vi "Main_Marvin.vi"() -> ()   [LabVIEW 2017]
uses:
  PCAN_Driver/ControlCAN.llb/DevType.ctl
  PCAN_Driver/ControlCAN.llb/CAN Channel.ctl
  PCAN_Driver/ControlCAN.llb/VCI_INIT_CONFIG.ctl
  PCAN_Driver/ControlCAN.llb/InitFlag.ctl
  PCAN_Driver/ControlCAN.llb/Fliter.ctl
  PCAN_Driver/ControlCAN.llb/Mode.ctl
  <vilib>/Utility/miscctls.llb/LVRowAndColumnTypeDef.ctl
  <vilib>/Utility/config.llb/Read Key (String).vi
  <vilib>/Utility/config.llb/Write Key (String).vi
  <vilib>/Utility/cursorutil.llb/Set Cursor (Icon Pict).vi
  PCAN_Driver/ControlCAN.lvlib
  <vilib>/Utility/config.llb/NI_LVConfig.lvlib
panel:
  in  "Index":string="5"
  out "Automation":bool
  out "ClosePanel 2":bool=TRUE
  out "ClosePanel":bool=TRUE
  out "Next SN":string
  out "Curret SN":string
  out "Array 5":dbl[](array[numeric])
  out "Array 4":dbl[](array[numeric])
  out "VC1500-2 Vel":dbl
  out "VC15100-1 Vel":dbl
  out "Array Test":T1(array[ring])
  out "TempAlg":bool=TRUE
  out "f":T2(ring)=enum."Empty"
  out "VC15100-2":dbl
  out "VC15100-1 Cur":dbl
  out "Auxiind":bool
  out "TempSensCalind":bool
  out "VisualInspectionResult":bool
  out "Burninind":bool
  out "TempControlind":bool
  out "MotorTempind":bool
  out "SpeedStopind":bool
  out "EnableTestind":bool
  out "ComTestind":bool
  out "SoftwareVer":string
  in  "SetSN":bool
  out "CurrentOffset":dbl
  out "Array 3":string[](array[string])
  out "Cal Value":string
  in  "Stop Burn-in":bool
  out "Array 2":dbl[](array[numeric])
  out "VISA resource name out":refnum<visa-resource-name>
  out "UUT":u8
  out "CAN Status":bool
  in  "Channel 2":T3 caption="Channel" items=["Channel 1", "Channel 2"]
  out "Config_CANAT":T9 {"DevType" items=["USB-CAN"=3, "USB-CAN2"=4]; "CanIndex" items=["通道1", "通道2"]; "VCI_INIT_CONFIG"."Fliter" items=["接收所有类型"=3, "只接收标准帧"=4, "只接收扩展帧"=7]; "VCI_INIT_CONFIG"."Mode" items=["正常工作", "自测模式（环回）", "仅侦听模式"]; "VCI_INIT_CONFIG"."InitFlag" items=["使用Flash参数", "使用界面设置参数"]}
  out "Array":u64[][](array[numeric]) format="%016x"
  out "Motor Phase Current RMS":dbl
  out "Ambient Temperature":dbl
  out "Speed error":bool
  out "Commutation err":bool
  out "Under voltage/Over voltage":bool
  out "Derated drive temp":bool
  out "Motor Over temperature":bool
  out "Motor Sensor temp Fauilre":bool
  out "Drive Over temperature":bool
  out "Drive Sensor temp Failure":bool
  out "Ambient Over temp":bool
  out "Ambient Sensor temp":bool
  out "DC Voltage":dbl
  out "DC Current":dbl
  out "Power transistor Heat sink Temp.":dbl
  out "Motor Stator Temp.":dbl
  out "Motor Speed RPM":dbl
  out "ECS State":u16
  out "Waveform Chart":dbl[](graph)
  out "UUT":string="EBAY"
  in  "Logger Path":path
  in  "Report":bool
  in  "Start":bool
  in  "ATR":string[][](table)=[["Test Communication", "-", "-", "-", "-", ""], ["Set S/N", "-", "-", "-", "-", ""], ["Set Board Number", "-", "-", "-", "-", ""], [" ", "", "", "", "", ""], ["Test Communication", "-", "-", "-", "-", ""], ["Get S/N", "-", "-", "-", "", ""], ["Get Board Number", "-", "-", "-", "", ""], ["Get FW", "-", "-", "-", "", ""], ["Enable Motor", "", "", "", "", ""], ["Small position command", "", "", "", "", ""], ["Measure delta", "", "", "", "", ""], ["Velocity command", "", "", "", "", ""]]
  in  "Settings":bool
  in  "Refresh Button":bool
  out "Serial":bool
  in  "VISA resource name":refnum<visa-resource-name>="COM6"
  in  "Serial Com":bool
  in  "Help Button":bool
  out "Pannel User Message":string
  in  "Stop Button":bool
  # "Marvin"
  # "REDLER TECHNOLOGIES LTD"
  # "ver 1.2g"
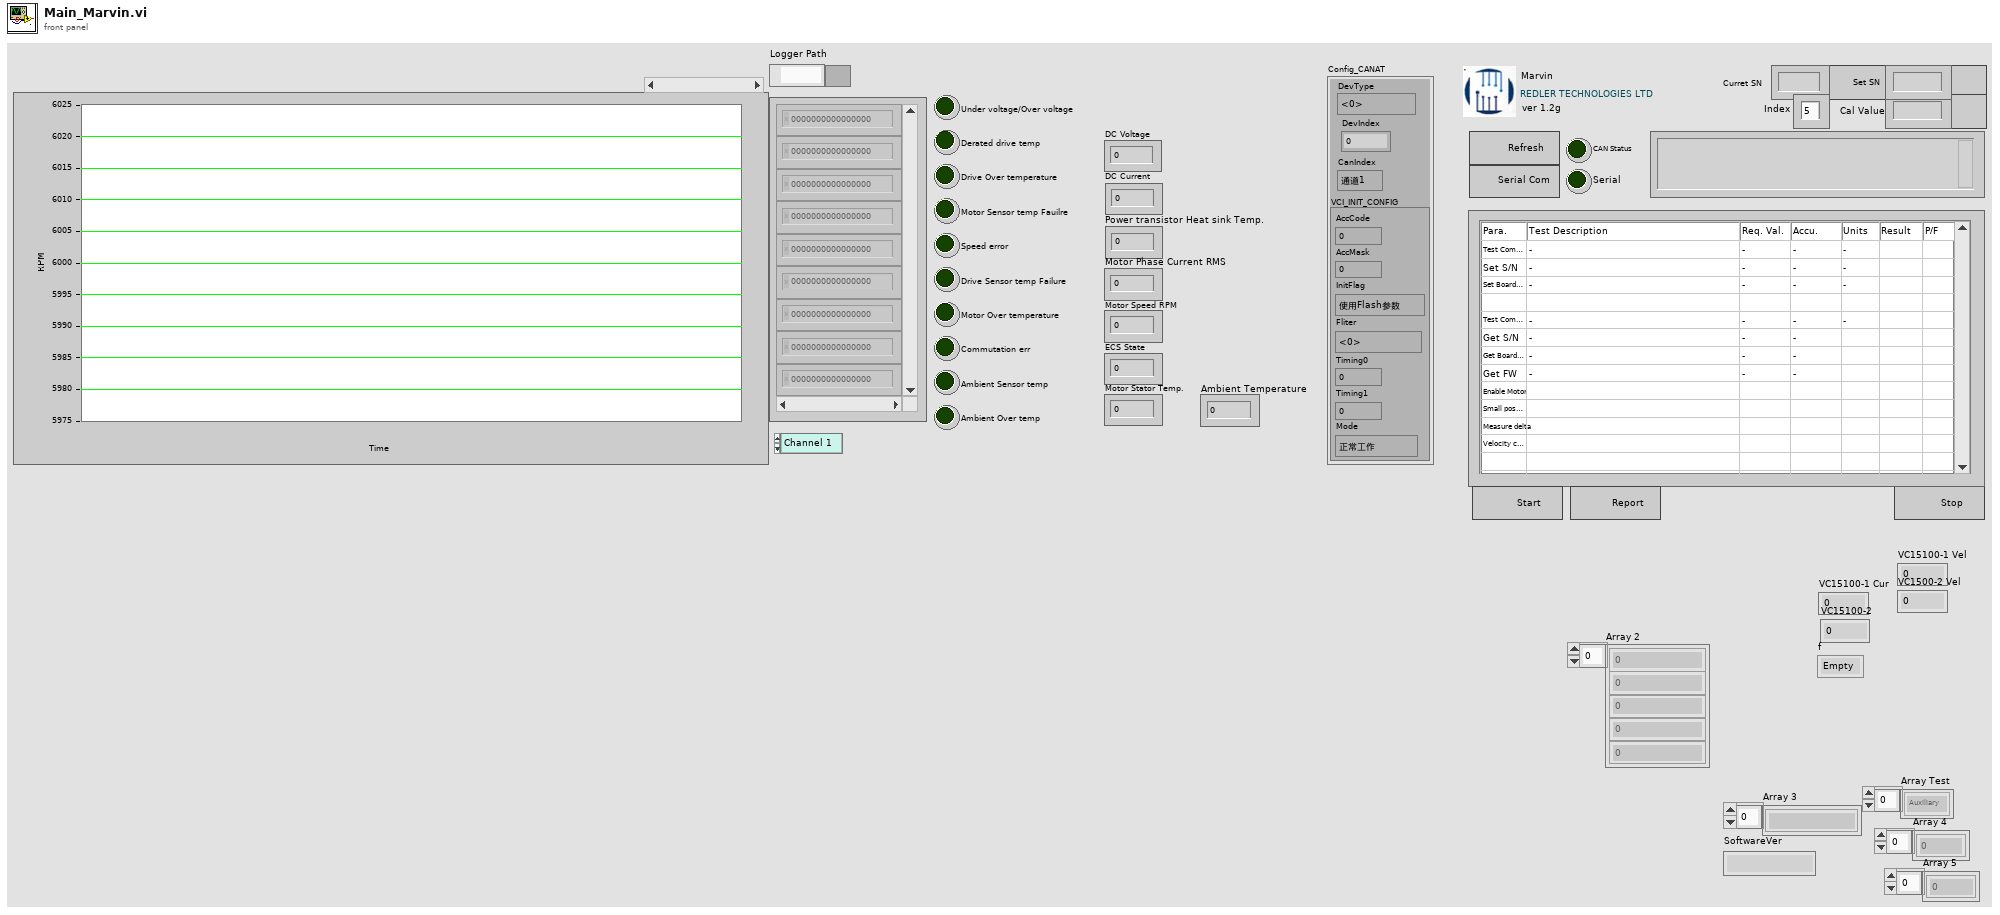
[diagram p1: front panel]
types:
  T1 = enum16{"Auxiliary", "Temp Sens Cal", "Com Test", "Enable Test", "Speed Command", "Stop Time", "Temp Control", "Burn in", "Visual Inspec", "Empty"}[]
  T2 = enum16{"Auxiliary", "Temp Sens Cal", "Com Test", "Enable Test", "Speed Command", "Stop Time", "Temp Control", "Burn in", "Visual Inspec", "Empty"}
  T3 = typedef "ControlCAN.lvlib/CAN Channel.ctl" = u32
  T4 = typedef "ControlCAN.lvlib/DevType.ctl" = u32
  T5 = typedef "ControlCAN.lvlib/VCI_INIT_CONFIG.ctl" = cluster{"AccCode":u32, "AccMask":u32, "InitFlag":T6, "Fliter":T7, "Timing0":u8, "Timing1":u8, "Mode":T8}
  T6 = typedef "ControlCAN.lvlib/InitFlag.ctl" = u32
  T7 = typedef "ControlCAN.lvlib/Fliter.ctl" = u8
  T8 = typedef "ControlCAN.lvlib/Mode.ctl" = u8
  T9 = cluster{"DevType":T4, "DevIndex":u32, "CanIndex":T3, "VCI_INIT_CONFIG":T5}
  T10 = cluster{"VISA":refnum<visa-resource-name>, "Array Test":enum16{"Auxiliary", "Temp Sens Cal", "Com Test", "Enable Test", "Speed Command", "Stop Time", "Temp Control", "Burn in", "Visual Inspec", "Empty"}[]}
  T11 = cluster{"ID":u32, "MSGTYPE":u8, "LEN":u8, "aDATA":u8[]}[]
  T12 = enum16{"Erase ATR Table", "Stop", "MainProgram", "Initialize"}
  T13 = enum8{"Enabled", "Disabled", "Disabled and Grayed Out"}
  T14 = cluster{"ID":u32, "MSGTYPE":u8, "LEN":u8, "aDATA":u8[]}
  T15 = typedef "NI_LVConfig.lvlib/Config Data RefNum.ctl" = refnum<k1>
  T16 = enum16{"STOP", "VC15100-2", "RESET", "VC15100-1", "MD0"}
  T17 = typedef "LVRowAndColumnTypeDef.ctl" = cluster{"Row":i32, "Column":i32}
  T18 = enum32{"Invalid", "Standard", "Closed", "Hidden", "Minimized", "Maximized"}
  T19 = enum16{"End", "Start", "Verify VR", "Verify UUT"}
  T20 = enum16{"open", "replace", "create", "open or create", "replace or create", "replace or create with confirmation"}
  T21 = typedef "ControlCAN.lvlib/VCI_CAN_OBJ.ctl" = cluster{"ID":u32, "TimeStamp":u32, "TimeFlag":u8, "SendType":u8, "RemoteFlag":u8, "ExternFlag":u8, "DataLen":u8, "Data":u8[], "Reserved":u8[]}
  T22 = cluster{"Type":enum16{"接收", "发送"}, "Channel":T3, "Time":timestamp, "VCI_CAN_OBJ":T21}[]
  T23 = cluster{"Type":enum16{"接收", "发送"}, "Channel":T3, "Time":timestamp, "VCI_CAN_OBJ":T21}
  T24 = typedef "LVPoint32TypeDef.ctl" = cluster{"Horizontal":i32, "Vertical":i32}
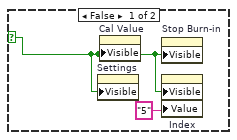
[diagram p3: hidden frame]
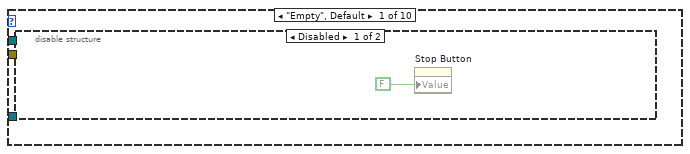
[diagram p6: hidden frame]
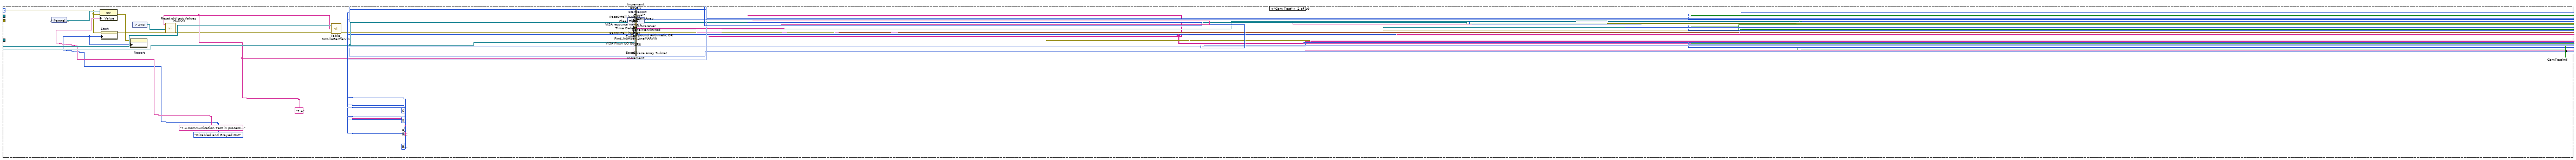
[diagram p8: hidden frame]
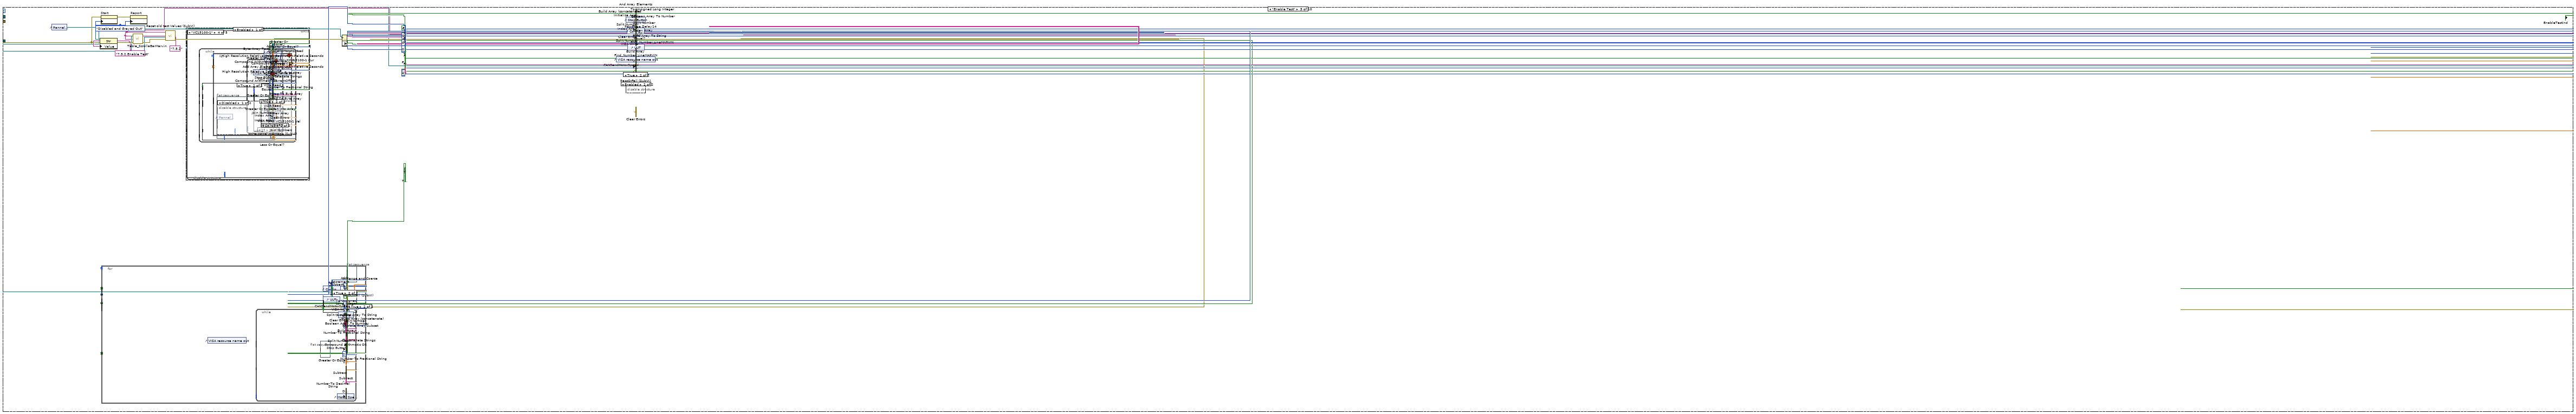
[diagram p9: hidden frame]
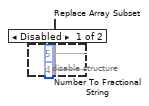
[diagram p11: hidden frame]
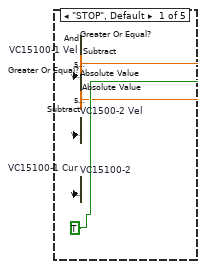
[diagram p12: hidden frame]
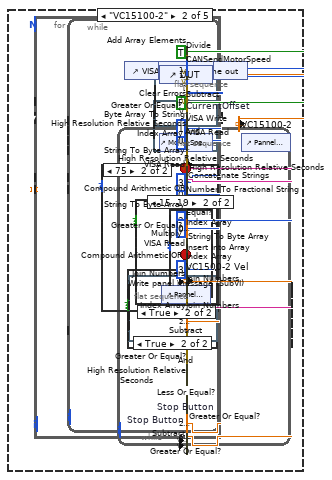
[diagram p13: hidden frame]
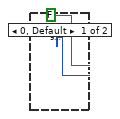
[diagram p14: hidden frame]
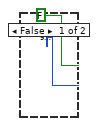
[diagram p15: hidden frame]
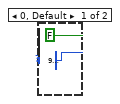
[diagram p16: hidden frame]
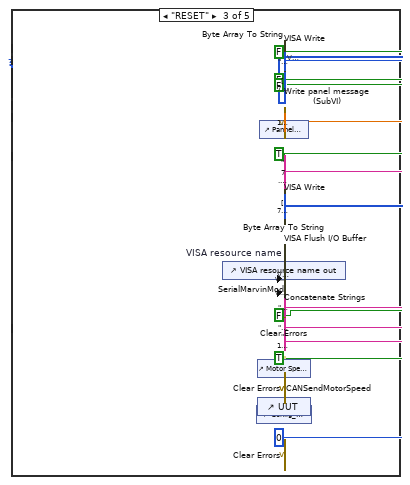
[diagram p18: hidden frame]
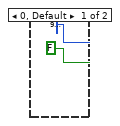
[diagram p19: hidden frame]
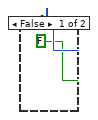
[diagram p20: hidden frame]
diagram:
  w1 = FALSE ("ClosePanel")
  w2 = "0" ("Next SN")
  w7 = 0.0 ("Val")
  (unwired) "[Marvin]\nEBAY Software Version = \"5.3.9\"\nAHU Software Version = \"5.3.8d\"\nEBAY Serial Number = \"0\"\nAHU Serial Number = \"0\""
  w21 = errorcluster {"status"=FALSE, "code"=0, "source"=""} ("error in (no error)")
  n1 = disable-structure shown="Disabled" {
    frame Disabled {
      n2 = case shown="\" float\"" {
        selector: _ -> [_ _]
        tunnel: [u32 0 ("Data I") w30] -> _
        frame "Int", Default {
        }
        frame " float" {
          n3 = To Single Precision Float(number=sgl 0.0 ("Data F")) -> (single precision float=w32:sgl)
          n4 = call "Int_Float.vi"("1 Float in"=w32) -> ("1 Int out"=w31:i32)  [unwired: 1 in, 1 out]
          n5 = To Unsigned Long Integer(number=w31) -> (unsigned 32bit integer=w30:u32)
        }
      }
    }
    frame Enabled {
    }
  }
  n6 = disable-structure shown="Disabled" {
    frame Disabled {
    }
    frame Enabled {
    }
  }
  n7 = disable-structure shown="Disabled" {
    frame Disabled {
      w35 = T13."Disabled and Grayed Out" ("Disabled")
      w36 = T13."Enabled" ("Disabled")
      n8 = control-ref of="Stop Button"() -> ()  [unwired: 1 out]
      n9 = control-ref of="Config_CANAT"() -> ()  [unwired: 1 out]
      n10 = control-ref of="UUT"() -> ()  [unwired: 1 out]
      n11 = control-ref of="Motor Speed RPM"() -> ()  [unwired: 1 out]
      n12 = control-ref of="Pannel User Message"() -> ()  [unwired: 1 out]
      n13 = control-ref of="ATR"() -> (w33:refnum<vi>)
      n14 = call "Reset old test Values (SubVI).vi"("Atr in"=w33) -> ()  [unwired: 10 in, 1 out]
      n15 = property on="Stop Button" class="Bool (strict)" props=["Value"]() -> ()  [unwired: 2 in, 3 out]
      n16 = property on="Start" class="Bool (strict)"("DisabledEnum"=w35) -> (error out=w34:errorcluster)  [unwired: 2 in, 1 out]
      n17 = property on="Start" class="Bool (strict)"("DisabledEnum"=w36) -> (error out=w37:errorcluster)  [unwired: 2 in, 1 out]
      n18 = property on="Report" class="Bool (strict)"(error in=w34, "DisabledEnum"=w35) -> ()  [unwired: 1 in, 2 out]
      n19 = property on="Report" class="Bool (strict)"(error in=w37, "DisabledEnum"=w36) -> ()  [unwired: 1 in, 2 out]
    }
    frame Enabled {
    }
  }
  n20 = disable-structure shown="Disabled" {
    frame Disabled {
      n21 = control-ref of="Pannel User Message"() -> (w38:refnum<vi>)
      n22 = call "Write panel message (SubVI).vi"("Time to wait"=30.0, "String in"=w38) -> ()  [unwired: 9 in, 1 out]
    }
    frame Enabled {
    }
  }
  n23 = disable-structure shown="Disabled" {
    frame Disabled {
      (unwired) 0.5 ("Delay Time (sec)")
      n24 = call <vilib>:"Unset Busy.vi"() -> ()  [unwired: 11 in, 1 out]
      n25 = call <vilib>:"Set Busy.vi"() -> ()  [unwired: 10 in, 2 out]
      n26 = call "Wait_Sec.vi"() -> ()  [unwired: 4 in, 1 out]
      n27 = call <vilib>:"Clear Errors.vi"() -> ()  [unwired: 6 in, 2 out]
    }
    frame Enabled {
    }
  }
  n28 = disable-structure shown="Disabled" {
    frame Disabled {
      (unwired) 5 ("disabled index (col)")
      (unwired) 3 ("index (row)")
      (unwired) 4 ("disabled index (col)")
      (unwired) 3 ("index (row)")
      n29 = property class="Tbl (strict)"() -> (reference out=w42:refnum<vi>, error out=w43:errorcluster, "Value"=w45:string[][])  [unwired: 2 in]
      n30 = Replace Array Subset(array=w45) -> (w44:string[][])  [unwired: 3 in]
      n31 = property class="Tbl (strict)"(reference=w42, error in=w43, "Value"=w44) -> (reference out=w40:refnum<vi>, error out=w41:errorcluster)
      n32 = call "PassOrFail (SubVI).vi"("error in (no error)"=w41, "Table in"=w40) -> ()  [unwired: 9 in, 1 out]
    }
    frame Enabled {
    }
  }
  n33 = control-ref of="ATR"() -> (w20:refnum<vi>)
  n34 = Obtain Queue(name (unnamed)="Test", element data type=T10 {"VISA"="COM1", "Array Test"=[]}, error in (no error)=w21) -> (queue out=w19:refnum<queue>)  [unwired: 2 in, 2 out]
  n35 = Obtain Queue(name (unnamed)="CAN RX Data", element data type=T11 [], error in (no error)=w21) -> (queue out=w23:refnum<queue>, error out=w13:errorcluster)  [unwired: 2 in, 1 out]
  n36 = while {
    tunnel: [w52] -> w9
    tunnel: [w48] -> w8
    tunnel: [w49] -> w6
    stop <- w52 stop-if-true
    n37 = call "Operator Name"() -> ("Operator Name"=w48:string, "OK"=w53:bool)  [unwired: 17 in, 1 out]
    n38 = Not Equal?(x=w48, y="") -> (x != y?=w54:bool)
    n39 = Equal?(x="nissim", y=w48) -> (x = y?=w46:bool)
    n40 = Equal?(x="admin", y=w48) -> (x = y?=w50:bool)
    n41 = And(x=w53, y=w54) -> (x .and. y?=w52:bool)
    n42 = Or(x=w46, y=w50) -> (x .or. y?=w49:bool)
  }
  n43 = while {
    shift-right: [w76] -> _
    shift-left: w23 -> [w78]
    shift-right: [w74] -> _
    shift-left: _ -> [w75]
    shift-right: [w71] -> _
    shift-left: _ -> [w70]
    shift-right: [w68] -> _
    shift-left: w13 -> [w68]
    shift-right: [w67] -> _
    shift-left: w7 -> [w61]
    shift-right: [w60] -> _
    shift-left: w7 -> [w66]
    shift-right: [w57] -> _
    shift-left: w7 -> [w65]
    shift-right: [w59] -> _
    shift-left: w7 -> [w64]
    shift-right: [w56] -> _
    shift-left: w7 -> [w63]
    shift-right: [w58] -> _
    shift-left: w7 -> [w62]
    stop <- w77 stop-if-true
    n44 = Dequeue Element(queue=w78, error in (no error)=w68) -> (queue out=w76:refnum<queue>, element=w69:T11, error out=w77:errorcluster)  [unwired: 1 in, 1 out]
    n45 = for {
      tunnel: [w245] -> w73 mode=indexing
      tunnel: w69 -> [w244] mode=indexing
      tunnel: [w243] -> w72 mode=indexing
      n46 = Unbundle By Name(w244) -> ("aDATA"=w243:u8[])
      n47 = call "Array Data to Single Num in Hex.vi"("aDATA"=w243) -> ("Numeric"=w245:u64)  [unwired: 10 in]
    }
    n48 = Build Array (concatenate)(w73, w75) -> (w74:u64[][])
    "Array" <- w74
    n49 = for {
      tunnel: w72 -> [w95] mode=indexing
      tunnel: [w93] -> w71
      tunnel: w70 -> [w92]
      tunnel: w69 -> [w91]
      shift-right: [w90] -> w67
      shift-left: w61 -> [w89]
      shift-right: [w84] -> w58
      shift-left: w62 -> [w83]
      shift-right: [w88] -> w60
      shift-left: w66 -> [w87]
      shift-right: [w86] -> w59
      shift-left: w64 -> [w85]
      shift-right: [w79] -> w56
      shift-left: w63 -> [w80]
      shift-right: [w82] -> w57
      shift-left: w65 -> [w81]
      i -> [w94]
      n50 = case shown="0, Default" w94 {
        tunnel: w95 -> [w156 w198 w238]
        tunnel: [w132 w193 w233] -> w93
        tunnel: w92 -> [w133 w193 w233]
        tunnel: w91 -> [w131 _ _]
        tunnel: [w117 w186 w226] -> w90
        tunnel: [w100 w185 w225] -> w88
        tunnel: [w99 w183 w224] -> w86
        tunnel: w89 -> [w120 w186 w226]
        tunnel: w87 -> [w103 w185 w225]
        tunnel: w85 -> [w98 w183 w224]
        tunnel: [w116 w184 w218] -> w84
        tunnel: w83 -> [w116 w184 w219]
        tunnel: [w113 w181 w222] -> w82
        tunnel: w81 -> [w112 w181 w222]
        tunnel: w80 -> [w109 w182 w223]
        tunnel: [w108 w182 w223] -> w79
        frame 0, Default {
          # "Frame ID\n0x18E1273F"
          n51 = Index Array(array=w156, index #1=0 ("index"), index #2=1 ("index"), index #3=2 ("index"), index #4=3 ("index"), index #5=4 ("index"), index #6=5 ("index"), index #7=6 ("index"), index #8=7 ("index")) -> (element #1=w140:u8, element #2=w142:u8, element #3=w143:u8, element #4=w147:u8, element #5=w150:u8, element #6=w154:u8, element #7=w155:u8, element #8=w153:u8)
          n52 = Number To Hexadecimal String(2:w153) -> (0:w166:string)  [unwired: 1 in]
          n53 = Join Numbers(hi=w155, lo=w154) -> ((hi.lo)=w172:u16)
          n54 = Join Numbers(hi=w143, lo=w142) -> ((hi.lo)=w144:u16)
          n55 = Number To Hexadecimal String(2:w150) -> (0:w151:string)  [unwired: 1 in]
          n56 = Number To Hexadecimal String(2:w172) -> (0:w171:string)  [unwired: 1 in]
          n57 = Number To Hexadecimal String(2:w140) -> (0:w141:string)  [unwired: 1 in]
          n58 = Number To Hexadecimal String(2:w144) -> (0:w145:string)  [unwired: 1 in]
          n59 = Number To Hexadecimal String(2:w147) -> (0:w148:string)  [unwired: 1 in]
          n60 = Hexadecimal String To Number(string=w166) -> (number=w165:u32)  [unwired: 2 in, 1 out]
          n61 = Index Array(array=w131, index=0) -> (element=w129:T14)
          n62 = To Double Precision Float(number=w165) -> (double precision float=w115:dbl)
          n63 = Unbundle By Name(w129) -> ("ID"=w122:u32)
          n64 = Hexadecimal String To Number(string=w151) -> (number=w152:u32)  [unwired: 2 in, 1 out]
          n65 = Hexadecimal String To Number(string=w171) -> (number=w170:u32)  [unwired: 2 in, 1 out]
          n66 = Hexadecimal String To Number(string=w141) -> (number=w138:u32)  [unwired: 2 in, 1 out]
          n67 = Hexadecimal String To Number(string=w145) -> (number=w146:u32)  [unwired: 2 in, 1 out]
          n68 = Hexadecimal String To Number(string=w148) -> (number=w149:u32)  [unwired: 2 in, 1 out]
          n69 = To Double Precision Float(number=w170) -> (double precision float=w167:dbl)
          n70 = To Double Precision Float(number=w152) -> (double precision float=w135:dbl)
          n71 = To Double Precision Float(number=w146) -> (double precision float=w119:dbl)
          n72 = To Double Precision Float(number=w149) -> (double precision float=w137:dbl)
          n73 = To Unsigned Word Integer(number=w138) -> (unsigned 16bit integer=→"ECS State":u16)
          n74 = To Double Precision Float(number=u32 10 ("y")) -> (double precision float=w168:dbl)
          n75 = Subtract(x=w135, y=50.0 ("x")) -> (x-y=w106:dbl)
          n76 = Subtract(x=w137, y=50.0 ("x")) -> (x-y=w104:dbl)
          n77 = Divide(x=w167, y=w168) -> (x/y=w111:dbl)
          n78 = Less Than 0?(x=w104) -> (x < 0?=w105:bool)
          n79 = Equal?(x=u32 417408815, y=w122) -> (x = y?=w123:bool)
          n80 = Equal?(x=u32 417408831, y=w122) -> (x = y?=w125:bool)
          n81 = Equal?(x=u32 417408863, y=w122) -> (x = y?=w124:bool)
          n82 = Less Than 0?(x=w106) -> (x < 0?=w107:bool)
          n83 = call "Filter (SubVI).vi"("Delta"=5000.0, "NewVal"=w119, "OldVal"=w120) -> ("Val"=w117:dbl)  [unwired: 8 in]
          "Motor Speed RPM" <- w117
          n84 = Select(t=w103, s=w105, f=w104) -> (s? t:f=w102:dbl)
          n85 = Select(t=w98, s=w107, f=w106) -> (s? t:f=w97:dbl)
          n86 = Compound Arithmetic op=OR(w125, w124, w123) -> (w121:bool)
          n87 = call "Filter (SubVI).vi"("Delta"=130.0, "NewVal"=w102, "OldVal"=w103) -> ("Val"=w100:dbl)  [unwired: 8 in]
          "Motor Stator Temp." <- w100
          n88 = call "Filter (SubVI).vi"("Delta"=100.0, "NewVal"=w97, "OldVal"=w98) -> ("Val"=w99:dbl)  [unwired: 8 in]
          "Power transistor Heat sink Temp." <- w99
          n89 = call "Filter (SubVI).vi"("Delta"=15.0, "NewVal"=w111, "OldVal"=w109) -> ("Val"=w108:dbl)  [unwired: 8 in]
          "DC Voltage" <- w108
          n90 = call "Filter (SubVI).vi"("Delta"=15.0, "NewVal"=w115, "OldVal"=w112) -> ("Val"=w113:dbl)  [unwired: 8 in]
          "DC Current" <- w113
          n91 = case shown="True" w121 {
            tunnel: w133 -> [w173 w176]
            tunnel: [w173 w175] -> w132
            tunnel: w119 -> [_ w174]
            frame False {
            }
            frame True {
              n92 = disable-structure shown="Disabled" {
                disable-tunnel: w174 -> [w180 _]
                frame Disabled {
                  n93 = call <vilib>:"Application Directory.vi"() -> ("Application Directory"=w178:path)
                  n94 = Build Path(base path=w178, name or relative path="RPM Log.lvm") -> (appended path=w179:path)
                  n95 = call "Write To Measurement File"("Signals"=w180, "Filename"=w179) -> ()  [unwired: 15 in, 3 out]
                }
                frame Enabled {
                }
              }
              n96 = Build Array (concatenate)(w174, w176) -> (w175:dbl[])
              "Waveform Chart" <- w175
            }
          }
        }
        frame 1 {
          # "Framde ID\n0x18E3273F"
          n97 = control-ref of="UUT"() -> (w187:refnum<vi>)
          n98 = property on="Property Node" class="DigNum (strict)"(reference=w187) -> ("Value"=w188:u8)  [unwired: 1 in, 2 out]
          n99 = Index Array(array=w198, index #1=0 ("index"), index #2=1 ("index")) -> (element #1=w196:u8, element #2=w190:u8)
          n100 = Number To Boolean Array(number=w196) -> (Boolean array=w195:bool[])
          n101 = Number To Boolean Array(number=w190) -> (Boolean array=w192:bool[])
          n102 = Boolean To (0,1)(Boolean=w192) -> (0, 1=w189:i16[])
          n103 = Boolean To (0,1)(Boolean=w195) -> (0, 1=w194:i16[])
          n104 = case shown="95" w188 {
            tunnel: w189 -> [_ w199]
            frame 0, Default {
            }
            frame 95 {
              n105 = for {
                tunnel: w199 -> [w204] mode=indexing
                i -> [w200]
                stop <- w202 stop-if-true
                n106 = Not Equal To 0?(x=w204) -> (x != 0?=w203:bool)
                n107 = case shown="0, Default" w200 {
                  tunnel: w203 -> [w205 w206]
                  frame 0, Default {
                    "Ambient Sensor temp" <- w205
                  }
                  frame 1 {
                    "Ambient Over temp" <- w206
                  }
                }
                n108 = Equal?(x=w200, y=1.0) -> (x = y?=w202:bool)
              }
            }
          }
          n109 = for {
            tunnel: w194 -> [w208] mode=indexing
            i -> [w209]
            n110 = Not Equal To 0?(x=w208) -> (x != 0?=w207:bool)
            n111 = case shown="2" w209 {
              tunnel: w207 -> [w210 w211 w212 w213 w214 w215 w216 w217]
              frame 0, Default {
                "Drive Sensor temp Failure" <- w210
              }
              frame 1 {
                "Drive Over temperature" <- w211
              }
              frame 2 {
                "Motor Sensor temp Fauilre" <- w212
              }
              frame 3 {
                "Motor Over temperature" <- w213
              }
              frame 4 {
                "Derated drive temp" <- w214
              }
              frame 5 {
                "Under voltage/Over voltage" <- w215
              }
              frame 6 {
                "Commutation err" <- w216
              }
              frame 7 {
                "Speed error" <- w217
              }
            }
          }
        }
        frame 2 {
          # "Frame ID\n0x18E2273F"
          n112 = Index Array(array=w238, index #1=0 ("index"), index #2=1 ("index")) -> (element #1=w235:u8, element #2=w231:u8)
          n113 = disable-structure shown="Enabled" {
            disable-tunnel: [w241 w242] -> w236
            disable-tunnel: w235 -> [w240 w242]
            frame Disabled {
              n114 = Number To Hexadecimal String(2:w240) -> (0:w239:string)  [unwired: 1 in]
              n115 = Hexadecimal String To Number(string=w239) -> (number=w241:u32)  [unwired: 2 in, 1 out]
            }
            frame Enabled {
            }
          }
          n116 = Number To Hexadecimal String(2:w231) -> (0:w229:string)  [unwired: 1 in]
          n117 = Hexadecimal String To Number(string=w229) -> (number=w230:u32)  [unwired: 2 in, 1 out]
          n118 = To Double Precision Float(number=w230) -> (double precision float=w228:dbl)
          n119 = To Double Precision Float(number=w236) -> (double precision float=→"Motor Phase Current RMS":dbl)
          n120 = Subtract(x=w228, y=50.0) -> (x-y=w220:dbl)
          n121 = Less Than 0?(x=w220) -> (x < 0?=w221:bool)
          n122 = Select(t=w219, s=w221, f=w220) -> (s? t:f=w218:dbl)
          "Ambient Temperature" <- w218
        }
      }
    }
  }
  n123 = control-ref of="This VI"() -> (w5:refnum<vi>)
  n124 = register-events "Register For Events"(w5) -> (reference out=w4:refnum<event-registration>)  [unwired: 2 in, 1 out]
  n125 = call <vilib>:"Application Directory.vi"() -> ("Application Directory"=w16:path)
  n126 = Build Path(base path=w16, name or relative path="data\\MarvinParams.ini") -> (appended path=w10:path)
  n127 = call <vilib>:"Open Config Data.vi"("error in (no error)"=w13, "create file if necessary (T)"=FALSE, "configuration file path"=w10) -> ("error out"=w12:errorcluster, "refnum"=w11:T15)  [unwired: 7 out]
  n128 = case shown="True" w6 {
    selector: w6 -> [w247 w249]
    frame False {
      n129 = property on="Settings" class="Bool"("Visible"=w247) -> ()  [unwired: 2 in, 2 out]
      n130 = property on="Cal Value" class="Str"("Visible"=w247) -> ()  [unwired: 2 in, 2 out]
      n131 = property on="Stop Burn-in" class="Bool"("Visible"=w247) -> ()  [unwired: 2 in, 2 out]
      n132 = property on="Index" class="Str"("Visible"=w247, "Value"="5" ("Index")) -> ()  [unwired: 2 in, 2 out]
    }
    frame True {
      n133 = property on="Settings" class="Bool"("Visible"=w249) -> ()  [unwired: 2 in, 2 out]
      n134 = property on="Cal Value" class="Str"("Visible"=w249) -> ()  [unwired: 2 in, 2 out]
      n135 = property on="Index" class="Str"("Visible"=w249, "Value"="5" ("Index")) -> ()  [unwired: 2 in, 2 out]
      n136 = property on="Stop Burn-in" class="Bool"("Visible"=w249) -> ()  [unwired: 2 in, 2 out]
    }
  }
  n137 = local write "ClosePanel"(w1) -> ()
  n138 = local write "Next SN"(w2) -> ()
  n139 = while {
    tunnel: w20 -> [w258]
    tunnel: w13 -> [w256]
    tunnel: w19 -> [w257]
    stop <- w252 stop-if-true
    n140 = Dequeue Element(queue=w257, error in (no error)=w256) -> (element=w255:T10, error out=w252:errorcluster)  [unwired: 1 in, 2 out]
    n141 = Unbundle By Name(w255) -> ("VISA"=w254:refnum<visa-resource-name>, "Array Test"=w253:T1)
    n142 = for {
      tunnel: w253 -> [w263] mode=indexing
      tunnel: w254 -> [w265]
      tunnel: w258 -> [w264]
      tunnel: w252 -> [w262]
      tunnel: [w262] -> w251
      stop <- w260 stop-if-true
      n143 = case shown="\"Stop Time\"" w263 {
        tunnel: w265 -> [_ _ _ _ _ _ _ _ w1959 _]
        tunnel: w264 -> [_ w299 w318 w970 w1166 w1285 w1607 w1918 w1921 w2166]
        tunnel: w262 -> [_ w279 w334 w975 w1173 w1297 w1633 w1914 w1954 w2175]
        frame "Empty", Default {
          n144 = disable-structure shown="Disabled" {
            frame Disabled {
              n145 = property on="Stop Button" class="Bool (strict)"("Value"=FALSE ("Stop Button")) -> ()  [unwired: 2 in, 2 out]
            }
            frame Enabled {
            }
          }
        }
        frame "Com Test" {
          w276 = T13."Enabled" ("Disabled")
          w277 = T13."Disabled and Grayed Out" ("Disabled")
          w300 = 6 ("disabled index (col)")
          w269 = "7.4" ("Test Paragraph")
          n146 = control-ref of="Pannel User Message"() -> (w297:refnum<vi>)
          n147 = property class="Str"(reference=w297, error in=w279, "Value"="7.4.Communication Test in process...") -> (error out=w268:errorcluster)  [unwired: 1 out]
          n148 = property on="Start" class="Bool (strict)"(error in=w279, "DisabledEnum"=w277) -> (error out=w278:errorcluster)  [unwired: 1 in, 1 out]
          n149 = property on="Report" class="Bool (strict)"(error in=w278, "DisabledEnum"=w277) -> ()  [unwired: 1 in, 2 out]
          n150 = control-ref of="ATR"() -> (w270:refnum<vi>)
          n151 = call "Reset old test Values (SubVI).vi"("error in"=w268, "Atr in"=w270, "Test Paragraph"=w269) -> ("error out"=w267:errorcluster)  [unwired: 8 in]
          n152 = call "Table_ScrollaBarMarvin.vi"("error in"=w267, "Line to focus"=w269, "reference in"=w299) -> ("error out"=w298:errorcluster)  [unwired: 2 out]
          n153 = control-ref of="UUT"() -> (w310:refnum<vi>)
          n154 = property on="SoftwareVer" class="Str"() -> ("Value"=w283:string)  [unwired: 2 in, 2 out]
          n155 = property on="VISA resource name" class="VISAName"() -> ("Value"=w294:refnum<visa-resource-name>)  [unwired: 2 in, 2 out]
          n156 = property class="Tbl (strict)"(reference=w299, error in=w298) -> (reference out=w287:refnum<vi>, error out=w314:errorcluster, "Value"=w271:string[][])
          n157 = Index Array(array=w271, index (col)=0 ("disabled index (col)")) -> (element=w315:string[])  [unwired: 1 in]
          n158 = call "Find_Number_LineMARVIN.vi"("Test Paragraph"=w269, "error in"=w314, "Row Headers[]"=w315) -> ("error out"=w312:errorcluster, "Line number"=w311:i32)  [unwired: 2 in, 2 out]
          n159 = call <vilib>:"Clear Errors.vi"("error in (no error)"=w312) -> ("error out"=w273:errorcluster)  [unwired: 5 in, 1 out]
          n160 = call "Time Delay7"("error in (no error)"=w273) -> ("error out"=w272:errorcluster)  [unwired: 10 in]
          n161 = VISA Flush I/O Buffer(VISA resource name=w294, error in (no error)=w272) -> (VISA resource name out=w292:refnum<visa-resource-name>, error out=w293:errorcluster)  [unwired: 1 in]
          n162 = call "SerialMarvinMod.vi"("error in (no error)"=w293, "write buffer"="VR\r\n", "VISA resource name"=w292) -> ("error out"=w286:errorcluster, "read buffer"=w289:string)  [unwired: 7 in]
          n163 = Equal?(x=w283, y=w289) -> (x = y?=w281:bool)
          n164 = Increment(x=w311) -> (x+1=w291:i32)
          n165 = Increment(x=w291) -> (x+1=w302:i32)
          n166 = Replace Array Subset(array=w271, new element=w289, index (row)=w291, index (col)=5 ("disabled index (col)")) -> (w288:string[][])
          n167 = property class="Tbl (strict)"(reference=w287, error in=w286, "Value"=w288) -> (error out=w285:errorcluster)  [unwired: 1 out]
          n168 = call "PassOrFail (SubVI).vi"("disabled index (col)"=w300, "index (row)"=w291, "error in (no error)"=w285, "Boolean"=w281, "Table in"=w299) -> ("error out"=w284:errorcluster)  [unwired: 6 in]
          n169 = property class="DigNum (strict)"(reference=w310, error in=w284) -> (error out=w301:errorcluster, "Value"=w309:u8)  [unwired: 1 out]
          n170 = Equal?(x=w309, y=u8 47) -> (x = y?=w305:bool)
          n171 = Equal?(x=w309, y=u8 63) -> (x = y?=w304:bool)
          n172 = Equal?(x=w309, y=u8 95) -> (x = y?=w303:bool)
          n173 = Compound Arithmetic op=OR(w305, w304, w303) -> (w282:bool)
          n174 = call "PassOrFail (SubVI).vi"("disabled index (col)"=w300, "index (row)"=w302, "error in (no error)"=w301, "Boolean"=w282, "Table in"=w299) -> ("error out"=w274:errorcluster)  [unwired: 6 in]
          n175 = property on="Start" class="Bool (strict)"(error in=w274, "DisabledEnum"=w276) -> (error out=w275:errorcluster)  [unwired: 1 in, 1 out]
          n176 = property on="Report" class="Bool (strict)"(error in=w275, "DisabledEnum"=w276) -> ()  [unwired: 1 in, 2 out]
          n177 = And(x=w282, y=w281) -> (x .and. y?=→"ComTestind":bool)
        }
        frame "Enable Test" {
          w333 = T13."Enabled" ("Disabled")
          w336 = T13."Disabled and Grayed Out" ("Disabled")
          w317 = "7.5.2" ("Test Paragraph")
          n178 = control-ref of="Pannel User Message"() -> (w352:refnum<vi>)
          n179 = property class="Str"(reference=w352, error in=w334, "Value"="7.5.2.Enable Test") -> (error out=w351:errorcluster)  [unwired: 1 out]
          n180 = property on="Start" class="Bool (strict)"(error in=w334, "DisabledEnum"=w336) -> (error out=w335:errorcluster)  [unwired: 1 in, 1 out]
          n181 = property on="Report" class="Bool (strict)"(error in=w335, "DisabledEnum"=w336) -> ()  [unwired: 1 in, 2 out]
          n182 = call "Table_ScrollaBarMarvin.vi"("error in"=w351, "Line to focus"=w317, "reference in"=w318) -> ("error out"=w390:errorcluster)  [unwired: 2 out]
          n183 = call "Reset old test Values (SubVI).vi"("error in"=w390, "Atr in"=w318, "Test Paragraph"=w317) -> ("error out"=w319:errorcluster)  [unwired: 8 in]
          n184 = property class="Tbl (strict)"(reference=w318, error in=w319) -> (error out=w392:errorcluster, "Value"=w393:string[][])  [unwired: 1 out]
          n185 = control-ref of="VISA resource name out"() -> (w363:refnum<vi>)
          n186 = control-ref of="Stop Button"() -> (w329:refnum<vi>)
          n187 = control-ref of="Config_CANAT"() -> (w345:refnum<vi>)
          n188 = control-ref of="UUT"() -> (w346:refnum<vi>)
          n189 = Initialize Array(FALSE, 14 ("dimension size")) -> (w375:bool[])
          n190 = Build Array (concatenate)(w375, bool[] [FALSE, FALSE, FALSE, FALSE, FALSE, FALSE, FALSE] ("array")) -> (w376:bool[])
          n191 = Boolean Array To Number(Boolean array=w376) -> (number=w374:u32)
          n192 = To Unsigned Long Integer(number=w374) -> (unsigned 32bit integer=w365:u32)
          n193 = Split Number(x=w365) -> (hi(x)=w370:u16, lo(x)=w371:u16)
          n194 = Split Number(x=w371) -> (hi(x)=w369:u8, lo(x)=w368:u8)
          n195 = Index Array(array=w393, index (col)=0 ("disabled index (col)")) -> (element=w394:string[])  [unwired: 1 in]
          n196 = property on="UUT" class="Str"() -> ("Value"=w327:string)  [unwired: 2 in, 2 out]
          n197 = Equal?(x=w327, y="EBAY") -> (x = y?=w325:bool)
          n198 = case shown="True" w325 {
            tunnel: [u16 12100 ("Motor Speed RPM") u16 15100 ("Motor Speed RPM")] -> w324
            tunnel: [11200.0 ("y") 14800.0 ("y")] -> w323
            tunnel: [13000.0 ("y") 16000.0 ("y")] -> w322
            tunnel: [20.0 ("y") 48.0 ("y")] -> w321
            tunnel: [15.0 ("y") 40.0 ("y")] -> w320
            frame False {
            }
            frame True {
            }
          }
          n199 = call "Find_Number_LineMARVIN.vi"("Test Paragraph"=w317, "error in"=w392, "Row Headers[]"=w394) -> ("error out"=w328:errorcluster, "Line number"=w389:i32)  [unwired: 2 in, 2 out]
          n200 = for {
            tunnel: w318 -> [w928]
            tunnel: w389 -> [w918]
            tunnel: u16[] [5000, 0, 5000] -> [w893] mode=indexing
            tunnel: [w916] -> w387
            tunnel: w328 -> [w894]
            tunnel: bool[] [TRUE, FALSE, TRUE] -> [w892] mode=indexing
            tunnel: bool[] [TRUE, TRUE, TRUE] -> [w891] mode=indexing
            tunnel: [w890] -> w342 mode=indexing
            i -> [w920]
            w921 = 200.0 ("y")
            n201 = control-ref of="VISA resource name out"() -> (w913:refnum<vi>)
            n202 = while {
              tunnel: [w940] -> w930
              tunnel: [w957] -> w929
              tunnel: w887 -> [w956]
              tunnel: w889 -> [w954]
              stop <- w939 stop-if-true
              w951 = 15.0 ("y")
              n203 = flat-sequence {
                tunnel: [w959] -> w955
                frame #0 {
                  n204 = call <vilib>:"High Resolution Relative Seconds.vi"() -> ("relative seconds"=w959:dbl)
                }
              }
              n205 = control-ref of="Motor Speed RPM"() -> (w958:refnum<vi>)
              n206 = control-ref of="Pannel User Message"() -> (w952:refnum<vi>)
              n207 = property on="Stop Button" class="Bool (strict)"() -> ("Value"=w938:bool)  [unwired: 2 in, 2 out]
              n208 = Subtract(x=w955, y=w954) -> (x-y=w950:dbl)
              n209 = Greater Or Equal?(x=w950, y=w951) -> (x >= y?=w953:bool)
              n210 = Compound Arithmetic op=OR(w938, w953) -> (w939:bool)
              n211 = Subtract(x=w951, y=w950) -> (x-y=w942:dbl)
              n212 = Number To Fractional String(number=w942, precision (6)=i16 2) -> (F-format string=w948:string)  [unwired: 2 in]
              n213 = property class="DigNum (strict)"(reference=w958, error in=w956) -> (error out=w957:errorcluster, "Value"=w940:dbl)  [unwired: 1 out]
              n214 = Number To Decimal String(number=w940) -> (decimal integer string=w949:string)  [unwired: 1 in]
              n215 = Concatenate Strings("7.5.2.Enable Test in process...\nRemained Time: " ("string"), w948, "  sec." ("string"), "\r\n", "Motor speed [rpm]: " ("string"), w949) -> (w943:string)
              n216 = property class="Str"(reference=w952, "Value"=w943) -> ()  [unwired: 1 in, 2 out]
            }
            n217 = control-ref of="Config_CANAT"() -> (w935:refnum<vi>)
            n218 = Subtract(x=w893, y=w921) -> (x-y=w922:dbl)
            n219 = flat-sequence {
              tunnel: [w937] -> w889
              tunnel: w888 -> [w936]
              tunnel: [w936] -> w887
              frame #0 {
                n220 = call <vilib>:"High Resolution Relative Seconds.vi"() -> ("relative seconds"=w937:dbl)
              }
            }
            n221 = Add(x=w893, y=w921) -> (x+y=w923:dbl)
            n222 = In Range and Coerce(upper limit=w923, x=w930, lower limit=w922) -> (In Range?=w890:bool)  [unwired: 1 out]
            n223 = Increment(x=w920) -> (x+1=w919:i32)
            n224 = Add(x=w918, y=w919) -> (x+y=w915:i32)
            n225 = case shown="True" w892 {
              tunnel: [bool[] [FALSE, FALSE, FALSE, FALSE, FALSE, FALSE, FALSE] ("array") bool[] [FALSE, FALSE, FALSE, TRUE, FALSE, FALSE, FALSE] ("array")] -> w900
              frame False {
              }
              frame True {
              }
            }
            n226 = call <vilib>:"Clear Errors.vi"("error in (no error)"=w929) -> ("error out"=w886:errorcluster)  [unwired: 5 in, 1 out]
            n227 = call "PassOrFail (SubVI).vi"("disabled index (col)"=6, "index (row)"=w915, "error in (no error)"=w886, "Boolean"=w890, "Table in"=w928) -> ("error out"=w932:errorcluster)  [unwired: 6 in]
            n228 = property class="Tbl (strict)"(reference=w928, error in=w932) -> (reference out=w924:refnum<vi>, error out=w933:errorcluster, "Value"=w925:string[][])
            n229 = Build Array (concatenate)(bool[] [FALSE, FALSE, FALSE, TRUE, FALSE, FALSE, FALSE, FALSE, FALSE, FALSE, FALSE, FALSE, FALSE, FALSE] ("array"), w900) -> (w901:bool[])
            n230 = Boolean Array To Number(Boolean array=w901) -> (number=w902:u32)
            n231 = To Unsigned Long Integer(number=w902) -> (unsigned 32bit integer=w911:u32)
            n232 = Split Number(x=w911) -> (hi(x)=w906:u16, lo(x)=w905:u16)
            n233 = Split Number(x=w905) -> (hi(x)=w907:u8, lo(x)=w908:u8)
            n234 = Number To Fractional String(number=w930, precision (6)=i16 2) -> (F-format string=w927:string)  [unwired: 2 in]
            n235 = Replace Array Subset(array=w925, new element=w927, index (row)=w915, index (col)=5 ("disabled index (col)")) -> (w926:string[][])
            n236 = property class="Tbl (strict)"(reference=w924, error in=w933, "Value"=w926) -> (error out=w916:errorcluster)  [unwired: 1 out]
            n237 = property class="VISAName"(reference=w913, error in=w894) -> (error out=w914:errorcluster, "Value"=w904:refnum<visa-resource-name>)  [unwired: 1 out]
            n238 = Split Number(x=w906) -> (hi(x)=w909:u8, lo(x)=w910:u8)
            n239 = Build Array(u8 75, u8 0 ("element"), u8 4 ("Length"), u8 2, w908, w907, w910, w909) -> (w903:u8[])
            n240 = Byte Array To String(unsigned byte array=w903) -> (string=w912:string)
            n241 = VISA Write(VISA resource name=w904, write buffer=w912, error in (no error)=w914) -> (error out=w895:errorcluster)  [unwired: 2 out]
            n242 = case shown="True" w891 {
              tunnel: w935 -> [_ w965]
              tunnel: [w960 w964] -> w888
              tunnel: w895 -> [w960 w962]
              frame False {
              }
              frame True {
                n243 = control-ref of="UUT"() -> (w966:refnum<vi>)
                n244 = call "CANSendMotorSpeed.vi"("Remote"=TRUE, "error in (no error)"=w962, "Motor Speed RPM"=u16 5000, "UUT"=w966, "Cluster in"=w965) -> ("error out"=w964:errorcluster)  [unwired: 6 in]
              }
            }
          }
          n245 = And Array Elements(Boolean array=w342) -> (logical AND=w341:bool)
          n246 = Split Number(x=w370) -> (hi(x)=w367:u8, lo(x)=w366:u8)
          n247 = Build Array(u8 75, u8 0 ("element"), u8 4 ("Length"), u8 2, w368, w369, w366, w367) -> (w373:u8[])
          n248 = Byte Array To String(unsigned byte array=w373) -> (string=w364:string)
          n249 = call <vilib>:"Clear Errors.vi"("error in (no error)"=w387) -> ("error out"=w338:errorcluster)  [unwired: 5 in, 1 out]
          n250 = disable-structure shown="Enabled" {
            disable-tunnel: w338 -> [w427 w883]
            disable-tunnel: [w426 w882] -> w344
            disable-tunnel: [w425 w884] -> w340
            disable-tunnel: T16."MD0" -> [w424 _]
            disable-tunnel: w329 -> [w423 _]
            disable-tunnel: w324 -> [w422 _]
            disable-tunnel: w323 -> [w421 _]
            disable-tunnel: w322 -> [w420 _]
            disable-tunnel: w321 -> [w419 _]
            disable-tunnel: w320 -> [w418 _]
            frame Enabled {
              n251 = while {
                tunnel: [w439] -> w425
                tunnel: w427 -> [w441]
                tunnel: [w440] -> w426
                shift-right: [w437] -> _
                shift-left: w424 -> [w438]
                tunnel: w423 -> [w433]
                tunnel: w422 -> [w432]
                tunnel: w421 -> [w431]
                tunnel: w420 -> [w430]
                tunnel: w419 -> [w429]
                tunnel: w418 -> [w428]
                stop <- w435 stop-if-true
                n252 = case shown="\"VC15100-1\"" w438 {
                  selector: w438 -> [w455 _ _ _ _]
                  tunnel: w441 -> [w456 w484 w638 w678 w844]
                  tunnel: [w456 w477 w644 w672 w843] -> w440
                  tunnel: [w448 FALSE FALSE FALSE FALSE] -> w439
                  tunnel: [w455 T16."STOP" T16."VC15100-2" w664 w847] -> w437
                  tunnel: [TRUE FALSE FALSE FALSE FALSE] -> w436
                  tunnel: w433 -> [_ w463 w622 w658 w838]
                  tunnel: w432 -> [_ w462 _ _ _]
                  tunnel: w431 -> [_ w461 _ _ _]
                  tunnel: w430 -> [_ w460 _ _ _]
                  tunnel: w429 -> [_ w459 _ w656 _]
                  tunnel: w428 -> [_ w458 _ w657 _]
                  frame "STOP", Default {
                    n253 = property on="VC15100-1 Vel" class="DigNum (strict)"() -> ("Value"=w447:dbl)  [unwired: 2 in, 2 out]
                    n254 = property on="VC1500-2 Vel" class="DigNum (strict)"() -> ("Value"=w446:dbl)  [unwired: 2 in, 2 out]
                    n255 = Subtract(x=w447, y=w446) -> (x-y=w445:dbl)
                    n256 = Absolute Value(x=w445) -> (abs(x)=w444:dbl)
                    n257 = Greater Or Equal?(x=w444, y=500.0) -> (x >= y?=w442:bool)
                    n258 = property on="VC15100-2" class="DigNum (strict)"() -> ("Value"=w454:dbl)  [unwired: 2 in, 2 out]
                    n259 = property on="VC15100-1 Cur" class="DigNum (strict)"() -> ("Value"=w453:dbl)  [unwired: 2 in, 2 out]
                    n260 = Subtract(x=w454, y=w453) -> (x-y=w450:dbl)
                    n261 = Absolute Value(x=w450) -> (abs(x)=w449:dbl)
                    n262 = Greater Or Equal?(x=w449, y=5.0) -> (x >= y?=w451:bool)
                    n263 = And(x=w442, y=w451) -> (x .and. y?=w448:bool)
                  }
                  frame "VC15100-2" {
                    n264 = control-ref of="VISA resource name out"() -> (w479:refnum<vi>)
                    n265 = flat-sequence {
                      tunnel: [w578] -> w483
                      tunnel: w482 -> [w577]
                      tunnel: [w577] -> w481
                      frame #0 {
                        n266 = call <vilib>:"High Resolution Relative Seconds.vi"() -> ("relative seconds"=w578:dbl)
                      }
                    }
                    n267 = control-ref of="Config_CANAT"() -> (w486:refnum<vi>)
                    n268 = control-ref of="UUT"() -> (w485:refnum<vi>)
                    n269 = call <vilib>:"Clear Errors.vi"("error in (no error)"=w481) -> ("error out"=w471:errorcluster)  [unwired: 5 in, 1 out]
                    n270 = while {
                      tunnel: w483 -> [w602]
                      tunnel: w471 -> [w596]
                      tunnel: [w597] -> w478
                      tunnel: [w595] -> w476
                      tunnel: w463 -> [w583]
                      tunnel: w461 -> [w580]
                      tunnel: w460 -> [w579]
                      stop <- w600 stop-if-true
                      w581 = "7.5.2.4.Motor rotation direction test in process..." ("string")
                      n271 = control-ref of="Motor Speed RPM"() -> (w582:refnum<vi>)
                      n272 = property class="DigNum (strict)"(reference=w582, error in=w596) -> (error out=w597:errorcluster, "Value"=w586:dbl)  [unwired: 1 out]
                      "VC1500-2 Vel" <- w586
                      n273 = Number To Fractional String(number=w586, precision (6)=i16 2) -> (F-format string=w590:string)  [unwired: 2 in]
                      n274 = Concatenate Strings(w581, "\r\n", "Motor speed [rpm]: " ("string"), w590) -> (w585:string)
                      n275 = Greater Or Equal?(x=w586, y=w580) -> (x >= y?=w594:bool)
                      n276 = call <vilib>:"High Resolution Relative Seconds.vi"() -> ("relative seconds"=w603:dbl)
                      n277 = Subtract(x=w603, y=w602) -> (x-y=w598:dbl)
                      n278 = Less Or Equal?(x=w586, y=w579) -> (x <= y?=w593:bool)
                      n279 = And(x=w594, y=w593) -> (x .and. y?=w592:bool)
                      n280 = case shown="True" w592 {
                        selector: w592 -> [w604 w609]
                        tunnel: [w604 w608] -> w595
                        tunnel: w581 -> [_ w607]
                        tunnel: w583 -> [_ w606]
                        tunnel: w582 -> [_ w605]
                        frame False {
                        }
                        frame True {
                          n281 = flat-sequence {
                            tunnel: w609 -> [w616]
                            tunnel: [w616] -> w608
                            tunnel: w607 -> [w613]
                            tunnel: w606 -> [w612]
                            tunnel: w605 -> [w611]
                            frame #0 {
                              n282 = control-ref of="Pannel User Message"() -> (w614:refnum<vi>)
                              n283 = call "Write panel message (SubVI).vi"(4:"rpm"=w611, 5:"rpm"=TRUE ("rpm"), "Stop"=w612, "Time to wait"=20.0, "Strin"=w613, "String in"=w614) -> ()  [unwired: 5 in, 1 out]
                            }
                          }
                        }
                      }
                      n284 = Greater Or Equal?(x=w598, y=60.0) -> (x >= y?=w599:bool)
                      n285 = property on="Stop Button" class="Bool (strict)"() -> ("Value"=w584:bool)  [unwired: 2 in, 2 out]
                      n286 = Compound Arithmetic op=OR(w595, w599, w584) -> (w600:bool)
                      n287 = control-ref of="Pannel User Message"() -> (w591:refnum<vi>)
                      n288 = property class="Str"(reference=w591, "Value"=w585) -> ()  [unwired: 1 in, 2 out]
                    }
                    n289 = for {
                      N: 10 -> [_]
                      tunnel: w479 -> [w499]
                      tunnel: [w488] -> w474 mode=indexing
                      shift-right: [w489] -> w477
                      shift-left: w478 -> [w498]
                      tunnel: w458 -> [w487]
                      n290 = flat-sequence {
                        tunnel: w497 -> [w501]
                        tunnel: [w501] -> w494
                        tunnel: [w500] -> w493
                        frame #0 {
                          n291 = call <vilib>:"High Resolution Relative Seconds.vi"() -> ("relative seconds"=w500:dbl)
                        }
                      }
                      n292 = Byte Array To String(unsigned byte array=u8[] [75, 0, 4, 17, 0, 0, 0, 0] ("appended array")) -> (string=w496:string)
                      n293 = property class="VISAName"(reference=w499, error in=w498) -> (error out=w490:errorcluster, "Value"=w491:refnum<visa-resource-name>)  [unwired: 1 out]
                      n294 = VISA Write(VISA resource name=w491, write buffer=w496, error in (no error)=w490) -> (VISA resource name out=w495:refnum<visa-resource-name>, error out=w497:errorcluster)  [unwired: 1 out]
                      n295 = while {
                        tunnel: w495 -> [w515]
                        tunnel: w494 -> [w514]
                        tunnel: [w513] -> _
                        tunnel: [w512] -> w489
                        tunnel: w493 -> [w510]
                        tunnel: [w504] -> w488
                        tunnel: w487 -> [w502]
                        stop <- w506 stop-if-true
                        n296 = VISA Read(VISA resource name=w515, byte count=u32 1, error in (no error)=w514) -> (VISA resource name out=w517:refnum<visa-resource-name>, read buffer=w518:string, error out=w516:errorcluster)  [unwired: 1 out]
                        n297 = String To Byte Array(string=w518) -> (unsigned byte array=w521:u8[])
                        n298 = Index Array(array=w521, index=0) -> (element=w519:u8)
                        n299 = case shown="75" w519 {
                          tunnel: [w526 w531] -> w512
                          tunnel: w517 -> [w525 w540]
                          tunnel: w516 -> [w526 w539]
                          tunnel: [w525 w532] -> w513
                          tunnel: [u32 9999 w529] -> w504
                          tunnel: [FALSE w528] -> w505
                          tunnel: w502 -> [_ w527]
                          frame 0, Default {
                          }
                          frame 75 {
                            n300 = VISA Read(VISA resource name=w540, byte count=u32 3, error in (no error)=w539) -> (VISA resource name out=w535:refnum<visa-resource-name>, read buffer=w543:string, error out=w534:errorcluster)  [unwired: 1 out]
                            n301 = String To Byte Array(string=w543) -> (unsigned byte array=w533:u8[])
                            n302 = Index Array(array=w533, index #1=0 ("index")) -> (element #1=w538:u8, element #2=w536:u8)  [unwired: 2 in, 1 out]
                            n303 = Equal?(x=u8 0, y=w538) -> (x = y?=w537:bool)
                            n304 = case shown="True" w537 {
                              tunnel: [w546 w554] -> w531
                              tunnel: w536 -> [_ w561]
                              tunnel: w535 -> [w547 w560]
                              tunnel: w534 -> [w546 w559]
                              tunnel: w533 -> [_ w558]
                              tunnel: [w547 w556] -> w532
                              tunnel: [u32 9999 w550] -> w529
                              tunnel: [FALSE w549] -> w528
                              tunnel: w527 -> [_ w548]
                              frame False {
                              }
                              frame True {
                                n305 = VISA Read(VISA resource name=w560, byte count=w561, error in (no error)=w559) -> (VISA resource name out=w556:refnum<visa-resource-name>, read buffer=w555:string, error out=w554:errorcluster)  [unwired: 1 out]
                                n306 = String To Byte Array(string=w555) -> (unsigned byte array=w557:u8[])
                                n307 = Insert Into Array(array=w558, new element=w557) -> (w551:u8[])  [unwired: 1 in]
                                n308 = Index Array(array=w551, index #1=0 ("index")) -> (element #3=w552:u8)  [unwired: 2 in, 2 out]
                                n309 = case shown="15..19" w552 {
                                tunnel: w551 -> [_ w575]
                                tunnel: [u32 9999 w565] -> w550
                                tunnel: [FALSE w566] -> w549
                                tunnel: w548 -> [_ w564]
                                frame 0, Default {
                                }
                                frame 15..19 {
                                n310 = Index Array(array=w575, index #1=3 ("index")) -> (element #1=w574:u8, element #2=w573:u8, element #3=w572:u8, element #4=w571:u8)  [unwired: 3 in]
                                n311 = Join Numbers(hi=w571, lo=w572) -> ((hi.lo)=w569:u16)
                                n312 = Join Numbers(hi=w573, lo=w574) -> ((hi.lo)=w570:u16)
                                n313 = Join Numbers(hi=w569, lo=w570) -> ((hi.lo)=w567:u32)
                                n314 = Multiply(x=0.02003173828125, y=w567) -> (x*y=w565:dbl)
                                n315 = Greater Or Equal?(x=w565, y=w564) -> (x >= y?=w566:bool)
                                }
                                }
                              }
                            }
                          }
                        }
                        n316 = call <vilib>:"High Resolution Relative Seconds.vi"() -> ("relative seconds"=w511:dbl)
                        n317 = Subtract(x=w511, y=w510) -> (x-y=w509:dbl)
                        n318 = Greater Or Equal?(x=w509, y=2.0) -> (x >= y?=w507:bool)
                        n319 = property on="Stop Button" class="Bool (strict)"() -> ("Value"=w503:bool)  [unwired: 2 in, 2 out]
                        n320 = Compound Arithmetic op=OR(w503, w507, w505) -> (w506:bool)
                      }
                    }
                    n321 = Add Array Elements(numeric array=w474) -> (sum=w466:dbl)
                    n322 = Divide(x=w466, y=10.0 ("x")) -> (x/y=w465:dbl)
                    n323 = call "CANSendMotorSpeed.vi"("Remote"=TRUE, "error in (no error)"=w484, "Motor Speed RPM"=w462, "UUT"=w485, "Cluster in"=w486) -> ("error out"=w482:errorcluster)  [unwired: 6 in]
                    n324 = property on="CurrentOffset" class="DigNum (strict)"() -> ("Value"=w472:dbl)  [unwired: 2 in, 2 out]
                    n325 = Subtract(x=w465, y=w472) -> (x-y=w473:dbl)
                    "VC15100-2" <- w473
                    n326 = Greater Or Equal?(x=w473, y=w459) -> (x >= y?=w475:bool)
                    n327 = And(x=w475, y=w476) -> ()  [unwired: 1 out]
                  }
                  frame "RESET" {
                    # "Venable + Power ON"
                    # "Venable + Power OFF"
                    n328 = control-ref of="VISA resource name out"() -> (w652:refnum<vi>)
                    n329 = control-ref of="Config_CANAT"() -> (w639:refnum<vi>)
                    n330 = control-ref of="Motor Speed RPM"() -> (w620:refnum<vi>)
                    n331 = control-ref of="UUT"() -> (w640:refnum<vi>)
                    n332 = control-ref of="Pannel User Message"() -> (w627:refnum<vi>)
                    n333 = Byte Array To String(unsigned byte array=u8[] [75, 0, 4, 2, 0, 0, 2, 0]) -> (string=w650:string)
                    n334 = Byte Array To String(unsigned byte array=u8[] [75, 0, 4, 2, 0, 0, 18, 0]) -> (string=w653:string)
                    n335 = property on="VISA resource name" class="VISAName"() -> ("Value"=w636:refnum<visa-resource-name>)  [unwired: 2 in, 2 out]
                    n336 = VISA Flush I/O Buffer(VISA resource name=w636) -> (VISA resource name out=w637:refnum<visa-resource-name>)  [unwired: 2 in, 1 out]
                    n337 = Concatenate Strings("EP=1\r\nMD[1]=" ("write buffer"), "1" ("string"), "\r\n" ("string")) -> (w635:string)
                    n338 = call <vilib>:"Clear Errors.vi"("error in (no error)"=w638) -> ("error out"=w618:errorcluster)  [unwired: 5 in, 1 out]
                    n339 = call "CANSendMotorSpeed.vi"("Remote"=TRUE, "error in (no error)"=w618, "Motor Speed RPM"=u16 0, "UUT"=w640, "Cluster in"=w639) -> ("error out"=w630:errorcluster)  [unwired: 6 in]
                    n340 = call <vilib>:"Clear Errors.vi"("error in (no error)"=w630) -> ("error out"=w617:errorcluster)  [unwired: 5 in, 1 out]
                    n341 = call "SerialMarvinMod.vi"("error in (no error)"=w617, "Clear Log"=FALSE, "write buffer"=w635, "VISA resource name"=w637) -> ("error out"=w629:errorcluster)  [unwired: 6 in, 1 out]
                    n342 = call <vilib>:"Clear Errors.vi"("error in (no error)"=w629) -> ("error out"=w628:errorcluster)  [unwired: 5 in, 1 out]
                    n343 = property class="VISAName"(reference=w652, error in=w628) -> (error out=w651:errorcluster, "Value"=w654:refnum<visa-resource-name>)  [unwired: 1 out]
                    n344 = VISA Write(VISA resource name=w654, write buffer=w653, error in (no error)=w651) -> (VISA resource name out=w649:refnum<visa-resource-name>, error out=w625:errorcluster)  [unwired: 1 out]
                    n345 = call "Write panel message (SubVI).vi"(4:"rpm"=w620, 5:"rpm"=FALSE ("rpm"), "PrintTime"=TRUE, "Stop"=w622, "error in (no error)"=w625, "Time to wait"=15.0, "Strin"="7.5.2.4.Motor rotation direction test in process...\nSet parameters" ("string"), "String in"=w627) -> ("error out"=w624:errorcluster)  [unwired: 3 in]
                    n346 = VISA Write(VISA resource name=w649, write buffer=w650, error in (no error)=w624) -> (error out=w644:errorcluster)  [unwired: 2 out]
                  }
                  frame "VC15100-1" {
                    n347 = control-ref of="Config_CANAT"() -> (w680:refnum<vi>)
                    n348 = control-ref of="UUT"() -> (w679:refnum<vi>)
                    n349 = flat-sequence {
                      tunnel: [w773] -> w676
                      tunnel: w675 -> [w772]
                      tunnel: [w772] -> w674
                      frame #0 {
                        n350 = call <vilib>:"High Resolution Relative Seconds.vi"() -> ("relative seconds"=w773:dbl)
                      }
                    }
                    n351 = call "CANSendMotorSpeed.vi"("Remote"=TRUE, "error in (no error)"=w678, "Motor Speed RPM"=u16 15100, "UUT"=w679, "Cluster in"=w680) -> ("error out"=w675:errorcluster)  [unwired: 6 in]
                    n352 = property on="CurrentOffset" class="DigNum (strict)"() -> ("Value"=w668:dbl)  [unwired: 2 in, 2 out]
                    n353 = call <vilib>:"Clear Errors.vi"("error in (no error)"=w674) -> ("error out"=w667:errorcluster)  [unwired: 5 in, 1 out]
                    n354 = while {
                      tunnel: w676 -> [w798]
                      tunnel: w667 -> [w793]
                      tunnel: [w792] -> w671
                      tunnel: w658 -> [w780]
                      tunnel: [w774] -> w655
                      stop <- w796 stop-if-true
                      w777 = "7.5.2.4.Motor rotation direction test in process..." ("string")
                      n355 = control-ref of="Motor Speed RPM"() -> (w778:refnum<vi>)
                      n356 = control-ref of="Pannel User Message"() -> (w784:refnum<vi>)
                      n357 = call <vilib>:"High Resolution Relative Seconds.vi"() -> ("relative seconds"=w799:dbl)
                      n358 = Subtract(x=w799, y=w798) -> (x-y=w794:dbl)
                      n359 = Greater Or Equal?(x=w794, y=60.0) -> (x >= y?=w795:bool)
                      n360 = property on="Stop Button" class="Bool (strict)"() -> ("Value"=w779:bool)  [unwired: 2 in, 2 out]
                      n361 = property class="DigNum (strict)"(reference=w778, error in=w793) -> (error out=w775:errorcluster, "Value"=w782:dbl)  [unwired: 1 out]
                      "VC15100-1 Vel" <- w782
                      n362 = Number To Fractional String(number=w782, precision (6)=i16 2) -> (F-format string=w783:string)  [unwired: 2 in]
                      n363 = Concatenate Strings(w777, "\r\n", "Motor speed [rpm]: " ("string"), w783) -> (w781:string)
                      n364 = property class="Str"(reference=w784, "Value"=w781) -> ()  [unwired: 1 in, 2 out]
                      n365 = Greater Or Equal?(x=w782, y=12800.0) -> (x >= y?=w791:bool)
                      n366 = Less Or Equal?(x=w782, y=16000.0) -> (x <= y?=w790:bool)
                      n367 = And(x=w791, y=w790) -> (x .and. y?=w788:bool)
                      n368 = case shown="True" w788 {
                        selector: w788 -> [w808 w816]
                        tunnel: [w808 w815] -> w792
                        tunnel: w777 -> [_ w814]
                        tunnel: w780 -> [_ w813]
                        tunnel: w778 -> [_ w812]
                        tunnel: [w804 w811] -> w776
                        tunnel: w775 -> [w801 w810]
                        tunnel: [w802 w809] -> w774
                        frame False {
                          n369 = control-ref of="VISA resource name out"() -> (w807:refnum<vi>)
                          n370 = control-ref of="Stop Button"() -> (w806:refnum<vi>)
                          n371 = call "Read ADC Current (SubVI).vi"("error out"=w801, "Bool Refnum"=w806, "VISAResourceName in"=w807) -> ("error out 2"=w802:errorcluster, "Result"=w805:dbl)  [unwired: 7 in]
                          n372 = Greater Or Equal?(x=w805, y=60.0) -> (x >= y?=w804:bool)
                        }
                        frame True {
                          n373 = flat-sequence {
                            tunnel: w816 -> [_]
                            tunnel: [FALSE] -> w815
                            tunnel: w814 -> [w823]
                            tunnel: w813 -> [w822]
                            tunnel: w812 -> [w821]
                            tunnel: [w820] -> w811
                            tunnel: w810 -> [w818]
                            tunnel: [w817] -> w809
                            frame #0 {
                              n374 = disable-structure shown="Disabled" {
                                disable-tunnel: w823 -> [w827 _]
                                disable-tunnel: w822 -> [w826 _]
                                disable-tunnel: w821 -> [w824 _]
                                disable-tunnel: [_ w832] -> w820
                                disable-tunnel: w818 -> [_ w831]
                                disable-tunnel: [_ w830] -> w817
                                frame Disabled {
                                n375 = control-ref of="Pannel User Message"() -> (w829:refnum<vi>)
                                n376 = call "Write panel message (SubVI).vi"(4:"rpm"=w824, 5:"rpm"=TRUE ("rpm"), "Stop"=w826, "Time to wait"=20.0, "Strin"=w827, "String in"=w829) -> ()  [unwired: 5 in, 1 out]
                                }
                                frame Enabled {
                                n377 = control-ref of="VISA resource name out"() -> (w836:refnum<vi>)
                                n378 = control-ref of="Stop Button"() -> (w835:refnum<vi>)
                                n379 = call "Read ADC Current (SubVI).vi"("error out"=w831, "Bool Refnum"=w835, "VISAResourceName in"=w836) -> ("error out 2"=w830:errorcluster, "Result"=w833:dbl)  [unwired: 7 in]
                                n380 = Greater Or Equal?(x=w833, y=60.0) -> (x >= y?=w832:bool)
                                }
                              }
                            }
                          }
                        }
                      }
                      n381 = Compound Arithmetic op=OR(w792, w795, w779, w776) -> (w796:bool)
                    }
                    n382 = for {
                      N: 10 -> [_]
                      tunnel: [w684] -> w662 mode=indexing
                      tunnel: [T16."RESET"] -> w664
                      tunnel: w655 -> [w694]
                      tunnel: [w685] -> w672
                      tunnel: w657 -> [w682]
                      n383 = control-ref of="VISA resource name out"() -> (w681:refnum<vi>)
                      n384 = flat-sequence {
                        tunnel: w693 -> [w696]
                        tunnel: [w696] -> w690
                        tunnel: [w695] -> w689
                        frame #0 {
                          n385 = call <vilib>:"High Resolution Relative Seconds.vi"() -> ("relative seconds"=w695:dbl)
                        }
                      }
                      n386 = Byte Array To String(unsigned byte array=u8[] [75, 0, 4, 17, 0, 0, 0, 0] ("appended array")) -> (string=w692:string)
                      n387 = property class="VISAName"(reference=w681, error in=w694) -> (error out=w686:errorcluster, "Value"=w687:refnum<visa-resource-name>)  [unwired: 1 out]
                      n388 = VISA Write(VISA resource name=w687, write buffer=w692, error in (no error)=w686) -> (VISA resource name out=w691:refnum<visa-resource-name>, error out=w693:errorcluster)  [unwired: 1 out]
                      n389 = while {
                        tunnel: w691 -> [w710]
                        tunnel: w690 -> [w709]
                        tunnel: [w708] -> _
                        tunnel: [w707] -> w685
                        tunnel: w689 -> [w705]
                        tunnel: [w699] -> w684
                        tunnel: w682 -> [w697]
                        stop <- w701 stop-if-true
                        n390 = call <vilib>:"High Resolution Relative Seconds.vi"() -> ("relative seconds"=w706:dbl)
                        n391 = Subtract(x=w706, y=w705) -> (x-y=w704:dbl)
                        n392 = Greater Or Equal?(x=w704, y=2.0) -> (x >= y?=w702:bool)
                        n393 = property on="Stop Button" class="Bool (strict)"() -> ("Value"=w698:bool)  [unwired: 2 in, 2 out]
                        n394 = VISA Read(VISA resource name=w710, byte count=u32 1, error in (no error)=w709) -> (VISA resource name out=w712:refnum<visa-resource-name>, read buffer=w713:string, error out=w711:errorcluster)  [unwired: 1 out]
                        n395 = String To Byte Array(string=w713) -> (unsigned byte array=w716:u8[])
                        n396 = Index Array(array=w716, index=0) -> (element=w714:u8)
                        n397 = case shown="75" w714 {
                          tunnel: [w721 w726] -> w707
                          tunnel: w712 -> [w720 w735]
                          tunnel: w711 -> [w721 w734]
                          tunnel: [w720 w727] -> w708
                          tunnel: [u32 9999 w724] -> w699
                          tunnel: [FALSE w723] -> w700
                          tunnel: w697 -> [_ w722]
                          frame 0, Default {
                          }
                          frame 75 {
                            n398 = VISA Read(VISA resource name=w735, byte count=u32 3, error in (no error)=w734) -> (VISA resource name out=w730:refnum<visa-resource-name>, read buffer=w738:string, error out=w729:errorcluster)  [unwired: 1 out]
                            n399 = String To Byte Array(string=w738) -> (unsigned byte array=w728:u8[])
                            n400 = Index Array(array=w728, index #1=0 ("index")) -> (element #1=w733:u8, element #2=w731:u8)  [unwired: 2 in, 1 out]
                            n401 = Equal?(x=u8 0, y=w733) -> (x = y?=w732:bool)
                            n402 = case shown="True" w732 {
                              tunnel: [w741 w749] -> w726
                              tunnel: w731 -> [_ w756]
                              tunnel: w730 -> [w742 w755]
                              tunnel: w729 -> [w741 w754]
                              tunnel: w728 -> [_ w753]
                              tunnel: [w742 w751] -> w727
                              tunnel: [u32 9999 w745] -> w724
                              tunnel: [FALSE w744] -> w723
                              tunnel: w722 -> [_ w743]
                              frame False {
                              }
                              frame True {
                                n403 = VISA Read(VISA resource name=w755, byte count=w756, error in (no error)=w754) -> (VISA resource name out=w751:refnum<visa-resource-name>, read buffer=w750:string, error out=w749:errorcluster)  [unwired: 1 out]
                                n404 = String To Byte Array(string=w750) -> (unsigned byte array=w752:u8[])
                                n405 = Insert Into Array(array=w753, new element=w752) -> (w746:u8[])  [unwired: 1 in]
                                n406 = Index Array(array=w746, index #1=0 ("index")) -> (element #3=w747:u8)  [unwired: 2 in, 2 out]
                                n407 = case shown="15..19" w747 {
                                tunnel: w746 -> [_ w770]
                                tunnel: [u32 9999 w760] -> w745
                                tunnel: [FALSE w761] -> w744
                                tunnel: w743 -> [_ w759]
                                frame 0, Default {
                                }
                                frame 15..19 {
                                n408 = Index Array(array=w770, index #1=3 ("index")) -> (element #1=w769:u8, element #2=w768:u8, element #3=w767:u8, element #4=w766:u8)  [unwired: 3 in]
                                n409 = Join Numbers(hi=w766, lo=w767) -> ((hi.lo)=w764:u16)
                                n410 = Join Numbers(hi=w768, lo=w769) -> ((hi.lo)=w765:u16)
                                n411 = Join Numbers(hi=w764, lo=w765) -> ((hi.lo)=w762:u32)
                                n412 = Multiply(x=0.02003173828125, y=w762) -> (x*y=w760:dbl)
                                n413 = Greater Or Equal?(x=w760, y=w759) -> (x >= y?=w761:bool)
                                }
                                }
                              }
                            }
                          }
                        }
                        n414 = Compound Arithmetic op=OR(w698, w702, w700) -> (w701:bool)
                      }
                    }
                    n415 = Add Array Elements(numeric array=w662) -> (sum=w661:dbl)
                    n416 = Divide(x=w661, y=10.0) -> (x/y=w659:dbl)
                    n417 = Subtract(x=w659, y=w668) -> (x-y=w669:dbl)
                    "VC15100-1 Cur" <- w669
                    n418 = Greater Or Equal?(x=w669, y=w656) -> (x >= y?=w670:bool)
                    n419 = And(x=w670, y=w671) -> ()  [unwired: 1 out]
                  }
                  frame "MD0" {
                    n420 = control-ref of="Pannel User Message"() -> (w841:refnum<vi>)
                    n421 = property on="Serial" class="Bool (strict)"(error in=w844) -> (error out=w840:errorcluster, "Value"=w846:bool)  [unwired: 1 in, 1 out]
                    n422 = Select(t=T16."VC15100-1", s=w846, f=T16."STOP") -> (s? t:f=w847:T16)
                    n423 = property class="Str"(reference=w841, error in=w840, "Value"="7.5.2.4.Motor rotation direction test in process..." ("string")) -> (error out=w839:errorcluster)  [unwired: 1 out]
                    n424 = case shown="True" w846 {
                      tunnel: [w850 w860] -> w843
                      tunnel: w839 -> [w850 w859]
                      tunnel: w838 -> [_ w854]
                      frame False {
                        n425 = call "Display Message to User6"() -> ()  [unwired: 10 in, 2 out]
                      }
                      frame True {
                        (unwired) TRUE ("Remote")
                        # "Venable + Power ON"
                        # "Venable + Power OFF"
                        n426 = control-ref of="VISA resource name out"() -> (w867:refnum<vi>)
                        n427 = control-ref of="Config_CANAT"() -> (w873:refnum<vi>)
                        n428 = control-ref of="UUT"() -> (w874:refnum<vi>)
                        n429 = control-ref of="Motor Speed RPM"() -> (w852:refnum<vi>)
                        n430 = control-ref of="Pannel User Message"() -> (w858:refnum<vi>)
                        n431 = Byte Array To String(unsigned byte array=u8[] [75, 0, 4, 2, 0, 0, 2, 0]) -> (string=w865:string)
                        n432 = Byte Array To String(unsigned byte array=u8[] [75, 0, 4, 2, 0, 0, 18, 0]) -> (string=w868:string)
                        n433 = property on="VISA resource name" class="VISAName"() -> ("Value"=w880:refnum<visa-resource-name>)  [unwired: 2 in, 2 out]
                        n434 = VISA Flush I/O Buffer(VISA resource name=w880) -> (VISA resource name out=w881:refnum<visa-resource-name>)  [unwired: 2 in, 1 out]
                        n435 = Concatenate Strings("EP=1\r\nMD[1]=" ("write buffer"), "0" ("string"), "\r\n" ("string")) -> (w879:string)
                        n436 = call "CANSendMotorSpeed.vi"("error in (no error)"=w859, "Motor Speed RPM"=u16 0, "UUT"=w874, "Cluster in"=w873) -> ("error out"=w871:errorcluster)  [unwired: 7 in]
                        n437 = call "SerialMarvinMod.vi"("error in (no error)"=w871, "Clear Log"=FALSE, "write buffer"=w879, "VISA resource name"=w881) -> ("error out"=w870:errorcluster)  [unwired: 6 in, 1 out]
                        n438 = call <vilib>:"Clear Errors.vi"("error in (no error)"=w870) -> ("error out"=w861:errorcluster)  [unwired: 5 in, 1 out]
                        n439 = property class="VISAName"(reference=w867, error in=w861) -> (error out=w866:errorcluster, "Value"=w869:refnum<visa-resource-name>)  [unwired: 1 out]
                        n440 = VISA Write(VISA resource name=w869, write buffer=w868, error in (no error)=w866) -> (VISA resource name out=w864:refnum<visa-resource-name>, error out=w856:errorcluster)  [unwired: 1 out]
                        n441 = call "Write panel message (SubVI).vi"(4:"rpm"=w852, 5:"rpm"=FALSE ("rpm"), "Stop"=w854, "error in (no error)"=w856, "Time to wait"=15.0, "Strin"="7.5.2.4.Motor rotation direction test in process...\nSet parameters" ("string"), "String in"=w858) -> ("error out"=w855:errorcluster)  [unwired: 4 in]
                        n442 = VISA Write(VISA resource name=w864, write buffer=w865, error in (no error)=w855) -> (error out=w860:errorcluster)  [unwired: 2 out]
                      }
                    }
                  }
                }
                n443 = property on="Stop Button" class="Bool (strict)"() -> ("Value"=w434:bool)  [unwired: 2 in, 2 out]
                n444 = Compound Arithmetic op=OR(w436, w434) -> (w435:bool)
              }
            }
            frame Disabled {
              n445 = call "Display Message to User"("error in (no error)"=w883) -> ("error out"=w882:errorcluster, "YES"=w884:bool)  [unwired: 9 in]
            }
          }
          n446 = And(x=w341, y=w340) -> (x .and. y?=→"EnableTestind":bool)
          n447 = call "CANSendMotorSpeed.vi"("Remote"=FALSE, "error in (no error)"=w344, "Motor Speed RPM"=u16 0, "UUT"=w346, "Cluster in"=w345) -> ("error out"=w343:errorcluster)  [unwired: 6 in]
          n448 = property class="Tbl (strict)"(reference=w318, error in=w343) -> (reference out=w377:refnum<vi>, error out=w384:errorcluster, "Value"=w383:string[][])
          n449 = Index Array(array=w383, index (col)=0 ("disabled index (col)")) -> (element=w382:string[])  [unwired: 1 in]
          n450 = call "Find_Number_LineMARVIN.vi"("Test Paragraph"="7.5.2.4", "error in"=w384, "Row Headers[]"=w382) -> ("error out"=w381:errorcluster, "Line number"=w378:i32)  [unwired: 2 in, 2 out]
          n451 = call "PassOrFail (SubVI).vi"("disabled index (col)"=6, "index (row)"=w378, "error in (no error)"=w381, "Boolean"=w340, "Table in"=w377) -> ("error out"=w379:errorcluster)  [unwired: 6 in]
          n452 = disable-structure shown="Enabled" {
            disable-tunnel: w379 -> [w411 w417]
            disable-tunnel: w378 -> [w408 _]
            disable-tunnel: _ -> [w407 _]
            disable-tunnel: w377 -> [w406 _]
            disable-tunnel: [w405 w417] -> w354
            frame Disabled {
              n453 = property class="Tbl (strict)"(reference=w406, error in=w411) -> (reference out=w416:refnum<vi>, error out=w412:errorcluster, "Value"=w415:string[][])
              n454 = Number To Fractional String(number=w407, precision (6)=i16 4) -> (F-format string=w409:string)  [unwired: 2 in]
              n455 = Replace Array Subset(array=w415, new element=w409, index (row)=w408, index (col)=5 ("disabled index (col)")) -> (w414:string[][])
              n456 = property class="Tbl (strict)"(reference=w416, error in=w412, "Value"=w414) -> (error out=w405:errorcluster)  [unwired: 1 out]
            }
            frame Enabled {
            }
          }
          n457 = property class="VISAName"(reference=w363, error in=w354) -> (error out=w362:errorcluster, "Value"=w372:refnum<visa-resource-name>)  [unwired: 1 out]
          n458 = VISA Write(VISA resource name=w372, write buffer=w364, error in (no error)=w362) -> (error out=w331:errorcluster)  [unwired: 2 out]
          n459 = call <vilib>:"Clear Errors.vi"("error in (no error)"=w331) -> ("error out"=w330:errorcluster)  [unwired: 5 in, 1 out]
          n460 = call "Time Delay14"("error in (no error)"=w330) -> ("error out"=w316:errorcluster)  [unwired: 10 in]
          n461 = property on="Start" class="Bool (strict)"(error in=w316, "DisabledEnum"=w333) -> (error out=w332:errorcluster)  [unwired: 1 in, 1 out]
          n462 = property on="Report" class="Bool (strict)"(error in=w332, "DisabledEnum"=w333) -> ()  [unwired: 1 in, 2 out]
        }
        frame "Speed Command" {
          w976 = T13."Disabled and Grayed Out" ("Disabled")
          w980 = T13."Enabled" ("Disabled")
          w1060 = "7.5.3" ("Test Paragraph")
          w969 = "7.5.4" ("Test Paragraph")
          n463 = control-ref of="Pannel User Message"() -> (w991:refnum<vi>)
          n464 = property class="Str"(reference=w991, error in=w975, "Value"="7.5.4.Speed Command Test") -> (error out=w990:errorcluster)  [unwired: 1 out]
          n465 = property on="Start" class="Bool (strict)"(error in=w975, "DisabledEnum"=w976) -> (error out=w977:errorcluster)  [unwired: 1 in, 1 out]
          n466 = Initialize Array(FALSE, 14 ("dimension size")) -> (w1038:bool[])
          n467 = property on="Report" class="Bool (strict)"(error in=w977, "DisabledEnum"=w976) -> ()  [unwired: 1 in, 2 out]
          n468 = Build Array (concatenate)(w1038, bool[] [FALSE, FALSE, FALSE, TRUE, FALSE, FALSE, FALSE] ("array")) -> (w1039:bool[])
          n469 = call "Table_ScrollaBarMarvin.vi"("error in"=w990, "Line to focus"=w969, "reference in"=w970) -> ("error out"=w1071:errorcluster)  [unwired: 2 out]
          n470 = Boolean Array To Number(Boolean array=w1039) -> (number=w1037:u32)
          n471 = call "Reset old test Values (SubVI).vi"("error in"=w1071, "Atr in"=w970, "Test Paragraph"=w969) -> ("error out"=w971:errorcluster)  [unwired: 8 in]
          n472 = property class="Tbl (strict)"(reference=w970, error in=w971) -> (error out=w1073:errorcluster, "Value"=w1074:string[][])  [unwired: 1 out]
          n473 = To Unsigned Long Integer(number=w1037) -> (unsigned 32bit integer=w1028:u32)
          n474 = control-ref of="VISA resource name out"() -> (w1002:refnum<vi>)
          n475 = control-ref of="VISA resource name out"() -> (w1026:refnum<vi>)
          n476 = control-ref of="Config_CANAT"() -> (w1068:refnum<vi>)
          n477 = control-ref of="UUT"() -> (w1067:refnum<vi>)
          n478 = Initialize Array(FALSE, 14 ("dimension size")) -> (w1014:bool[])
          n479 = Build Array (concatenate)(w1014, bool[] [FALSE, FALSE, FALSE, FALSE, FALSE, FALSE, FALSE] ("array")) -> (w1015:bool[])
          n480 = Boolean Array To Number(Boolean array=w1015) -> (number=w1013:u32)
          n481 = To Unsigned Long Integer(number=w1013) -> (unsigned 32bit integer=w1004:u32)
          n482 = Split Number(x=w1004) -> (hi(x)=w1009:u16, lo(x)=w1010:u16)
          n483 = Split Number(x=w1010) -> (hi(x)=w1008:u8, lo(x)=w1007:u8)
          n484 = property on="UUT" class="Str"() -> ("Value"=w974:string)  [unwired: 2 in, 2 out]
          n485 = Equal?(x=w974, y="EBAY") -> (x = y?=w972:bool)
          n486 = case shown="False" w972 {
            tunnel: [u16[] [6000, 9000, 12100] u16[] [6000, 11500, 15100]] -> w1069
            frame False {
            }
            frame True {
            }
          }
          n487 = Split Number(x=w1028) -> (hi(x)=w1033:u16, lo(x)=w1034:u16)
          n488 = Split Number(x=w1009) -> (hi(x)=w1006:u8, lo(x)=w1005:u8)
          n489 = Build Array(u8 75, u8 0 ("element"), u8 4 ("Length"), u8 2, w1007, w1008, w1005, w1006) -> (w1012:u8[])
          n490 = Byte Array To String(unsigned byte array=w1012) -> (string=w1003:string)
          n491 = Split Number(x=w1034) -> (hi(x)=w1032:u8, lo(x)=w1031:u8)
          n492 = Concatenate Strings("7.5.3.Stop Time Test in process... ", "\r\n", "Motor Speed [rpm]: " ("string")) -> (w985:string)
          n493 = Index Array(array=w1074, index (col)=0 ("disabled index (col)")) -> (element=w1075:string[])  [unwired: 1 in]
          n494 = Split Number(x=w1033) -> (hi(x)=w1030:u8, lo(x)=w1029:u8)
          n495 = Build Array(u8 75, u8 0 ("element"), u8 4 ("Length"), u8 2, w1031, w1032, w1029, w1030) -> (w1036:u8[])
          n496 = Byte Array To String(unsigned byte array=w1036) -> (string=w1027:string)
          n497 = call "Find_Number_LineMARVIN.vi"("Test Paragraph"=w969, "error in"=w1073, "Row Headers[]"=w1075) -> ("error out"=w1017:errorcluster, "Line number"=w1070:i32)  [unwired: 2 in, 2 out]
          n498 = property class="VISAName"(reference=w1026, error in=w1017) -> (error out=w1025:errorcluster, "Value"=w1035:refnum<visa-resource-name>)  [unwired: 1 out]
          n499 = VISA Write(VISA resource name=w1035, write buffer=w1027, error in (no error)=w1025) -> (error out=w1016:errorcluster)  [unwired: 2 out]
          n500 = for {
            tunnel: w1016 -> [w1123]
            tunnel: w970 -> [w1120]
            tunnel: w1070 -> [w1109]
            tunnel: w1069 -> [w1112] mode=indexing
            tunnel: [w1107] -> w1066
            tunnel: [w1099] -> w984 mode=indexing
            i -> [w1111]
            w1113 = 200.0 ("y")
            n501 = control-ref of="Config_CANAT"() -> (w1129:refnum<vi>)
            n502 = control-ref of="Motor Speed RPM"() -> (w1128:refnum<vi>)
            n503 = control-ref of="UUT"() -> (w1130:refnum<vi>)
            n504 = Add(x=w1112, y=w1113) -> (x+y=w1115:dbl)
            n505 = Subtract(x=w1112, y=w1113) -> (x-y=w1114:dbl)
            n506 = Increment(x=w1111) -> (x+1=w1110:i32)
            n507 = Add(x=w1109, y=w1110) -> (x+y=w1106:i32)
            n508 = call "CANSendMotorSpeed.vi"("Remote"=TRUE, "error in (no error)"=w1123, "Motor Speed RPM"=w1112, "UUT"=w1130, "Cluster in"=w1129) -> ("error out"=w1104:errorcluster)  [unwired: 6 in]
            n509 = call <vilib>:"High Resolution Relative Seconds.vi"() -> ("relative seconds"=w1100:dbl)
            n510 = while {
              tunnel: w1104 -> [w1150]
              tunnel: [w1150] -> w1103
              tunnel: "7.5.4.Speed Command Test" ("Value") -> [w1147]
              tunnel: "Time to wait: " ("Value") -> [w1145]
              tunnel: w1100 -> [w1143]
              stop <- w1135 stop-if-true
              n511 = control-ref of="Pannel User Message"() -> (w1149:refnum<vi>)
              n512 = call <vilib>:"High Resolution Relative Seconds.vi"() -> ("relative seconds"=w1144:dbl)
              n513 = Subtract(x=w1144, y=w1143) -> (x-y=w1141:dbl)
              n514 = property on="Stop Button" class="Bool (strict)"() -> ("Value"=w1134:bool)  [unwired: 2 in, 2 out]
              n515 = Subtract(x=35.0, y=w1141) -> (x-y=w1136:dbl)
              n516 = Less Or Equal To 0?(x=w1136) -> (x <= 0?=w1142:bool)
              n517 = Compound Arithmetic op=OR(w1142, w1134) -> (w1135:bool)
              n518 = Number To Fractional String(number=w1136, precision (6)=i16 2) -> (F-format string=w1138:string)  [unwired: 2 in]
              n519 = property on="Motor Speed RPM" class="DigNum (strict)"() -> ("Value"=w1132:dbl)  [unwired: 2 in, 2 out]
              n520 = Number To Fractional String(number=w1132, precision (6)=i16 2) -> (F-format string=w1131:string)  [unwired: 2 in]
              n521 = Concatenate Strings(w1147, "\r\n", w1145, w1138, "  Sec.\nMotor speed [rpm]: " ("string"), w1131) -> (w1148:string)
              n522 = property class="Str"(reference=w1149, "Value"=w1148) -> ()  [unwired: 1 in, 2 out]
            }
            n523 = property class="DigNum (strict)"(reference=w1128, error in=w1103) -> (error out=w1121:errorcluster, "Value"=w1122:dbl)  [unwired: 1 out]
            n524 = In Range and Coerce(upper limit=w1115, x=w1122, lower limit=w1114) -> (In Range?=w1099:bool)  [unwired: 1 out]
            n525 = call "PassOrFail (SubVI).vi"("disabled index (col)"=6, "index (row)"=w1106, "error in (no error)"=w1121, "Boolean"=w1099, "Table in"=w1120) -> ("error out"=w1125:errorcluster)  [unwired: 6 in]
            n526 = property class="Tbl (strict)"(reference=w1120, error in=w1125) -> (reference out=w1116:refnum<vi>, error out=w1126:errorcluster, "Value"=w1117:string[][])
            n527 = Number To Fractional String(number=w1122, precision (6)=i16 2) -> (F-format string=w1119:string)  [unwired: 2 in]
            n528 = Replace Array Subset(array=w1117, new element=w1119, index (row)=w1106, index (col)=5 ("disabled index (col)")) -> (w1118:string[][])
            n529 = property class="Tbl (strict)"(reference=w1116, error in=w1126, "Value"=w1118) -> (error out=w1107:errorcluster)  [unwired: 1 out]
          }
          n530 = call "CANSendMotorSpeed.vi"("Remote"=TRUE, "error in (no error)"=w1066, "Motor Speed RPM"=u16 0, "UUT"=w1067, "Cluster in"=w1068) -> ("error out"=w1063:errorcluster)  [unwired: 6 in]
          n531 = while {
            tunnel: w1064 -> [w1095]
            tunnel: w1062 -> [w1089]
            tunnel: [w1090] -> w1041
            tunnel: [w1086] -> w1053
            tunnel: w985 -> [w1083]
            stop <- w1093 stop-if-true
            n532 = control-ref of="Motor Speed RPM"() -> (w1098:refnum<vi>)
            n533 = control-ref of="Pannel User Message"() -> (w1088:refnum<vi>)
            n534 = call <vilib>:"High Resolution Relative Seconds.vi"() -> ("relative seconds"=w1096:dbl)
            n535 = Subtract(x=w1096, y=w1095) -> (x-y=w1090:dbl)
            n536 = property class="DigNum (strict)"(reference=w1098, error in=w1089) -> (error out=w1087:errorcluster, "Value"=w1081:dbl)  [unwired: 1 out]
            n537 = Number To Fractional String(number=w1081, precision (6)=i16 2) -> (F-format string=w1082:string)  [unwired: 2 in]
            n538 = Concatenate Strings(w1083, w1082) -> (w1084:string)
            n539 = property class="Str"(reference=w1088, error in=w1087, "Value"=w1084) -> (error out=w1086:errorcluster)  [unwired: 1 out]
            n540 = Less Or Equal?(x=w1081, y=0.0) -> (x <= y?=w1092:bool)
            n541 = Greater Or Equal?(x=w1090, y=50.0) -> (x >= y?=w1091:bool)
            n542 = property on="Stop Button" class="Bool (strict)"() -> ("Value"=w1080:bool)  [unwired: 2 in, 2 out]
            n543 = Compound Arithmetic op=OR(w1092, w1091, w1080) -> (w1093:bool)
          }
          n544 = Less?(x=w1041, y=50.0) -> (x < y?=w983:bool)
          n545 = call "Table_ScrollaBarMarvin.vi"("error in"=w1053, "Line to focus"=w1060, "reference in"=w970) -> ("error out"=w1061:errorcluster)  [unwired: 2 out]
          n546 = property class="Tbl (strict)"(reference=w970, error in=w1061) -> (reference out=w1040:refnum<vi>, error out=w1058:errorcluster, "Value"=w1057:string[][])
          n547 = Index Array(array=w1057, index (col)=0 ("disabled index (col)")) -> (element=w1056:string[])  [unwired: 1 in]
          n548 = call "Find_Number_LineMARVIN.vi"("Test Paragraph"=w1060, "error in"=w1058, "Row Headers[]"=w1056) -> ("error out"=w1054:errorcluster, "Line number"=w1055:i32)  [unwired: 2 in, 2 out]
          n549 = Build Array (concatenate)(w984, w983) -> (w982:bool[])
          n550 = And Array Elements(Boolean array=w982) -> (logical AND=→"SpeedStopind":bool)
          n551 = Increment(x=w1055) -> (x+1=w1042:i32)
          n552 = call "PassOrFail (SubVI).vi"("disabled index (col)"=6, "index (row)"=w1042, "error in (no error)"=w1054, "Boolean"=w983, "Table in"=w1040) -> ("error out"=w1046:errorcluster)  [unwired: 6 in]
          n553 = property class="Tbl (strict)"(reference=w1040, error in=w1046) -> (reference out=w1051:refnum<vi>, error out=w1047:errorcluster, "Value"=w1050:string[][])
          n554 = Number To Fractional String(number=w1041, precision (6)=i16 2) -> (F-format string=w1043:string)  [unwired: 2 in]
          n555 = Replace Array Subset(array=w1050, new element=w1043, index (row)=w1042, index (col)=5 ("disabled index (col)")) -> (w1049:string[][])
          n556 = property class="Tbl (strict)"(reference=w1051, error in=w1047, "Value"=w1049) -> (error out=w993:errorcluster)  [unwired: 1 out]
          n557 = property class="VISAName"(reference=w1002, error in=w993) -> (error out=w1001:errorcluster, "Value"=w1011:refnum<visa-resource-name>)  [unwired: 1 out]
          n558 = VISA Write(VISA resource name=w1011, write buffer=w1003, error in (no error)=w1001) -> (error out=w978:errorcluster)  [unwired: 2 out]
          n559 = property on="Start" class="Bool (strict)"(error in=w978, "DisabledEnum"=w980) -> (error out=w979:errorcluster)  [unwired: 1 in, 1 out]
          n560 = property on="Report" class="Bool (strict)"(error in=w979, "DisabledEnum"=w980) -> ()  [unwired: 1 in, 2 out]
          n561 = flat-sequence {
            tunnel: [w1079] -> w1064
            tunnel: w1063 -> [w1078]
            tunnel: [w1078] -> w1062
            frame #0 {
              n562 = call <vilib>:"High Resolution Relative Seconds.vi"() -> ("relative seconds"=w1079:dbl)
            }
          }
        }
        frame "Stop Time" {
          w1168 = T13."Enabled" ("Disabled")
          w1169 = T13."Disabled and Grayed Out" ("Disabled")
          w1156 = "9.Motor Temperature  test in process..." ("Value")
          w1165 = "9" ("Test Paragraph")
          # "k15 = 64\nk16 = 128"
          # "K15+Venable"
          # "Deg"
          # "K15 OFF"
          n563 = property on="Stop Button" class="Bool (strict)"("DisabledEnum"=w1169) -> ()  [unwired: 2 in, 2 out]
          n564 = Byte Array To String(unsigned byte array=u8[] [75, 0, 4, 2, 0, 64, 0, 0] ("appended array")) -> ()  [unwired: 1 out]
          n565 = property on="Start" class="Bool (strict)"(error in=w1173, "DisabledEnum"=w1169) -> (error out=w1174:errorcluster)  [unwired: 1 in, 1 out]
          n566 = property on="Report" class="Bool (strict)"(error in=w1174, "DisabledEnum"=w1169) -> (error out=w1172:errorcluster)  [unwired: 1 in, 1 out]
          n567 = control-ref of="VISA resource name out"() -> (w1194:refnum<vi>)
          n568 = control-ref of="Stop Button"() -> (w1159:refnum<vi>)
          n569 = control-ref of="Config_CANAT"() -> (w1185:refnum<vi>)
          n570 = control-ref of="UUT"() -> (w1186:refnum<vi>)
          n571 = control-ref of="Motor Speed RPM"() -> (w1157:refnum<vi>)
          n572 = control-ref of="Pannel User Message"() -> (w1190:refnum<vi>)
          n573 = control-ref of="Pannel User Message"() -> (w1158:refnum<vi>)
          n574 = Byte Array To String(unsigned byte array=u8[] [75, 0, 4, 2, 0, 0, 0, 0] ("appended array")) -> (string=w1197:string)
          n575 = property on="Index" class="Str"() -> ("Value"=w1155:string)  [unwired: 2 in, 2 out]
          n576 = Decimal String To Number(string=w1155) -> (number=w1154:i32)  [unwired: 2 in, 1 out]
          n577 = Subtract(x=w1154, y=3 ("x")) -> (x-y=w1153:i32)
          n578 = Number To Decimal String(number=w1153) -> (decimal integer string=w1152:string)  [unwired: 1 in]
          n579 = property class="Str"(reference=w1190, error in=w1172, "Value"=w1156) -> (error out=w1189:errorcluster)  [unwired: 1 out]
          n580 = call "Reset old test Values (SubVI).vi"("error in"=w1189, "Atr in"=w1166, "Test Paragraph"=w1165) -> ("error out"=w1167:errorcluster)  [unwired: 8 in]
          n581 = call "Table_ScrollaBarMarvin.vi"("error in"=w1167, "Line to focus"=w1165, "reference in"=w1166) -> ("error out"=w1204:errorcluster)  [unwired: 2 out]
          n582 = property class="Tbl (strict)"(reference=w1166, error in=w1204) -> (reference out=w1188:refnum<vi>, error out=w1203:errorcluster, "Value"=w1202:string[][])
          n583 = Index Array(array=w1202, index (col)=0 ("disabled index (col)")) -> (element=w1201:string[])  [unwired: 1 in]
          n584 = call "Find_Number_LineMARVIN.vi"("Test Paragraph"=w1165, "error in"=w1203, "Row Headers[]"=w1201) -> ("error out"=w1199:errorcluster, "Line number"=w1179:i32)  [unwired: 2 in, 2 out]
          n585 = call "Table_ScrollaBarMarvin.vi"("error in"=w1199, "Line to focus"=w1165, "reference in"=w1188) -> ("error out"=w1182:errorcluster)  [unwired: 2 out]
          n586 = call "CANSendMotorSpeed.vi"("Remote"=FALSE, "error in (no error)"=w1182, "Motor Speed RPM"=u16 0, "UUT"=w1186, "Cluster in"=w1185) -> ("error out"=w1181:errorcluster)  [unwired: 6 in]
          n587 = property class="VISAName"(reference=w1194, error in=w1181) -> (error out=w1180:errorcluster, "Value"=w1205:refnum<visa-resource-name>)  [unwired: 1 out]
          n588 = call "Write panel message (SubVI).vi"("rpm"=w1157, "Stop"=w1159, "error in (no error)"=w1180, "Time to wait"=5.0 ("Delay Time (sec)"), "Strin"=w1156, "String in"=w1158) -> ("error out"=w1192:errorcluster)  [unwired: 5 in]
          n589 = call "Time Delay2"("error in (no error)"=w1192) -> ("error out"=w1163:errorcluster)  [unwired: 10 in]
          n590 = call "Write panel message (SubVI).vi"("rpm"=w1157, "PrintTime"=FALSE, "Stop"=w1159, "error in (no error)"=w1163, "Time to wait"=0.01, "Strin"=w1156, "String in"=w1158) -> ("error out"=w1162:errorcluster)  [unwired: 4 in]
          n591 = call <vilib>:"Clear Errors.vi"("error in (no error)"=w1162) -> ("error out"=w1164:errorcluster)  [unwired: 5 in, 1 out]
          n592 = for {
            tunnel: w1164 -> [w1256]
            tunnel: dbl[] [1288.0, 1569.0, 1774.0] -> [w1236] mode=indexing
            tunnel: w1188 -> [w1250]
            tunnel: w1188 -> [w1245]
            tunnel: [w1238] -> w1170
            tunnel: w1205 -> [w1244]
            tunnel: w1179 -> [w1234]
            tunnel: dbl[] [60.0, 90.0, 110.0] -> [w1231] mode=indexing
            tunnel: [w1229] -> w1177 mode=indexing
            tunnel: u32[] [128, 1024, 4096] -> [w1215] mode=indexing
            tunnel: w1159 -> [w1212]
            tunnel: w1158 -> [w1211]
            tunnel: w1157 -> [w1210]
            tunnel: w1156 -> [w1207]
            tunnel: w1152 -> [w1206]
            i -> [w1228]
            w1237 = 3.0 ("y")
            n593 = Add(x=w1231, y=w1237) -> (x+y=w1241:dbl)
            n594 = Increment(x=w1234) -> (x+1=w1233:i32)
            n595 = Subtract(x=w1231, y=w1237) -> (x-y=w1242:dbl)
            n596 = Add(x=w1233, y=w1228) -> (x+y=w1232:i32)
            n597 = call "DegToDAC (SubVI).vi"("error in (no error)"=w1256, "R2"=10.0, "Numeric"=w1236) -> ("error out"=w1240:errorcluster)  [unwired: 7 in, 1 out]
            n598 = To Unsigned Long Integer(number=w1215) -> (unsigned 32bit integer=w1218:u32)
            n599 = Split Number(x=w1218) -> (hi(x)=w1223:u16, lo(x)=w1224:u16)
            n600 = Split Number(x=w1224) -> (hi(x)=w1222:u8, lo(x)=w1221:u8)
            n601 = Split Number(x=w1223) -> (hi(x)=w1220:u8, lo(x)=w1219:u8)
            n602 = Build Array(u8 75, u8 0 ("element"), u8 4 ("Length"), u8 2, w1221, w1222, w1219, w1220) -> (w1216:u8[])
            n603 = Byte Array To String(unsigned byte array=w1216) -> (string=w1214:string)
            n604 = VISA Write(VISA resource name=w1244, write buffer=w1214, error in (no error)=w1240) -> (error out=w1243:errorcluster)  [unwired: 2 out]
            n605 = call "Write panel message (SubVI).vi"(4:"rpm"=w1210, 5:"rpm"=FALSE ("rpm"), "PrintTime"=TRUE, "Stop"=w1212, "error in (no error)"=w1243, "Time to wait"=3.0, "Strin"=w1207, "String in"=w1211) -> ("error out"=w1235:errorcluster)  [unwired: 3 in]
            n606 = disable-structure shown="Enabled" {
              disable-tunnel: [w1260 w1270] -> w1249
              disable-tunnel: [w1258 w1266] -> w1239
              disable-tunnel: w1235 -> [w1257 w1269]
              disable-tunnel: w1206 -> [_ w1261]
              frame Disabled {
                n607 = control-ref of="Motor Stator Temp."() -> (w1259:refnum<vi>)
                n608 = property class="DigNum (strict)"(reference=w1259, error in=w1257) -> (error out=w1260:errorcluster, "Value"=w1258:dbl)  [unwired: 1 out]
              }
              frame Enabled {
                n609 = for {
                  N: 6 -> [_]
                  tunnel: [w1283] -> w1271 mode=indexing
                  tunnel: w1269 -> [w1279]
                  tunnel: [w1282] -> w1270
                  tunnel: w1261 -> [w1273]
                  n610 = Search and Replace String(input string="TA[2]\r\n" ("write buffer"), search string="2", replace string=w1273) -> (result string=w1272:string)  [unwired: 5 in, 3 out]
                  n611 = property on="VISA resource name" class="VISAName"() -> ("Value"=w1280:refnum<visa-resource-name>)  [unwired: 2 in, 2 out]
                  n612 = call "Time Delay15"("error in (no error)"=w1279) -> ("error out"=w1276:errorcluster)  [unwired: 10 in]
                  n613 = VISA Flush I/O Buffer(VISA resource name=w1280, error in (no error)=w1276) -> (VISA resource name out=w1277:refnum<visa-resource-name>, error out=w1278:errorcluster)  [unwired: 1 in]
                  n614 = call "SerialMarvinMod.vi"("error in (no error)"=w1278, "write buffer"=w1272, "VISA resource name"=w1277) -> ("error out"=w1282:errorcluster, "read buffer"=w1281:string)  [unwired: 7 in]
                  n615 = Fract/Exp String To Number(string=w1281) -> (number=w1283:dbl)  [unwired: 3 in, 1 out]
                }
                n616 = Delete From Array(array=w1271, length=1, index=0) -> (array with subset deleted=w1264:dbl[])  [unwired: 1 out]
                n617 = Add Array Elements(numeric array=w1264) -> (sum=w1267:dbl)
                n618 = Divide(x=w1267, y=5.0) -> (x/y=w1266:dbl)
              }
            }
            n619 = In Range and Coerce(upper limit=w1241, x=w1239, lower limit=w1242) -> (In Range?=w1229:bool)  [unwired: 1 out]
            n620 = call "PassOrFail (SubVI).vi"("disabled index (col)"=6, "index (row)"=w1232, "error in (no error)"=w1249, "Boolean"=w1229, "Table in"=w1245) -> ("error out"=w1253:errorcluster)  [unwired: 6 in]
            n621 = property class="Tbl (strict)"(reference=w1250, error in=w1253) -> (error out=w1246:errorcluster, "Value"=w1255:string[][])  [unwired: 1 out]
            n622 = Number To Fractional String(number=w1239, precision (6)=i16 2) -> (F-format string=w1254:string)  [unwired: 2 in]
            n623 = Replace Array Subset(array=w1255, new element=w1254, index (row)=w1232, index (col)=5 ("disabled index (col)")) -> (w1247:string[][])
            n624 = property class="Tbl (strict)"(reference=w1245, error in=w1246, "Value"=w1247) -> (error out=w1238:errorcluster)  [unwired: 1 out]
          }
          n625 = And Array Elements(Boolean array=w1177) -> (logical AND=→"MotorTempind":bool)
          n626 = property class="VISAName"(reference=w1194, error in=w1170) -> (error out=w1196:errorcluster, "Value"=w1198:refnum<visa-resource-name>)  [unwired: 1 out]
          n627 = VISA Write(VISA resource name=w1198, write buffer=w1197, error in (no error)=w1196) -> ()  [unwired: 3 out]
          n628 = property on="Start" class="Bool (strict)"(error in=w1170, "DisabledEnum"=w1168) -> (error out=w1171:errorcluster)  [unwired: 1 in, 1 out]
          n629 = property on="Report" class="Bool (strict)"(error in=w1171, "DisabledEnum"=w1168) -> ()  [unwired: 1 in, 2 out]
          n630 = property on="Stop Button" class="Bool (strict)"("DisabledEnum"=w1168) -> ()  [unwired: 2 in, 2 out]
        }
        frame "Temp Control" {
          (unwired) dbl[] [5927.0, 11480.0, 15061.0, 11530.0, 6175.0]
          w1299 = T13."Enabled" ("Disabled")
          w1301 = T13."Disabled and Grayed Out" ("Disabled")
          w1284 = "7.5.6" ("Test Paragraph")
          # "K16+Venable"
          # "Deg"
          # "K16 OFF + Venable"
          # "Venable"
          n631 = flat-sequence {
            tunnel: w1297 -> [_]
            frame #0 {
              "TempAlg" <- TRUE
            }
          }
          n632 = control-ref of="Pannel User Message"() -> (w1323:refnum<vi>)
          n633 = property class="Str"(reference=w1323, error in=w1297, "Value"="7.5.6.Temperature controle test") -> (error out=w1322:errorcluster)  [unwired: 1 out]
          n634 = property on="Start" class="Bool (strict)"(error in=w1297, "DisabledEnum"=w1301) -> (error out=w1302:errorcluster)  [unwired: 1 in, 1 out]
          n635 = call "Reset old test Values (SubVI).vi"("error in"=w1322, "Atr in"=w1285, "Test Paragraph"=w1284) -> ("error out"=w1286:errorcluster)  [unwired: 8 in]
          n636 = property on="Report" class="Bool (strict)"(error in=w1302, "DisabledEnum"=w1301) -> ()  [unwired: 1 in, 2 out]
          n637 = call "Table_ScrollaBarMarvin.vi"("error in"=w1286, "Line to focus"=w1284, "reference in"=w1285) -> ("error out"=w1343:errorcluster)  [unwired: 2 out]
          n638 = property class="Tbl (strict)"(reference=w1285, error in=w1343) -> (reference out=w1320:refnum<vi>, error out=w1342:errorcluster, "Value"=w1341:string[][])
          n639 = control-ref of="VISA resource name out"() -> (w1333:refnum<vi>)
          n640 = control-ref of="Config_CANAT"() -> (w1314:refnum<vi>)
          n641 = control-ref of="UUT"() -> (w1315:refnum<vi>)
          n642 = Byte Array To String(unsigned byte array=u8[] [75, 0, 4, 2, 0, 0, 0, 0] ("appended array")) -> (string=w1335:string)
          n643 = Index Array(array=w1341, index (col)=0 ("disabled index (col)")) -> (element=w1340:string[])  [unwired: 1 in]
          n644 = Byte Array To String(unsigned byte array=u8[] [75, 0, 4, 2, 0, 0, 2, 0] ("appended array")) -> (string=w1345:string)
          n645 = Byte Array To String(unsigned byte array=u8[] [75, 0, 4, 2, 0, 128, 2, 0] ("appended array")) -> (string=w1327:string)
          n646 = call "Find_Number_LineMARVIN.vi"("Test Paragraph"=w1284, "error in"=w1342, "Row Headers[]"=w1340) -> ("error out"=w1338:errorcluster, "Line number"=w1330:i32)  [unwired: 2 in, 2 out]
          n647 = call "Table_ScrollaBarMarvin.vi"("error in"=w1338, "Line to focus"=w1284, "reference in"=w1320) -> ("error out"=w1310:errorcluster)  [unwired: 2 out]
          n648 = call "CANSendMotorSpeed.vi"("Remote"=FALSE, "error in (no error)"=w1310, "Motor Speed RPM"=u16 0, "UUT"=w1315, "Cluster in"=w1314) -> ("error out"=w1309:errorcluster)  [unwired: 6 in]
          n649 = property class="VISAName"(reference=w1333, error in=w1309) -> (error out=w1346:errorcluster, "Value"=w1344:refnum<visa-resource-name>)  [unwired: 1 out]
          n650 = VISA Write(VISA resource name=w1344, write buffer=w1345, error in (no error)=w1346) -> (VISA resource name out=w1328:refnum<visa-resource-name>, error out=w1329:errorcluster)  [unwired: 1 out]
          n651 = call "Wait_Sec.vi"("Delay Time (sec)"=2.0, "error out"=w1329) -> ("error in"=w1325:errorcluster)  [unwired: 2 in]
          n652 = VISA Write(VISA resource name=w1328, write buffer=w1327, error in (no error)=w1325) -> (VISA resource name out=w1318:refnum<visa-resource-name>, error out=w1326:errorcluster)  [unwired: 1 out]
          n653 = call "Time Delay"("error in (no error)"=w1326) -> ("error out"=w1311:errorcluster)  [unwired: 10 in]
          n654 = while {
            tunnel: [w1367] -> w1293
            stop <- w1368 stop-if-true
            w1370 = 6050.0 ("y")
            n655 = Random Number (0-1)() -> (number: 0 to 1=w1371:dbl)
            n656 = Multiply(x=w1371, y=w1370) -> (x*y=w1367:dbl)
            n657 = In Range and Coerce(upper limit=w1370, x=w1367, lower limit=5950.0) -> (In Range?=w1368:bool)  [unwired: 1 out]
          }
          n658 = while {
            tunnel: [w1352] -> w1292
            stop <- w1353 stop-if-true
            w1355 = 11550.0 ("y")
            n659 = Random Number (0-1)() -> (number: 0 to 1=w1356:dbl)
            n660 = Multiply(x=w1356, y=w1355) -> (x*y=w1352:dbl)
            n661 = In Range and Coerce(upper limit=w1355, x=w1352, lower limit=11450.0) -> (In Range?=w1353:bool)  [unwired: 1 out]
          }
          n662 = while {
            tunnel: [w1362] -> w1291
            stop <- w1363 stop-if-true
            w1365 = 15050.0 ("y")
            n663 = Random Number (0-1)() -> (number: 0 to 1=w1366:dbl)
            n664 = Multiply(x=w1366, y=w1365) -> (x*y=w1362:dbl)
            n665 = In Range and Coerce(upper limit=w1365, x=w1362, lower limit=14950.0) -> (In Range?=w1363:bool)  [unwired: 1 out]
          }
          n666 = while {
            tunnel: [w1357] -> w1290
            stop <- w1358 stop-if-true
            w1360 = 11550.0 ("y")
            n667 = Random Number (0-1)() -> (number: 0 to 1=w1361:dbl)
            n668 = Multiply(x=w1361, y=w1360) -> (x*y=w1357:dbl)
            n669 = In Range and Coerce(upper limit=w1360, x=w1357, lower limit=11450.0) -> (In Range?=w1358:bool)  [unwired: 1 out]
          }
          n670 = while {
            tunnel: [w1347] -> w1289
            stop <- w1348 stop-if-true
            w1350 = 6050.0 ("y")
            n671 = Random Number (0-1)() -> (number: 0 to 1=w1351:dbl)
            n672 = Multiply(x=w1351, y=w1350) -> (x*y=w1347:dbl)
            n673 = In Range and Coerce(upper limit=w1350, x=w1347, lower limit=5950.0) -> (In Range?=w1348:bool)  [unwired: 1 out]
          }
          n674 = Build Array(w1293, w1292, w1291, w1290, w1289) -> (w1288:dbl[])
          n675 = To Unsigned Word Integer(number=w1288) -> (unsigned 16bit integer=w1287:u16[])
          n676 = for {
            tunnel: w1311 -> [w1414]
            tunnel: dbl[] [1202.0, 1288.0, 1472.0, 1472.0, 1379.0] -> [w1383] mode=indexing
            tunnel: dbl[] [200.0, 200.0, 400.0, 200.0, 200.0] -> [w1413] mode=indexing
            tunnel: w1330 -> [w1411]
            tunnel: w1320 -> [w1404]
            tunnel: w1320 -> [w1389]
            tunnel: [w1403] -> w1319
            tunnel: w1318 -> [w1384]
            tunnel: dbl[] [6000.0, 7000.0, 12200.0, 14500.0, 11100.0] -> [w1375] mode=indexing
            tunnel: dbl[] [50.0, 68.0, 88.0, 80.0, 60.0] -> [w1382] mode=indexing
            tunnel: dbl[] [6000.0, 11400.0, 14900.0, 11600.0, 6200.0] -> [w1380] mode=indexing
            tunnel: [w1377] -> w1306 mode=indexing
            tunnel: [w1376] -> w1305 mode=indexing
            tunnel: w1287 -> [w1374] mode=indexing
            tunnel: dbl[] [57.0, 67.0, 89.0, 79.0, 61.0] -> [w1373] mode=indexing
            i -> [w1379]
            w1395 = 6 ("disabled index (col)")
            n677 = disable-structure shown="Enabled" {
              disable-tunnel: w1414 -> [w1432 w1602]
              disable-tunnel: w1413 -> [w1431 _]
              disable-tunnel: [w1430 w1600] -> w1393
              disable-tunnel: w1384 -> [w1428 _]
              disable-tunnel: w1383 -> [w1427 _]
              disable-tunnel: w1382 -> [w1426 _]
              disable-tunnel: [w1424 w1602] -> w1381
              disable-tunnel: w1380 -> [w1423 _]
              disable-tunnel: w1379 -> [w1422 _]
              disable-tunnel: [w1420 w1601] -> w1378
              disable-tunnel: [w1419 w1603] -> w1377
              disable-tunnel: [w1418 w1603] -> w1376
              disable-tunnel: w1375 -> [w1415 _]
              disable-tunnel: w1374 -> [_ w1601]
              disable-tunnel: w1373 -> [_ w1600]
              frame Enabled {
                n678 = call <vilib>:"High Resolution Relative Seconds.vi"() -> ("relative seconds"=w1429:dbl)
                n679 = while {
                  tunnel: w1431 -> [w1511]
                  tunnel: w1432 -> [w1523]
                  tunnel: [w1506] -> w1416
                  tunnel: [w1491] -> w1421
                  tunnel: [w1509] -> w1419
                  tunnel: [w1499] -> w1430
                  tunnel: [w1498] -> w1418
                  tunnel: w1422 -> [w1500]
                  tunnel: w1429 -> [w1518]
                  tunnel: w1428 -> [w1514]
                  tunnel: w1415 -> [w1512]
                  shift-right: [w1513] -> _
                  shift-left: w1427 -> [w1497]
                  tunnel: w1426 -> [w1496]
                  shift-right: [w1488] -> _
                  shift-left: "" -> [w1495]
                  tunnel: [w1486] -> w1417
                  stop <- w1520 stop-if-true
                  n680 = control-ref of="Motor Speed RPM"() -> (w1522:refnum<vi>)
                  n681 = control-ref of="Ambient Temperature"() -> (w1524:refnum<vi>)
                  n682 = call <vilib>:"High Resolution Relative Seconds.vi"() -> ("relative seconds"=w1515:dbl)
                  n683 = call <vilib>:"High Resolution Relative Seconds.vi"() -> ("relative seconds"=w1519:dbl)
                  n684 = Subtract(x=w1519, y=w1518) -> (x-y=w1517:dbl)
                  n685 = Greater Or Equal?(x=w1517, y=180.0) -> (x >= y?=w1486:bool)
                  n686 = property on="Stop Button" class="Bool (strict)"() -> ("Value"=w1490:bool)  [unwired: 2 in, 2 out]
                  n687 = First Call?() -> (First Call?: T/F=w1487:bool)
                  n688 = case shown="0, 1, Default" w1500 {
                    tunnel: w1523 -> [w1572 w1579]
                    tunnel: [w1572 w1578] -> w1494
                    tunnel: w1514 -> [_ w1577]
                    tunnel: w1497 -> [_ w1576]
                    tunnel: [TRUE FALSE] -> w1510
                    frame 10 {
                    }
                    frame 0, 1, Default {
                      n689 = call "DegToDAC (SubVI).vi"("error in (no error)"=w1579, "R2"=0.0, "Numeric"=w1576) -> ("error out"=w1580:errorcluster, "output array"=w1575:u8[])  [unwired: 7 in]
                      n690 = Byte Array To String(unsigned byte array=w1575) -> (string=w1581:string)
                      n691 = VISA Write(VISA resource name=w1577, write buffer=w1581, error in (no error)=w1580) -> (error out=w1578:errorcluster)  [unwired: 2 out]
                    }
                  }
                  n692 = property class="DigNum (strict)"(reference=w1524, error in=w1494) -> (error out=w1521:errorcluster, "Value"=w1499:dbl)  [unwired: 1 out]
                  n693 = property class="DigNum (strict)"(reference=w1522, error in=w1521) -> (error out=w1493:errorcluster, "Value"=w1506:dbl)  [unwired: 1 out]
                  n694 = Number To Fractional String(number=w1499, precision (6)=i16 2) -> (F-format string=w1504:string)  [unwired: 2 in]
                  n695 = Number To Fractional String(number=w1506, precision (6)=i16 2) -> (F-format string=w1502:string)  [unwired: 2 in]
                  n696 = Concatenate Strings("\r\n", "Temp: " ("string"), w1504, "  Speed: " ("string"), w1502) -> (w1489:string)
                  n697 = case shown="True" w1487 {
                    tunnel: w1489 -> [w1525 _]
                    tunnel: [w1525 ""] -> w1488
                    frame False {
                    }
                    frame True {
                    }
                  }
                  n698 = case shown="1, 2" w1500 {
                    tunnel: w1499 -> [w1531 w1537 w1540]
                    tunnel: [w1532 w1538 w1541] -> w1498
                    tunnel: w1496 -> [w1530 w1533 _]
                    frame 3, 4 {
                      w1529 = 2.0 ("y")
                      n699 = Add(x=w1529, y=w1530) -> (x+y=w1528:dbl)
                      n700 = Subtract(x=w1530, y=w1529) -> (x-y=w1527:dbl)
                      n701 = In Range and Coerce(upper limit=w1528, x=w1531, lower limit=w1527) -> (In Range?=w1532:bool)  [unwired: 1 out]
                    }
                    frame 1, 2 {
                      w1536 = 2.0 ("y")
                      n702 = Add(x=w1536, y=w1533) -> (x+y=w1535:dbl)
                      n703 = Subtract(x=w1533, y=w1536) -> (x-y=w1534:dbl)
                      n704 = In Range and Coerce(upper limit=w1535, x=w1537, lower limit=w1534) -> (In Range?=w1538:bool)  [unwired: 1 out]
                    }
                    frame Default {
                      n705 = Less Or Equal?(x=w1540, y=65.0) -> (x <= y?=w1541:bool)
                    }
                  }
                  n706 = case shown="3, 4" w1500 {
                    tunnel: [w1547 w1564] -> w1509
                    tunnel: [w1551 w1568] -> w1513
                    tunnel: w1497 -> [w1550 w1567]
                    tunnel: w1506 -> [w1545 w1559]
                    tunnel: w1512 -> [w1544 w1563]
                    tunnel: w1511 -> [w1549 w1566]
                    tunnel: w1493 -> [w1543 w1557]
                    tunnel: [w1543 w1557] -> w1492
                    frame 0, 1, Default {
                      n707 = Add(x=10.0, y=w1550) -> (x+y=w1551:dbl)
                      n708 = Greater Or Equal?(x=w1545, y=w1544) -> (x >= y?=w1546:bool)
                      n709 = Add(x=w1544, y=w1549) -> (x+y=w1552:dbl)
                      n710 = Subtract(x=w1544, y=w1549) -> (x-y=w1553:dbl)
                      n711 = In Range and Coerce(upper limit=w1552, x=w1545, lower limit=w1553) -> (In Range?=w1542:bool)  [unwired: 1 out]
                      n712 = Compound Arithmetic op=OR(w1546, w1542) -> (w1547:bool)
                    }
                    frame 3, 4 {
                      n713 = Subtract(x=w1567, y=10.0 ("x")) -> (x-y=w1568:dbl)
                      n714 = Less Or Equal?(x=w1559, y=w1563) -> (x <= y?=w1561:bool)
                      n715 = Greater Or Equal?(x=w1559, y=5800.0) -> (x >= y?=w1560:bool)
                      n716 = property on="Stop Button" class="Bool (strict)"() -> ("Value"=w1556:bool)  [unwired: 2 in, 2 out]
                      n717 = Not(x=w1556) -> (.not. x?=w1555:bool)
                      n718 = Compound Arithmetic op=AND(w1561, w1560, w1555) -> (w1562:bool)
                      n719 = Add(x=w1563, y=w1566) -> (x+y=w1569:dbl)
                      n720 = Subtract(x=w1563, y=w1566) -> (x-y=w1570:dbl)
                      n721 = In Range and Coerce(upper limit=w1569, x=w1559, lower limit=w1570) -> (In Range?=w1554:bool)  [unwired: 1 out]
                      n722 = Compound Arithmetic op=OR(w1562, w1554) -> (w1564:bool)
                    }
                  }
                  n723 = while {
                    tunnel: w1492 -> [w1584]
                    tunnel: w1515 -> [w1598]
                    tunnel: [w1584] -> w1491
                    tunnel: w1495 -> [w1585]
                    stop <- w1583 stop-if-true
                    n724 = control-ref of="Pannel User Message"() -> (w1586:refnum<vi>)
                    n725 = property on="Stop Button" class="Bool (strict)"() -> ("Value"=w1582:bool)  [unwired: 2 in, 2 out]
                    n726 = call <vilib>:"High Resolution Relative Seconds.vi"() -> ("relative seconds"=w1599:dbl)
                    n727 = Subtract(x=w1599, y=w1598) -> (x-y=w1596:dbl)
                    n728 = Subtract(x=4.0, y=w1596) -> (x-y=w1591:dbl)
                    n729 = Less Or Equal To 0?(x=w1591) -> (x <= 0?=w1597:bool)
                    n730 = Compound Arithmetic op=OR(w1597, w1582) -> (w1583:bool)
                    n731 = Number To Fractional String(number=w1591, precision (6)=i16 2) -> (F-format string=w1593:string)  [unwired: 2 in]
                    n732 = Concatenate Strings("7.5.6.Temperature controle test" ("Value"), "\r\n", "Time to wait: " ("Value"), w1593, "  Sec." ("string"), w1585) -> (w1588:string)
                    n733 = property class="Str"(reference=w1586, "Value"=w1588) -> ()  [unwired: 1 in, 2 out]
                  }
                  n734 = Compound Arithmetic op=OR(w1509, w1510, w1486, w1490) -> (w1520:bool)
                }
                n735 = case shown="False" w1417 {
                  tunnel: [w1439 w1485] -> w1424
                  tunnel: w1423 -> [w1438 _]
                  tunnel: w1422 -> [w1437 _]
                  tunnel: w1421 -> [w1436 w1485]
                  tunnel: [w1433 w1484] -> w1420
                  tunnel: w1416 -> [_ w1484]
                  frame False {
                    n736 = while {
                      tunnel: w1435 -> [w1464]
                      tunnel: [w1463] -> w1439
                      tunnel: w1438 -> [w1462]
                      tunnel: w1437 -> [w1461]
                      tunnel: w1434 -> [w1456]
                      tunnel: [w1450] -> w1433
                      stop <- w1459 stop-if-true
                      w1446 = 120.0 ("y")
                      n737 = control-ref of="Motor Speed RPM"() -> (w1465:refnum<vi>)
                      n738 = control-ref of="Pannel User Message"() -> (w1455:refnum<vi>)
                      n739 = property class="DigNum (strict)"(reference=w1465, error in=w1464) -> (error out=w1463:errorcluster, "Value"=w1450:dbl)  [unwired: 1 out]
                      n740 = property on="Stop Button" class="Bool (strict)"() -> ("Value"=w1448:bool)  [unwired: 2 in, 2 out]
                      n741 = call <vilib>:"High Resolution Relative Seconds.vi"() -> ("relative seconds"=w1457:dbl)
                      n742 = Subtract(x=w1457, y=w1456) -> (x-y=w1445:dbl)
                      n743 = Number To Fractional String(number=w1450, precision (6)=i16 2) -> (F-format string=w1452:string)  [unwired: 2 in]
                      n744 = Subtract(x=w1446, y=w1445) -> (x-y=w1444:dbl)
                      n745 = Number To Fractional String(number=w1444, precision (6)=i16 2) -> (F-format string=w1442:string)  [unwired: 2 in]
                      n746 = Concatenate Strings("7.5.6.Temperature controle test\n" ("string"), "Motor speed [rpm]: " ("string"), w1452, "\nTimeout [sec]: " ("string"), w1442) -> (w1449:string)
                      n747 = property class="Str"(reference=w1455, "Value"=w1449) -> ()  [unwired: 1 in, 2 out]
                      n748 = Greater Or Equal?(x=w1445, y=w1446) -> (x >= y?=w1458:bool)
                      n749 = case shown="3, 4" w1461 {
                        tunnel: w1450 -> [w1467 w1473 w1479]
                        tunnel: [w1469 w1475 w1481] -> w1460
                        tunnel: w1462 -> [w1470 w1476 _]
                        frame 3, 4 {
                          n750 = Greater Or Equal?(x=w1467, y=5700.0) -> (x >= y?=w1468:bool)
                          n751 = Less Or Equal?(x=w1467, y=w1470) -> (x <= y?=w1471:bool)
                          n752 = And(x=w1468, y=w1471) -> (x .and. y?=w1469:bool)
                        }
                        frame 1, 2 {
                          n753 = Greater Or Equal?(x=w1473, y=w1476) -> (x >= y?=w1477:bool)
                          n754 = Less Or Equal?(x=w1473, y=15300.0) -> (x <= y?=w1474:bool)
                          n755 = And(x=w1477, y=w1474) -> (x .and. y?=w1475:bool)
                        }
                        frame Default {
                          n756 = Greater Or Equal?(x=w1479, y=5800.0) -> (x >= y?=w1483:bool)
                          n757 = Less Or Equal?(x=w1479, y=6200.0) -> (x <= y?=w1480:bool)
                          n758 = And(x=w1483, y=w1480) -> (x .and. y?=w1481:bool)
                        }
                      }
                      n759 = Compound Arithmetic op=OR(w1460, w1458, w1448) -> (w1459:bool)
                    }
                    n760 = flat-sequence {
                      tunnel: w1436 -> [w1441]
                      tunnel: [w1441] -> w1435
                      tunnel: [w1440] -> w1434
                      frame #0 {
                        n761 = call <vilib>:"High Resolution Relative Seconds.vi"() -> ("relative seconds"=w1440:dbl)
                      }
                    }
                  }
                  frame True {
                  }
                }
              }
              frame Disabled {
                w1603 = TRUE ("Boolean")
              }
            }
            n762 = Number To Fractional String(number=w1393, precision (6)=i16 2) -> (F-format string=w1400:string)  [unwired: 2 in]
            n763 = Number To Fractional String(number=w1378, precision (6)=i16 2) -> (F-format string=w1409:string)  [unwired: 2 in]
            n764 = Increment(x=w1411) -> (x+1=w1396:i32)
            n765 = Multiply(x=2, y=w1379) -> (x*y=w1412:i32)
            n766 = Add(x=w1396, y=w1412) -> (x+y=w1398:i32)
            n767 = call "PassOrFail (SubVI).vi"("disabled index (col)"=w1395, "index (row)"=w1398, "error in (no error)"=w1381, "Boolean"=w1377, "Table in"=w1389) -> ("error out"=w1408:errorcluster)  [unwired: 6 in]
            n768 = property class="Tbl (strict)"(reference=w1404, error in=w1408) -> (reference out=w1407:refnum<vi>, error out=w1391:errorcluster, "Value"=w1410:string[][])
            n769 = Replace Array Subset(array=w1410, new element=w1409, index (row)=w1398, index (col)=5 ("disabled index (col)")) -> (w1392:string[][])
            n770 = property class="Tbl (strict)"(reference=w1389, error in=w1391, "Value"=w1392) -> (reference out=w1387:refnum<vi>, error out=w1390:errorcluster)
            n771 = Increment(x=w1398) -> (x+1=w1394:i32)
            n772 = call "PassOrFail (SubVI).vi"("disabled index (col)"=w1395, "index (row)"=w1394, "error in (no error)"=w1390, "Boolean"=w1376, "Table in"=w1389) -> ("error out"=w1388:errorcluster)  [unwired: 6 in]
            n773 = property class="Tbl (strict)"(reference=w1387, error in=w1388) -> (error out=w1385:errorcluster, "Value"=w1386:string[][])  [unwired: 1 out]
            n774 = Replace Array Subset(array=w1386, new element=w1400, index (row)=w1394, index (col)=5 ("disabled index (col)")) -> (w1399:string[][])
            n775 = property class="Tbl (strict)"(reference=w1407, error in=w1385, "Value"=w1399) -> (error out=w1403:errorcluster)  [unwired: 1 out]
          }
          n776 = property class="VISAName"(reference=w1333, error in=w1319) -> (error out=w1298:errorcluster, "Value"=w1336:refnum<visa-resource-name>)  [unwired: 1 out]
          n777 = VISA Write(VISA resource name=w1336, write buffer=w1335, error in (no error)=w1298) -> ()  [unwired: 3 out]
          n778 = property on="Start" class="Bool (strict)"(error in=w1298, "DisabledEnum"=w1299) -> (error out=w1300:errorcluster)  [unwired: 1 in, 1 out]
          n779 = property on="Report" class="Bool (strict)"(error in=w1300, "DisabledEnum"=w1299) -> (error out=w1296:errorcluster)  [unwired: 1 in, 1 out]
          n780 = property on="TempAlg" class="Bool (strict)"(error in=w1296, "Value"=FALSE ("TempAlg")) -> ()  [unwired: 1 in, 2 out]
          n781 = Build Array (concatenate)(w1306, w1305) -> (w1304:bool[])
          n782 = And Array Elements(Boolean array=w1304) -> (logical AND=→"TempControlind":bool)
        }
        frame "Burn in" {
          w1613 = TRUE ("rpm")
          w1615 = FALSE ("PrintTime")
          w1631 = T13."Enabled" ("Disabled")
          w1634 = T13."Disabled and Grayed Out" ("Disabled")
          (unwired) "EP=1r\nVC=15100\r\n" ("write buffer")
          (unwired) dbl[] [60.0, 60.0, 60.0]
          w1699 = 13.0 ("y")
          w1698 = 25.0 ("x")
          w1697 = 2 ("disabled index (col)")
          w1704 = 6 ("disabled index (col)")
          w1723 = 400.0 ("y")
          w1722 = 15100.0 ("x")
          w1629 = "7.5.7.Burn-in test in process" ("Value")
          w1608 = "7.5.7" ("Test Paragraph")
          # "k16+Venable"
          # "K15 + Venable + 90deg OFF"
          # "Venable"
          n783 = Byte Array To String(unsigned byte array=u8[] [75, 0, 4, 2, 0, 0, 2, 0] ("appended array")) -> ()  [unwired: 1 out]
          n784 = property on="Start" class="Bool (strict)"(error in=w1633, "DisabledEnum"=w1634) -> (error out=w1635:errorcluster)  [unwired: 1 in, 1 out]
          n785 = property on="Report" class="Bool (strict)"(error in=w1635, "DisabledEnum"=w1634) -> (error out=w1606:errorcluster)  [unwired: 1 in, 1 out]
          n786 = control-ref of="Pannel User Message"() -> (w1731:refnum<vi>)
          n787 = Concatenate Strings(w1629, "\nFull speed operation" ("string")) -> (w1628:string)
          n788 = property class="Str"(reference=w1731, error in=w1606, "Value"=w1629) -> (reference out=w1620:refnum<vi>, error out=w1662:errorcluster)
          n789 = control-ref of="VISA resource name out"() -> (w1736:refnum<vi>)
          n790 = control-ref of="Stop Button"() -> (w1621:refnum<vi>)
          n791 = control-ref of="Config_CANAT"() -> (w1649:refnum<vi>)
          n792 = control-ref of="Config_CANAT"() -> (w1657:refnum<vi>)
          n793 = control-ref of="Config_CANAT"() -> (w1664:refnum<vi>)
          n794 = control-ref of="UUT"() -> (w1650:refnum<vi>)
          n795 = control-ref of="Power transistor Heat sink Temp."() -> (w1700:refnum<vi>)
          n796 = control-ref of="UUT"() -> (w1656:refnum<vi>)
          n797 = control-ref of="UUT"() -> (w1665:refnum<vi>)
          n798 = control-ref of="Motor Speed RPM"() -> (w1729:refnum<vi>)
          n799 = control-ref of="Motor Speed RPM"() -> (w1614:refnum<vi>)
          n800 = Byte Array To String(unsigned byte array=u8[] [75, 0, 4, 2, 0, 0, 0, 0] ("appended array")) -> (string=w1739:string)
          n801 = Add(x=w1722, y=w1723) -> (x+y=w1724:dbl)
          n802 = Add(x=w1698, y=w1699) -> (x+y=w1701:dbl)
          n803 = property on="UUT" class="Str"() -> ("Value"=w1612:string)  [unwired: 2 in, 2 out]
          n804 = Equal?(x=w1612, y="EBAY") -> (x = y?=w1610:bool)
          n805 = case shown="False" w1610 {
            tunnel: [28.0 ("x") 50.0 ("x")] -> w1715
            tunnel: [5.0 ("y") 7.0 ("y")] -> w1714
            frame False {
            }
            frame True {
            }
          }
          n806 = Add(x=w1715, y=w1714) -> (x+y=w1713:dbl)
          n807 = Subtract(x=w1722, y=w1723) -> (x-y=w1725:dbl)
          n808 = Subtract(x=w1698, y=w1699) -> (x-y=w1702:dbl)
          n809 = Byte Array To String(unsigned byte array=u8[] [75, 0, 4, 2, 0, 0, 2, 0] ("appended array")) -> (string=w1750:string)
          n810 = Subtract(x=w1715, y=w1714) -> (x-y=w1712:dbl)
          n811 = property on="CurrentOffset" class="DigNum (strict)"() -> ("Value"=w1642:dbl)  [unwired: 2 in, 2 out]
          n812 = disable-structure shown="Enabled" {
            disable-tunnel: w1665 -> [w1857 _]
            disable-tunnel: w1664 -> [w1856 _]
            disable-tunnel: u16 0 ("Motor Speed RPM") -> [w1854 _]
            disable-tunnel: w1662 -> [w1853 w1858]
            disable-tunnel: [w1852 w1858] -> w1661
            frame Disabled {
              n813 = call "CANSendMotorSpeed.vi"("Remote"=FALSE, "error in (no error)"=w1853, "Motor Speed RPM"=w1854, "UUT"=w1857, "Cluster in"=w1856) -> ("error out"=w1852:errorcluster)  [unwired: 6 in]
            }
            frame Enabled {
            }
          }
          n814 = call "Reset old test Values (SubVI).vi"("error in"=w1661, "Atr in"=w1607, "Test Paragraph"=w1608) -> ("error out"=w1609:errorcluster)  [unwired: 8 in]
          n815 = call "Table_ScrollaBarMarvin.vi"("error in"=w1609, "Line to focus"=w1608, "reference in"=w1607) -> ("error out"=w1748:errorcluster)  [unwired: 2 out]
          n816 = property class="Tbl (strict)"(reference=w1607, error in=w1748) -> (reference out=w1678:refnum<vi>, error out=w1747:errorcluster, "Value"=w1746:string[][])
          n817 = Index Array(array=w1746, index (col)=0 ("disabled index (col)")) -> (element=w1745:string[])  [unwired: 1 in]
          n818 = call "Find_Number_LineMARVIN.vi"("Test Paragraph"=w1608, "error in"=w1747, "Row Headers[]"=w1745) -> ("error out"=w1743:errorcluster, "Line number"=w1717:i32)  [unwired: 2 in, 2 out]
          n819 = call "Table_ScrollaBarMarvin.vi"("error in"=w1743, "Line to focus"=w1608, "reference in"=w1678) -> ("error out"=w1742:errorcluster)  [unwired: 2 out]
          n820 = property class="VISAName"(reference=w1736, error in=w1742) -> (error out=w1751:errorcluster, "Value"=w1749:refnum<visa-resource-name>)  [unwired: 1 out]
          n821 = VISA Write(VISA resource name=w1749, write buffer=w1750, error in (no error)=w1751) -> (VISA resource name out=w1734:refnum<visa-resource-name>, error out=w1735:errorcluster)  [unwired: 1 out]
          n822 = call "Wait_Sec.vi"("Delay Time (sec)"=0.0, "error out"=w1735) -> ("error in"=w1645:errorcluster)  [unwired: 2 in]
          n823 = property class="DigNum (strict)"(reference=w1700, error in=w1645) -> (error out=w1644:errorcluster, "Value"=w1693:dbl)  [unwired: 1 out]
          n824 = In Range and Coerce(upper limit=w1701, x=w1693, lower limit=w1702) -> (In Range?=w1639:bool)  [unwired: 1 out]
          n825 = Number To Fractional String(number=w1693, precision (6)=i16 2) -> (F-format string=w1708:string)  [unwired: 2 in]
          n826 = call "Write panel message (SubVI).vi"("rpm"=w1614, "Stop"=w1621, "error in (no error)"=w1644, "Time to wait"=10.0 ("Delay Time (sec)"), "Strin"=w1629, "String in"=w1620) -> ("error out"=w1659:errorcluster)  [unwired: 5 in]
          n827 = call "CANSendMotorSpeed.vi"("Remote"=TRUE, "error in (no error)"=w1659, "Motor Speed RPM"=u16 15100, "UUT"=w1656, "Cluster in"=w1657) -> ("error out"=w1658:errorcluster)  [unwired: 6 in]
          n828 = call "Write panel message (SubVI).vi"(4:"rpm"=w1614, 5:"rpm"=w1613, "PrintTime"=w1615, "Stop"=w1621, "error in (no error)"=w1658, "Time to wait"=30.0 ("Delay Time (sec)"), "Strin"=w1628, "String in"=w1620) -> ("error out"=w1728:errorcluster)  [unwired: 3 in]
          n829 = call "Write panel message (SubVI).vi"(4:"rpm"=w1614, 5:"rpm"=w1613, "PrintTime"=w1615, "Stop"=w1621, "error in (no error)"=w1728, "Time to wait"=1.0, "Strin"="7.5.7.Burn-in test in process.\nDC current measure.", "String in"=w1620) -> ("error out"=w1622:errorcluster)  [unwired: 3 in]
          n830 = Add(x=w1693, y=25.0) -> (x+y=w1687:dbl)
          n831 = Number To Fractional String(number=w1687, precision (6)=i16 2) -> (F-format string=w1691:string)  [unwired: 2 in]
          n832 = Concatenate Strings("< " ("string"), w1691) -> (w1690:string)
          n833 = Increment(x=w1717) -> (x+1=w1705:i32)
          n834 = Increment(x=w1705) -> (x+1=w1703:i32)
          n835 = Increment(x=w1703) -> (x+1=w1684:i32)
          n836 = Increment(x=w1684) -> (x+1=w1696:i32)
          n837 = Increment(x=w1696) -> (x+1=w1695:i32)
          n838 = Increment(x=w1695) -> (x+1=w1683:i32)
          n839 = for {
            N: 10 -> [_]
            tunnel: w1734 -> [w1777]
            tunnel: [w1768] -> w1617 mode=indexing
            tunnel: w1622 -> [w1776]
            tunnel: [w1769] -> w1726
            stop <- w1766 stop-if-true
            # "Get Current by ADC (2)"
            n840 = flat-sequence {
              tunnel: w1772 -> [w1779]
              tunnel: [w1779] -> w1771
              tunnel: [w1778] -> w1770
              frame #0 {
                n841 = call <vilib>:"High Resolution Relative Seconds.vi"() -> ("relative seconds"=w1778:dbl)
              }
            }
            n842 = Byte Array To String(unsigned byte array=u8[] [75, 0, 4, 17, 0, 0, 0, 0] ("appended array")) -> (string=w1775:string)
            n843 = call "Time Delay8"("error in (no error)"=w1776) -> ("error out"=w1767:errorcluster)  [unwired: 10 in]
            n844 = VISA Write(VISA resource name=w1777, write buffer=w1775, error in (no error)=w1767) -> (VISA resource name out=w1773:refnum<visa-resource-name>, error out=w1772:errorcluster)  [unwired: 1 out]
            n845 = while {
              tunnel: w1773 -> [w1792]
              tunnel: w1771 -> [w1791]
              tunnel: [w1790] -> _
              tunnel: [w1789] -> w1769
              tunnel: w1770 -> [w1787]
              tunnel: [w1781] -> w1768
              stop <- w1783 stop-if-true
              n846 = call <vilib>:"High Resolution Relative Seconds.vi"() -> ("relative seconds"=w1788:dbl)
              n847 = Subtract(x=w1788, y=w1787) -> (x-y=w1786:dbl)
              n848 = Greater Or Equal?(x=w1786, y=10.0) -> (x >= y?=w1784:bool)
              n849 = property on="Stop Button" class="Bool (strict)"() -> ("Value"=w1780:bool)  [unwired: 2 in, 2 out]
              n850 = VISA Read(VISA resource name=w1792, byte count=u32 1, error in (no error)=w1791) -> (VISA resource name out=w1794:refnum<visa-resource-name>, read buffer=w1795:string, error out=w1793:errorcluster)  [unwired: 1 out]
              n851 = String To Byte Array(string=w1795) -> (unsigned byte array=w1798:u8[])
              n852 = Index Array(array=w1798, index=0) -> (element=w1796:u8)
              n853 = case shown="75" w1796 {
                tunnel: [w1803 w1807] -> w1789
                tunnel: w1794 -> [w1802 w1816]
                tunnel: w1793 -> [w1803 w1815]
                tunnel: [w1802 w1808] -> w1790
                tunnel: [u32 9999 w1805] -> w1781
                tunnel: [FALSE w1804] -> w1782
                frame 0, Default {
                }
                frame 75 {
                  n854 = VISA Read(VISA resource name=w1816, byte count=u32 3, error in (no error)=w1815) -> (VISA resource name out=w1811:refnum<visa-resource-name>, read buffer=w1819:string, error out=w1810:errorcluster)  [unwired: 1 out]
                  n855 = String To Byte Array(string=w1819) -> (unsigned byte array=w1809:u8[])
                  n856 = Index Array(array=w1809, index #1=0 ("index")) -> (element #1=w1814:u8, element #2=w1812:u8)  [unwired: 2 in, 1 out]
                  n857 = Equal?(x=u8 0, y=w1814) -> (x = y?=w1813:bool)
                  n858 = case shown="True" w1813 {
                    tunnel: [w1822 w1829] -> w1807
                    tunnel: w1812 -> [_ w1836]
                    tunnel: w1811 -> [w1823 w1835]
                    tunnel: w1810 -> [w1822 w1834]
                    tunnel: w1809 -> [_ w1833]
                    tunnel: [w1823 w1831] -> w1808
                    tunnel: [u32 9999 w1825] -> w1805
                    tunnel: [FALSE w1824] -> w1804
                    frame False {
                    }
                    frame True {
                      n859 = VISA Read(VISA resource name=w1835, byte count=w1836, error in (no error)=w1834) -> (VISA resource name out=w1831:refnum<visa-resource-name>, read buffer=w1830:string, error out=w1829:errorcluster)  [unwired: 1 out]
                      n860 = String To Byte Array(string=w1830) -> (unsigned byte array=w1832:u8[])
                      n861 = Insert Into Array(array=w1833, new element=w1832) -> (w1826:u8[])  [unwired: 1 in]
                      n862 = Index Array(array=w1826, index #1=0 ("index")) -> (element #3=w1827:u8)  [unwired: 2 in, 2 out]
                      n863 = case shown="15..19" w1827 {
                        tunnel: w1826 -> [_ w1850]
                        tunnel: [u32 9999 w1839] -> w1825
                        tunnel: [FALSE w1840] -> w1824
                        frame 0, Default {
                        }
                        frame 15..19 {
                          n864 = Index Array(array=w1850, index #1=3 ("index")) -> (element #1=w1849:u8, element #2=w1848:u8, element #3=w1847:u8, element #4=w1846:u8)  [unwired: 3 in]
                          n865 = Join Numbers(hi=w1846, lo=w1847) -> ((hi.lo)=w1844:u16)
                          n866 = Join Numbers(hi=w1848, lo=w1849) -> ((hi.lo)=w1845:u16)
                          n867 = Join Numbers(hi=w1844, lo=w1845) -> ((hi.lo)=w1842:u32)
                          n868 = Multiply(x=0.02003173828125, y=w1842) -> (x*y=w1839:dbl)
                          n869 = Greater Or Equal?(x=w1839, y=40.0) -> (x >= y?=w1840:bool)
                        }
                      }
                    }
                  }
                }
              }
              n870 = Compound Arithmetic op=OR(w1780, w1784, w1782) -> (w1783:bool)
            }
            n871 = property on="Stop Button" class="Bool (strict)"() -> ("Value"=w1766:bool)  [unwired: 2 in, 2 out]
          }
          n872 = call <vilib>:"Clear Errors.vi"("error in (no error)"=w1726) -> ("error out"=w1653:errorcluster)  [unwired: 5 in, 1 out]
          n873 = property class="DigNum (strict)"(reference=w1729, error in=w1653) -> (error out=w1646:errorcluster, "Value"=w1688:dbl)  [unwired: 1 out]
          n874 = In Range and Coerce(upper limit=w1724, x=w1688, lower limit=w1725) -> (In Range?=w1640:bool)  [unwired: 1 out]
          n875 = Number To Fractional String(number=w1688, precision (6)=i16 2) -> (F-format string=w1709:string)  [unwired: 2 in]
          n876 = property class="Tbl (strict)"(reference=w1678, error in=w1646) -> (reference out=w1716:refnum<vi>, error out=w1673:errorcluster, "Value"=w1721:string[][])
          n877 = for {
            tunnel: w1617 -> [_] mode=indexing
            shift-right: [w1756] -> w1616
            shift-left: w1617 -> [w1759]
            n878 = Search 1D Array(1D array=w1759, element=9999.0) -> (index of element=w1757:i32)  [unwired: 1 in]
            n879 = Greater Or Equal To 0?(x=w1757) -> (x >= 0?=w1758:bool)
            n880 = case shown="True" w1758 {
              tunnel: w1759 -> [w1761 w1764]
              tunnel: w1757 -> [_ w1763]
              tunnel: [w1761 w1762] -> w1756
              frame False {
              }
              frame True {
                n881 = Delete From Array(array=w1764, length=1, index=w1763) -> (deleted portion=w1762:dbl[])  [unwired: 1 out]
              }
            }
          }
          n882 = Add Array Elements(numeric array=w1616) -> (sum=w1625:dbl)
          n883 = Divide(x=w1625, y=10.0) -> (x/y=w1624:dbl)
          n884 = Subtract(x=w1624, y=w1642) -> (x-y=w1643:dbl)
          n885 = In Range and Coerce(upper limit=w1713, x=w1643, lower limit=w1712) -> (In Range?=w1638:bool)  [unwired: 1 out]
          n886 = Number To Fractional String(number=w1643, precision (6)=i16 2) -> (F-format string=w1720:string)  [unwired: 2 in]
          n887 = Replace Array Subset(array=w1721, new element=w1720, index (row)=w1705, index (col)=5 ("disabled index (col)")) -> (w1681:string[][])
          n888 = property class="Tbl (strict)"(reference=w1678, error in=w1673, "Value"=w1681) -> (reference out=w1680:refnum<vi>, error out=w1672:errorcluster)
          n889 = call "PassOrFail (SubVI).vi"("disabled index (col)"=w1704, "index (row)"=w1705, "error in (no error)"=w1672, "Boolean"=w1638, "Table in"=w1716) -> ("error out"=w1671:errorcluster)  [unwired: 6 in]
          n890 = property class="Tbl (strict)"(reference=w1680, error in=w1671) -> (reference out=w1676:refnum<vi>, error out=w1670:errorcluster, "Value"=w1679:string[][])
          n891 = Replace Array Subset(array=w1679, new element=w1709, index (row)=w1703, index (col)=5 ("disabled index (col)")) -> (w1677:string[][])
          n892 = property class="Tbl (strict)"(reference=w1676, error in=w1670, "Value"=w1677) -> (reference out=w1675:refnum<vi>, error out=w1669:errorcluster)
          n893 = call "PassOrFail (SubVI).vi"("disabled index (col)"=w1704, "index (row)"=w1703, "error in (no error)"=w1669, "Boolean"=w1640, "Table in"=w1678) -> ("error out"=w1668:errorcluster)  [unwired: 6 in]
          n894 = property class="Tbl (strict)"(reference=w1675, error in=w1668) -> (error out=w1667:errorcluster, "Value"=w1674:string[][])  [unwired: 1 out]
          n895 = Replace Array Subset(array=w1674, new element #1=w1708, index (row) #1=w1684, index (col) #1=5 ("disabled index (col)"), new element #2=w1690, index (row) #2=w1696, index (col) #2=w1697, new element #3=w1690, index (row) #3=w1695, index (col) #3=w1697, new element #4=w1690, index (row) #4=w1683, index (col) #4=w1697) -> (w1706:string[][])
          n896 = property class="Tbl (strict)"(reference=w1678, error in=w1667, "Value"=w1706) -> (error out=w1666:errorcluster)  [unwired: 1 out]
          n897 = call "PassOrFail (SubVI).vi"("disabled index (col)"=w1704, "index (row)"=w1684, "error in (no error)"=w1666, "Boolean"=w1639, "Table in"=w1678) -> ("error out"=w1605:errorcluster)  [unwired: 6 in]
          n898 = property on="Stop Burn-in" class="Bool"(error in=w1605, "Visible"=TRUE) -> (error out=w1604:errorcluster)  [unwired: 1 in, 1 out]
          n899 = for {
            tunnel: w1604 -> [w1883]
            tunnel: dbl[] [600.0, 600.0, 600.0] -> [w1880] mode=indexing
            tunnel: w1687 -> [w1877]
            tunnel: w1684 -> [w1874]
            tunnel: w1607 -> [w1868]
            tunnel: [w1860] -> w1648
            tunnel: [w1859] -> w1641 mode=indexing
            i -> [w1873]
            n900 = control-ref of="Power transistor Heat sink Temp."() -> (w1879:refnum<vi>)
            n901 = while {
              tunnel: w1882 -> [w1902]
              tunnel: w1881 -> [w1905]
              tunnel: w1880 -> [w1896]
              tunnel: [w1893] -> w1878
              stop <- w1892 stop-if-true
              w1890 = i16 2 ("precision (6)")
              n902 = control-ref of="Pannel User Message"() -> (w1901:refnum<vi>)
              n903 = call <vilib>:"High Resolution Relative Seconds.vi"() -> ("relative seconds"=w1906:dbl)
              n904 = property on="Stop Button" class="Bool (strict)"() -> ("Value"=w1891:bool)  [unwired: 2 in, 2 out]
              n905 = Subtract(x=w1906, y=w1905) -> (x-y=w1895:dbl)
              n906 = Greater Or Equal?(x=w1895, y=w1896) -> (x >= y?=w1904:bool)
              n907 = Compound Arithmetic op=OR(w1891, "Stop Burn-in", w1904) -> (w1892:bool)
              n908 = Subtract(x=w1896, y=w1895) -> (x-y=w1897:dbl)
              n909 = Number To Fractional String(number=w1897, precision (6)=i16 2) -> (F-format string=w1898:string)  [unwired: 2 in]
              n910 = property on="Power transistor Heat sink Temp." class="DigNum (strict)"() -> ("Value"=w1889:dbl)  [unwired: 2 in, 2 out]
              n911 = Number To Fractional String(number=w1889, precision (6)=w1890) -> (F-format string=w1886:string)  [unwired: 2 in]
              n912 = property on="Motor Speed RPM" class="DigNum (strict)"() -> ("Value"=w1888:dbl)  [unwired: 2 in, 2 out]
              n913 = Number To Fractional String(number=w1888, precision (6)=w1890) -> (F-format string=w1884:string)  [unwired: 2 in]
              n914 = Concatenate Strings("Remained Time: " ("string"), w1898, "\nPCB Temp. [Deg]: " ("string"), w1886, "\nMotor speed [rpm]: " ("string"), w1884) -> (w1894:string)
              n915 = property class="Str"(reference=w1901, error in=w1902, "Value"=w1894) -> (error out=w1893:errorcluster)  [unwired: 1 out]
            }
            n916 = Increment(x=w1873) -> (x+1=w1872:i32)
            n917 = Add(x=w1874, y=w1872) -> (x+y=w1866:i32)
            n918 = flat-sequence {
              tunnel: [w1907] -> _
              tunnel: [w1907] -> w1882
              tunnel: [w1908] -> w1881
              tunnel: w1883 -> [w1907]
              frame #0 {
                n919 = call <vilib>:"High Resolution Relative Seconds.vi"() -> ("relative seconds"=w1908:dbl)
              }
            }
            n920 = property class="DigNum (strict)"(reference=w1879, error in=w1878) -> (error out=w1869:errorcluster, "Value"=w1870:dbl)  [unwired: 1 out]
            n921 = Less Or Equal?(x=w1870, y=w1877) -> (x <= y?=w1859:bool)
            n922 = property class="Tbl (strict)"(reference=w1868, error in=w1869) -> (reference out=w1863:refnum<vi>, error out=w1862:errorcluster, "Value"=w1865:string[][])
            n923 = Number To Fractional String(number=w1870, precision (6)=i16 2) -> (F-format string=w1871:string)  [unwired: 2 in]
            n924 = Replace Array Subset(array=w1865, new element=w1871, index (row)=w1866, index (col)=5 ("disabled index (col)")) -> (w1864:string[][])
            n925 = property class="Tbl (strict)"(reference=w1863, error in=w1862, "Value"=w1864) -> (error out=w1861:errorcluster)  [unwired: 1 out]
            n926 = call "PassOrFail (SubVI).vi"("disabled index (col)"=6, "index (row)"=w1866, "error in (no error)"=w1861, "Boolean"=w1859, "Table in"=w1863) -> ("error out"=w1860:errorcluster)  [unwired: 6 in]
          }
          n927 = call "CANSendMotorSpeed.vi"("Remote"=FALSE, "error in (no error)"=w1648, "Motor Speed RPM"=u16 0, "UUT"=w1650, "Cluster in"=w1649) -> ("error out"=w1647:errorcluster)  [unwired: 6 in]
          n928 = property on="Stop Burn-in" class="Bool"(error in=w1647, "Visible"=FALSE) -> (error out=w1630:errorcluster)  [unwired: 1 in, 1 out]
          n929 = property class="VISAName"(reference=w1736, error in=w1630) -> (error out=w1738:errorcluster, "Value"=w1740:refnum<visa-resource-name>)  [unwired: 1 out]
          n930 = VISA Write(VISA resource name=w1740, write buffer=w1739, error in (no error)=w1738) -> ()  [unwired: 3 out]
          n931 = property on="Start" class="Bool (strict)"(error in=w1630, "DisabledEnum"=w1631) -> (error out=w1632:errorcluster)  [unwired: 1 in, 1 out]
          n932 = property on="Report" class="Bool (strict)"(error in=w1632, "DisabledEnum"=w1631) -> ()  [unwired: 1 in, 2 out]
          n933 = Build Array (concatenate)(w1641, w1640, w1639, w1638) -> (w1637:bool[])
          n934 = And Array Elements(Boolean array=w1637) -> (logical AND=→"Burninind":bool)
        }
        frame "Visual Inspec" {
          w1912 = T13."Enabled" ("Disabled")
          w1915 = T13."Disabled and Grayed Out" ("Disabled")
          n935 = property on="Start" class="Bool (strict)"(error in=w1914, "DisabledEnum"=w1915) -> (error out=w1916:errorcluster)  [unwired: 1 in, 1 out]
          n936 = property on="Report" class="Bool (strict)"(error in=w1916, "DisabledEnum"=w1915) -> (error out=w1913:errorcluster)  [unwired: 1 in, 1 out]
          n937 = call "VisualInspection.vi"("error in (no error)"=w1913, "TableRef"=w1918) -> ("error out"=w1910:errorcluster, "VisualInspectionResult"=w1917:bool)  [unwired: 8 in]
          "VisualInspectionResult" <- w1917
          n938 = property on="Automation" class="Bool (strict)"() -> ("Value"=w1909:bool)  [unwired: 2 in, 2 out]
          n939 = case shown="True" w1909 {
            tunnel: w1917 -> [_ w1919]
            frame False {
            }
            frame True {
              n940 = property on="SetSN" class="Bool (strict)"("Val(Sgnl)"=w1919) -> ()  [unwired: 2 in, 2 out]
            }
          }
          n941 = property on="Start" class="Bool (strict)"(error in=w1910, "DisabledEnum"=w1912) -> (error out=w1911:errorcluster)  [unwired: 1 in, 1 out]
          n942 = property on="Report" class="Bool (strict)"(error in=w1911, "DisabledEnum"=w1912) -> ()  [unwired: 1 in, 2 out]
        }
        frame "Temp Sens Cal" {
          w1951 = T13."Enabled" ("Disabled")
          w1955 = T13."Disabled and Grayed Out" ("Disabled")
          w1930 = "7.5.5.Temperature sensor calibration test in process..." ("Value")
          w1935 = FALSE ("Clear Log")
          w1922 = "7.5.5" ("Test Paragraph")
          # "K15 OFF + Venable"
          # "K15 OFF + Venable"
          n943 = property on="Start" class="Bool (strict)"(error in=w1954, "DisabledEnum"=w1955) -> (error out=w1956:errorcluster)  [unwired: 1 in, 1 out]
          n944 = property on="Report" class="Bool (strict)"(error in=w1956, "DisabledEnum"=w1955) -> (error out=w1953:errorcluster)  [unwired: 1 in, 1 out]
          n945 = VISA Flush I/O Buffer(VISA resource name=w1959, error in (no error)=w1953) -> (VISA resource name out=w1938:refnum<visa-resource-name>, error out=w1958:errorcluster)  [unwired: 1 in]
          n946 = control-ref of="VISA resource name out"() -> (w1946:refnum<vi>)
          n947 = control-ref of="Config_CANAT"() -> (w1925:refnum<vi>)
          n948 = control-ref of="UUT"() -> (w1926:refnum<vi>)
          n949 = control-ref of="Pannel User Message"() -> (w1961:refnum<vi>)
          n950 = Byte Array To String(unsigned byte array=u8[] [75, 0, 4, 2, 0, 0, 0, 0] ("appended array")) -> (string=w1940:string)
          n951 = Concatenate Strings("EP=1\r\nAO" ("string"), "[", "1" ("string"), "]=0", "\r\n" ("write buffer")) -> (w1965:string)
          n952 = Byte Array To String(unsigned byte array=u8[] [75, 0, 4, 2, 0, 0, 16, 0] ("appended array")) -> (string=w1947:string)
          n953 = property class="Str"(reference=w1961, error in=w1958, "Value"=w1930) -> (error out=w1960:errorcluster)  [unwired: 1 out]
          n954 = call "Reset old test Values (SubVI).vi"("error in"=w1960, "Atr in"=w1921, "Test Paragraph"=w1922) -> ("error out"=w1923:errorcluster)  [unwired: 8 in]
          n955 = call "Table_ScrollaBarMarvin.vi"("error in"=w1923, "Line to focus"=w1922, "reference in"=w1921) -> ("error out"=w1972:errorcluster)  [unwired: 2 out]
          n956 = property class="Tbl (strict)"(reference=w1921, error in=w1972) -> (error out=w1974:errorcluster, "Value"=w1975:string[][])  [unwired: 1 out]
          n957 = Index Array(array=w1975, index (col)=0 ("disabled index (col)")) -> (element=w1976:string[])  [unwired: 1 in]
          n958 = call "Find_Number_LineMARVIN.vi"("Test Paragraph"=w1922, "error in"=w1974, "Row Headers[]"=w1976) -> ("error out"=w1971:errorcluster, "Line number"=w1969:i32)  [unwired: 2 in, 2 out]
          n959 = property on="Serial" class="Bool (strict)"(error in=w1971) -> (error out=w1964:errorcluster, "Value"=w1970:bool)  [unwired: 1 in, 1 out]
          n960 = call "CANSendMotorSpeed.vi"("Remote"=TRUE, "error in (no error)"=w1964, "Motor Speed RPM"=u16 0, "UUT"=w1926, "Cluster in"=w1925) -> ("error out"=w1929:errorcluster)  [unwired: 6 in]
          n961 = call "Time Delay13"("error in (no error)"=w1929) -> ("error out"=w1924:errorcluster)  [unwired: 10 in]
          n962 = call "SerialMarvinMod.vi"("error in (no error)"=w1924, "Clear Log"=w1935, "write buffer"=w1965, "VISA resource name"=w1938) -> ("error out"=w1944:errorcluster)  [unwired: 6 in, 1 out]
          n963 = property class="VISAName"(reference=w1946, error in=w1944) -> (error out=w1948:errorcluster, "Value"=w1949:refnum<visa-resource-name>)  [unwired: 1 out]
          n964 = VISA Write(VISA resource name=w1949, write buffer=w1947, error in (no error)=w1948) -> (VISA resource name out=w1939:refnum<visa-resource-name>, error out=w1942:errorcluster)  [unwired: 1 out]
          n965 = call "Time Delay6"("error in (no error)"=w1942) -> ("error out"=w1941:errorcluster)  [unwired: 10 in]
          n966 = VISA Write(VISA resource name=w1939, write buffer=w1940, error in (no error)=w1941) -> (error out=w1936:errorcluster)  [unwired: 2 out]
          n967 = call "SerialMarvinMod.vi"("error in (no error)"=w1936, "Clear Log"=w1935, "write buffer"="AO[1]\r\n", "VISA resource name"=w1938) -> ("error out"=w1920:errorcluster, "read buffer"=w1934:string)  [unwired: 6 in]
          n968 = Equal?(x=w1934, y="") -> (x = y?=w1931:bool)
          n969 = And(x=w1970, y=w1931) -> (x .and. y?=w1932:bool)
          n970 = case shown="True" w1932 {
            selector: w1932 -> [w1978 _]
            tunnel: w1920 -> [w1983 _]
            tunnel: w1921 -> [w1982 w2019]
            tunnel: w1969 -> [w1981 w2018]
            tunnel: w1938 -> [_ w2022]
            tunnel: [w1978 w2010] -> w1957
            tunnel: [w1977 w1989] -> w1950
            tunnel: w1930 -> [_ w2007]
            tunnel: w1920 -> [_ w2006]
            frame False {
              n971 = flat-sequence {
                tunnel: w1983 -> [w1984]
                tunnel: [w1984] -> w1977
                frame #0 {
                  n972 = One Button Dialog(message="Please establish RS connection.") -> ()  [unwired: 1 in, 1 out]
                }
              }
              n973 = Increment(x=w1981) -> (x+1=w1980:i32)
              n974 = call "PassOrFail (SubVI).vi"("disabled index (col)"=6, "index (row)"=w1980, "error in (no error)"=w1977, "Boolean"=w1978, "Table in"=w1982) -> ()  [unwired: 6 in, 1 out]
            }
            frame True {
              (unwired) dbl[] [0.68545] ("Val 2")
              (unwired) dbl[] [0.69103] ("Val 2")
              (unwired) u32[] [2048]
              # "Max"
              n975 = for {
                tunnel: u32[] [64, 512, 2048, 8192] -> [w2095] mode=indexing
                tunnel: w2022 -> [w2124]
                tunnel: dbl[] [0.59774, 0.65238, 0.68545, 0.71584] ("Val 2") -> [w2084] mode=indexing
                tunnel: [w2081] -> w2057 mode=indexing
                tunnel: [w2123] -> w2051
                tunnel: [w2099] -> w2002
                tunnel: [w2081] -> w2016 mode=indexing
                tunnel: [w2122] -> w2013 mode=indexing
                tunnel: dbl[] [0.60155, 0.65733, 0.69103, 0.72203] ("Val 2") -> [w2120] mode=indexing
                tunnel: [w2121] -> w2009 mode=indexing
                tunnel: [w2118] -> w2008 mode=indexing
                tunnel: w2007 -> [w2117]
                tunnel: w2006 -> [w2090]
                n976 = control-ref of="VISA resource name out"() -> (w2109:refnum<vi>)
                n977 = control-ref of="Stop Button"() -> (w2115:refnum<vi>)
                n978 = control-ref of="Motor Speed RPM"() -> (w2116:refnum<vi>)
                n979 = control-ref of="Pannel User Message"() -> (w2114:refnum<vi>)
                n980 = To Unsigned Long Integer(number=w2095) -> (unsigned 32bit integer=w2106:u32)
                n981 = Split Number(x=w2106) -> (hi(x)=w2101:u16, lo(x)=w2100:u16)
                n982 = Split Number(x=w2100) -> (hi(x)=w2102:u8, lo(x)=w2103:u8)
                n983 = Split Number(x=w2101) -> (hi(x)=w2104:u8, lo(x)=w2105:u8)
                n984 = Build Array(u8 75, u8 0 ("element"), u8 4 ("Length"), u8 2, w2103, w2102, w2105, w2104) -> (w2107:u8[])
                n985 = Byte Array To String(unsigned byte array=w2107) -> (string=w2108:string)
                n986 = call "Write panel message (SubVI).vi"("rpm"=w2116, "PrintTime"=FALSE, "Stop"=w2115, "error in (no error)"=w2090, "Time to wait"=0.1, "Strin"="7.5.5.Temperature sensor calibration test in process...", "String in"=w2114) -> ("error out"=w2113:errorcluster)  [unwired: 4 in]
                n987 = property class="VISAName"(reference=w2109, error in=w2113) -> (error out=w2110:errorcluster, "Value"=w2099:refnum<visa-resource-name>)  [unwired: 1 out]
                n988 = VISA Flush I/O Buffer(VISA resource name=w2099, error in (no error)=w2110) -> (VISA resource name out=w2112:refnum<visa-resource-name>, error out=w2111:errorcluster)  [unwired: 1 in]
                n989 = VISA Write(VISA resource name=w2112, write buffer=w2108, error in (no error)=w2111) -> (error out=w2089:errorcluster)  [unwired: 2 out]
                n990 = call "Time Delay3"("error in (no error)"=w2089) -> ("error out"=w2088:errorcluster)  [unwired: 10 in]
                n991 = while {
                  tunnel: w2124 -> [w2158]
                  tunnel: [w2128] -> _
                  tunnel: [w2156] -> w2122
                  tunnel: [w2126] -> w2087
                  tunnel: w2084 -> [w2127]
                  tunnel: [w2143] -> w2121
                  tunnel: w2120 -> [w2144]
                  tunnel: [w2157] -> w2123
                  shift-right: [w2136] -> w2118
                  shift-left: 0.0 -> [w2137]
                  tunnel: w2117 -> [w2134]
                  tunnel: w2088 -> [w2130]
                  tunnel: [w2129] -> w2086 mode=indexing
                  i -> [w2141]
                  stop <- w2142 stop-if-true
                  n992 = control-ref of="Stop Button"() -> (w2132:refnum<vi>)
                  n993 = control-ref of="Motor Speed RPM"() -> (w2131:refnum<vi>)
                  n994 = control-ref of="Pannel User Message"() -> (w2133:refnum<vi>)
                  n995 = Equal?(x=w2141, y=10) -> (x = y?=w2139:bool)
                  n996 = property on="Stop Button" class="Bool (strict)"() -> ("Value"=w2138:bool)  [unwired: 2 in, 2 out]
                  n997 = Compound Arithmetic op=OR(w2138, w2139) -> (w2142:bool)
                  n998 = Concatenate Strings("TA" ("string"), "[", "Index", "]", "\r\n" ("write buffer")) -> (w2150:string)
                  n999 = call "Write panel message (SubVI).vi"("rpm"=w2131, "PrintTime"=FALSE, "Stop"=w2132, "error in (no error)"=w2130, "Time to wait"=0.5 ("Delay Time (sec)"), "Strin"=w2134, "String in"=w2133) -> ("error out"=w2148:errorcluster)  [unwired: 4 in]
                  n1000 = call "SerialMarvinMod.vi"("error in (no error)"=w2148, "Clear Log"=FALSE, "write buffer"=w2150, "VISA resource name"=w2158) -> ("error out"=w2157:errorcluster, "read buffer"=w2156:string)  [unwired: 6 in]
                  n1001 = Fract/Exp String To Number(string=w2156) -> (number=w2129:dbl)  [unwired: 3 in, 1 out]
                  n1002 = Subtract(x=w2129, y=w2127) -> (x-y=w2128:dbl)
                  n1003 = Multiply(x=w2127, y=0.015) -> (x*y=w2145:dbl)
                  n1004 = Subtract(x=w2127, y=w2145) -> (x-y=w2143:dbl)
                  n1005 = In Range and Coerce(upper limit=w2144, x=w2129, lower limit=w2143) -> (In Range?=w2125:bool)  [unwired: 1 out]
                  n1006 = case shown="True" w2125 {
                    tunnel: w2129 -> [w2160 w2163]
                    tunnel: [w2159 w2162] -> w2126
                    tunnel: w2137 -> [w2161 w2164]
                    tunnel: [w2159 w2162] -> w2136
                    frame False {
                      n1007 = Max & Min(x=w2161, y=w2160) -> (max(x,y)=w2159:dbl)  [unwired: 1 out]
                    }
                    frame True {
                      n1008 = Max & Min(x=w2164, y=w2163) -> (max(x,y)=w2162:dbl)  [unwired: 1 out]
                    }
                  }
                }
                n1009 = Add Array Elements(numeric array=w2086) -> (sum=w2085:dbl)
                n1010 = Divide(x=w2085, y=11.0 ("x")) -> (x/y=w2083:dbl)
                n1011 = Subtract(x=w2087, y=w2084) -> ()  [unwired: 1 out]
                n1012 = Subtract(x=w2083, y=w2084) -> (x-y=w2081:dbl)
              }
              "Array 2" <- w2016
              "Array 3" <- w2013
              "Array 4" <- w2009
              "Array 5" <- w2008
              n1013 = control-ref of="Stop Button"() -> (w2001:refnum<vi>)
              n1014 = control-ref of="Motor Speed RPM"() -> (w1999:refnum<vi>)
              n1015 = control-ref of="Pannel User Message"() -> (w2000:refnum<vi>)
              n1016 = To Unsigned Long Integer(number=u32 0) -> (unsigned 32bit integer=w2039:u32)
              n1017 = Split Number(x=w2039) -> (hi(x)=w2045:u16, lo(x)=w2046:u16)
              n1018 = Split Number(x=w2046) -> (hi(x)=w2044:u8, lo(x)=w2043:u8)
              n1019 = Add Array Elements(numeric array=w2057) -> (sum=w2056:dbl)
              n1020 = Divide(x=w2056, y=4.0) -> (x/y=w2015:dbl)
              n1021 = In Range and Coerce(upper limit=0.1, x=w2015, lower limit=-0.1) -> (In Range?=w2011:bool)  [unwired: 1 out]
              n1022 = And(x=w2011, y=w2011) -> (x .and. y?=w2010:bool)
              n1023 = Number To Fractional String(number=w2015, precision (6)=i16 7) -> (F-format string=w2014:string)  [unwired: 2 in]
              n1024 = Concatenate Strings("EP=1\r\nAO" ("string"), "[", "1" ("string"), "]=", w2014, "\r\n" ("write buffer")) -> (w2025:string)
              n1025 = Increment(x=w2018) -> (x+1=w2030:i32)
              n1026 = call "PassOrFail (SubVI).vi"("disabled index (col)"=6, "index (row)"=w2030, "error in (no error)"=w2051, "Boolean"=w2011, "Table in"=w2019) -> ("error out"=w2032:errorcluster)  [unwired: 6 in]
              n1027 = property class="Tbl (strict)"(reference=w2019, error in=w2032) -> (reference out=w2036:refnum<vi>, error out=w2035:errorcluster, "Value"=w2033:string[][])
              n1028 = Number To Fractional String(number=w2015, precision (6)=i16 4) -> (F-format string=w2020:string)  [unwired: 2 in]
              n1029 = Replace Array Subset(array=w2033, new element=w2020, index (row)=w2030, index (col)=5 ("disabled index (col)")) -> (w2034:string[][])
              n1030 = property class="Tbl (strict)"(reference=w2036, error in=w2035, "Value"=w2034) -> (error out=w1992:errorcluster)  [unwired: 1 out]
              n1031 = case shown="True" w2011 {
                tunnel: w2025 -> [_ w2069]
                tunnel: w1992 -> [w2059 w2068]
                tunnel: w2022 -> [w2058 w2063]
                tunnel: ["0" ("read buffer") w2061] -> w2021
                tunnel: [w2059 w2065] -> w1991
                frame False {
                  n1032 = VISA Flush I/O Buffer(VISA resource name=w2058, error in (no error)=w2059) -> ()  [unwired: 1 in, 2 out]
                }
                frame True {
                  n1033 = call "SerialMarvinMod.vi"("error in (no error)"=w2068, "Clear Log"=FALSE, "write buffer"=w2069, "VISA resource name"=w2063) -> ("error out"=w2067:errorcluster)  [unwired: 6 in, 1 out]
                  n1034 = disable-structure shown="Enabled" {
                    disable-tunnel: w2067 -> [w2077 w2080]
                    disable-tunnel: [w2074 w2078] -> w2065
                    disable-tunnel: "AO[1]\r\n" ("write buffer") -> [w2073 _]
                    disable-tunnel: w2063 -> [w2072 w2079]
                    disable-tunnel: FALSE ("Clear Log") -> [w2071 _]
                    disable-tunnel: [w2070 _] -> w2061
                    frame Disabled {
                      n1035 = call "Time Delay4"("error in (no error)"=w2077) -> ("error out"=w2076:errorcluster)  [unwired: 10 in]
                      n1036 = call "SerialMarvinMod.vi"("error in (no error)"=w2076, "Clear Log"=w2071, "write buffer"=w2073, "VISA resource name"=w2072) -> ("error out"=w2075:errorcluster)  [unwired: 6 in, 1 out]
                      n1037 = call "SerialMarvinMod.vi"("error in (no error)"=w2075, "Clear Log"=w2071, "write buffer"=w2073, "VISA resource name"=w2072) -> ("error out"=w2074:errorcluster, "read buffer"=w2070:string)  [unwired: 6 in]
                    }
                    frame Enabled {
                      n1038 = VISA Flush I/O Buffer(VISA resource name=w2079, error in (no error)=w2080) -> (error out=w2078:errorcluster)  [unwired: 1 in, 1 out]
                    }
                  }
                }
              }
              n1039 = Equal?(x=w2014, y=w2021) -> ()  [unwired: 1 out]
              n1040 = Split Number(x=w2045) -> (hi(x)=w2042:u8, lo(x)=w2041:u8)
              n1041 = Build Array(u8 75, u8 0 ("element"), u8 4 ("Length"), u8 2, w2043, w2044, w2041, w2042) -> (w2037:u8[])
              n1042 = Byte Array To String(unsigned byte array=w2037) -> (string=w2050:string)
              n1043 = Byte Array To String(unsigned byte array=u8[] [75, 0, 4, 2, 0, 0, 16, 0] ("appended array")) -> (string=w2005:string)
              n1044 = VISA Write(VISA resource name=w2002, write buffer=w2005, error in (no error)=w1991) -> (error out=w2003:errorcluster)  [unwired: 2 out]
              n1045 = call <vilib>:"Clear Errors.vi"("error in (no error)"=w2003) -> ("error out"=w1996:errorcluster)  [unwired: 5 in, 1 out]
              n1046 = call "Write panel message (SubVI).vi"(4:"rpm"=w1999, 5:"rpm"=FALSE ("rpm"), "PrintTime"=TRUE, "Stop"=w2001, "error in (no error)"=w1996, "Time to wait"=15.0, "Strin"="7.5.5.Temperature sensor calibration test in process...", "String in"=w2000) -> ("error out"=w1993:errorcluster)  [unwired: 3 in]
              n1047 = VISA Write(VISA resource name=w2002, write buffer=w2050, error in (no error)=w1993) -> (error out=w1990:errorcluster)  [unwired: 2 out]
              n1048 = call <vilib>:"Clear Errors.vi"("error in (no error)"=w1990) -> ("error out"=w1989:errorcluster)  [unwired: 5 in, 1 out]
              n1049 = call "PassOrFail (SubVI).vi"("disabled index (col)"=6, "index (row)"=w2018, "error in (no error)"=w1989, "Boolean"=w2011, "Table in"=w2019) -> ()  [unwired: 6 in, 1 out]
            }
          }
          "TempSensCalind" <- w1957
          n1050 = property on="Start" class="Bool (strict)"(error in=w1950, "DisabledEnum"=w1951) -> (error out=w1952:errorcluster)  [unwired: 1 in, 1 out]
          n1051 = property on="Report" class="Bool (strict)"(error in=w1952, "DisabledEnum"=w1951) -> ()  [unwired: 1 in, 2 out]
        }
        frame "Auxiliary" {
          w2172 = T13."Enabled" ("Disabled")
          w2176 = T13."Disabled and Grayed Out" ("Disabled")
          w2169 = "8.Auxiliary test" ("Value")
          w2167 = "8" ("Test Paragraph")
          # "K20 OFF"
          # "K20 ON"
          # "OFF"
          n1052 = property on="Start" class="Bool (strict)"(error in=w2175, "DisabledEnum"=w2176) -> (error out=w2177:errorcluster)  [unwired: 1 in, 1 out]
          n1053 = property on="Report" class="Bool (strict)"(error in=w2177, "DisabledEnum"=w2176) -> (error out=w2174:errorcluster)  [unwired: 1 in, 1 out]
          n1054 = control-ref of="Pannel User Message"() -> (w2191:refnum<vi>)
          n1055 = property class="Str"(reference=w2191, error in=w2174, "Value"=w2169) -> (reference out=w2170:refnum<vi>, error out=w2190:errorcluster)
          n1056 = control-ref of="VISA resource name out"() -> (w2194:refnum<vi>)
          n1057 = Build Array(u8[] [75, 0, 4, 2, 0, 0, 8, 0] ("appended array"), u8[] [75, 0, 4, 2, 0, 0, 0, 0] ("appended array")) -> (w2186:u8[][])
          n1058 = Byte Array To String(unsigned byte array=u8[] [75, 0, 4, 2, 0, 0, 0, 0] ("appended array")) -> (string=w2196:string)
          n1059 = call "Reset old test Values (SubVI).vi"("error in"=w2190, "Atr in"=w2166, "Test Paragraph"=w2167) -> ("error out"=w2168:errorcluster)  [unwired: 8 in]
          n1060 = call "Table_ScrollaBarMarvin.vi"("error in"=w2168, "Line to focus"=w2167, "reference in"=w2166) -> ("error out"=w2204:errorcluster)  [unwired: 2 out]
          n1061 = property class="Tbl (strict)"(reference=w2166, error in=w2204) -> (reference out=w2185:refnum<vi>, error out=w2203:errorcluster, "Value"=w2202:string[][])
          n1062 = Index Array(array=w2202, index (col)=0 ("disabled index (col)")) -> (element=w2201:string[])  [unwired: 1 in]
          n1063 = call "Find_Number_LineMARVIN.vi"("Test Paragraph"=w2167, "error in"=w2203, "Row Headers[]"=w2201) -> ("error out"=w2199:errorcluster, "Line number"=w2189:i32)  [unwired: 2 in, 2 out]
          n1064 = call "Table_ScrollaBarMarvin.vi"("error in"=w2199, "Line to focus"=w2167, "reference in"=w2185) -> ("error out"=w2198:errorcluster)  [unwired: 2 out]
          n1065 = property class="VISAName"(reference=w2194, error in=w2198) -> (error out=w2182:errorcluster, "Value"=w2205:refnum<visa-resource-name>)  [unwired: 1 out]
          n1066 = call "Wait_Sec.vi"("Delay Time (sec)"=2.0, "error out"=w2182) -> ("error in"=w2193:errorcluster)  [unwired: 2 in]
          n1067 = call <vilib>:"Clear Errors.vi"("error in (no error)"=w2193) -> ("error out"=w2165:errorcluster)  [unwired: 5 in, 1 out]
          n1068 = for {
            tunnel: w2205 -> [w2262]
            tunnel: w2165 -> [w2260]
            tunnel: w2186 -> [w2256] mode=indexing
            tunnel: w2185 -> [w2242]
            tunnel: w2189 -> [w2245]
            tunnel: [w2243] -> w2184
            tunnel: dbl[] [0.3, 1.7] -> [w2228] mode=indexing
            tunnel: [w2211] -> w2181 mode=indexing
            tunnel: [w2210] -> w2180 mode=indexing
            tunnel: w2170 -> [w2221]
            tunnel: w2169 -> [w2219]
            i -> [w2226]
            stop <- w2213 stop-if-true
            w2249 = 6 ("disabled index (col)")
            n1069 = control-ref of="Stop Button"() -> (w2220:refnum<vi>)
            n1070 = control-ref of="Motor Speed RPM"() -> (w2216:refnum<vi>)
            n1071 = property on="Stop Button" class="Bool (strict)"() -> ("Value"=w2214:bool)  [unwired: 2 in, 2 out]
            n1072 = Equal To 0?(x=w2226) -> (x = 0?=w2225:bool)
            n1073 = Select(t="Please turn-on heat gun." ("Message"), s=w2225, f="Please turn-off heat gun." ("Message")) -> ()  [unwired: 1 out]
            n1074 = Byte Array To String(unsigned byte array=w2256) -> (string=w2261:string)
            n1075 = VISA Write(VISA resource name=w2262, write buffer=w2261, error in (no error)=w2260) -> (VISA resource name out=w2257:refnum<visa-resource-name>, error out=w2259:errorcluster)  [unwired: 1 out]
            n1076 = while {
              tunnel: w2206 -> [w2331]
              tunnel: w2257 -> [w2330]
              tunnel: w2255 -> [w2319]
              tunnel: [w2287] -> w2241
              tunnel: [w2278] -> w2244
              tunnel: w2226 -> [w2318]
              tunnel: [w2317] -> w2211
              tunnel: [w2297] -> w2210
              tunnel: w2228 -> [w2316]
              tunnel: w2226 -> [w2276]
              tunnel: w2221 -> [w2309]
              tunnel: w2220 -> [w2308]
              tunnel: w2219 -> [w2305]
              shift-right: [w2295] -> _
              shift-left: 0.0 ("Value") -> [w2294]
              tunnel: w2216 -> [w2291]
              shift-right: [w2284] -> _
              shift-left: 0.0 ("Value") -> [w2285]
              shift-right: [w2277] -> _
              shift-left: 0.0 ("Value") -> [w2279]
              shift-right: [w2282] -> _
              shift-left: 0.0 ("Value") -> [w2281]
              tunnel: [w2283] -> w2208
              tunnel: w2206 -> [w2280]
              stop <- w2313 stop-if-true
              w2298 = 500.0 ("y")
              # "Get Ebay fan by ADC (3)"
              n1077 = control-ref of="Power transistor Heat sink Temp."() -> (w2320:refnum<vi>)
              n1078 = call <vilib>:"High Resolution Relative Seconds.vi"() -> ("relative seconds"=w2321:dbl)
              n1079 = Byte Array To String(unsigned byte array=u8[] [75, 0, 4, 18, 0, 0, 0, 0] ("appended array")) -> (string=w2329:string)
              n1080 = VISA Write(VISA resource name=w2330, write buffer=w2329, error in (no error)=w2319) -> (VISA resource name out=w2314:refnum<visa-resource-name>, error out=w2315:errorcluster)  [unwired: 1 out]
              n1081 = property on="Stop Button" class="Bool (strict)"() -> ("Value"=w2311:bool)  [unwired: 2 in, 2 out]
              n1082 = Subtract(x=w2321, y=w2331) -> (x-y=w2293:dbl)
              n1083 = Subtract(x=w2298, y=w2293) -> (x-y=w2303:dbl)
              n1084 = Number To Fractional String(number=w2303, precision (6)=i16 2) -> (F-format string=w2302:string)  [unwired: 2 in]
              n1085 = Greater Or Equal?(x=w2293, y=w2298) -> (x >= y?=w2312:bool)
              n1086 = VISA Read(VISA resource name=w2314, byte count=u32 1, error in (no error)=w2315) -> (VISA resource name out=w2323:refnum<visa-resource-name>, read buffer=w2324:string, error out=w2322:errorcluster)  [unwired: 1 out]
              n1087 = String To Byte Array(string=w2324) -> (unsigned byte array=w2327:u8[])
              n1088 = Index Array(array=w2327, index=0) -> (element=w2325:u8)
              n1089 = case shown="75" w2325 {
                tunnel: [w2432 w2438] -> w2286
                tunnel: w2323 -> [_ w2446]
                tunnel: w2322 -> [w2432 w2445]
                tunnel: [FALSE w2436] -> w2297
                tunnel: [u32 9999 w2435] -> _
                tunnel: w2316 -> [_ w2434]
                tunnel: w2276 -> [_ w2433]
                frame 0, Default {
                }
                frame 75 {
                  n1090 = VISA Read(VISA resource name=w2446, byte count=u32 3, error in (no error)=w2445) -> (VISA resource name out=w2441:refnum<visa-resource-name>, read buffer=w2449:string, error out=w2440:errorcluster)  [unwired: 1 out]
                  n1091 = String To Byte Array(string=w2449) -> (unsigned byte array=w2439:u8[])
                  n1092 = Index Array(array=w2439, index #1=0 ("index")) -> (element #1=w2444:u8, element #2=w2442:u8)  [unwired: 2 in, 1 out]
                  n1093 = Equal?(x=u8 0, y=w2444) -> (x = y?=w2443:bool)
                  n1094 = case shown="True" w2443 {
                    tunnel: [w2452 w2460] -> w2438
                    tunnel: w2442 -> [_ w2466]
                    tunnel: w2441 -> [_ w2465]
                    tunnel: w2440 -> [w2452 w2464]
                    tunnel: w2439 -> [_ w2463]
                    tunnel: [FALSE w2455] -> w2436
                    tunnel: [u32 9999 w2456] -> w2435
                    tunnel: w2434 -> [_ w2454]
                    tunnel: w2433 -> [_ w2453]
                    frame False {
                    }
                    frame True {
                      n1095 = VISA Read(VISA resource name=w2465, byte count=w2466, error in (no error)=w2464) -> (read buffer=w2461:string, error out=w2460:errorcluster)  [unwired: 2 out]
                      n1096 = String To Byte Array(string=w2461) -> (unsigned byte array=w2462:u8[])
                      n1097 = Insert Into Array(array=w2463, new element=w2462) -> (w2457:u8[])  [unwired: 1 in]
                      n1098 = Index Array(array=w2457, index #1=0 ("index")) -> (element #3=w2458:u8)  [unwired: 2 in, 2 out]
                      n1099 = case shown="15..19" w2458 {
                        tunnel: w2457 -> [_ w2481]
                        tunnel: [u32 9999 w2472] -> w2456
                        tunnel: [FALSE w2471] -> w2455
                        tunnel: w2454 -> [_ w2470]
                        tunnel: w2453 -> [_ w2469]
                        frame 0, Default {
                        }
                        frame 15..19 {
                          n1100 = Index Array(array=w2481, index #1=3 ("index")) -> (element #1=w2480:u8, element #2=w2479:u8, element #3=w2478:u8, element #4=w2477:u8)  [unwired: 3 in]
                          n1101 = Join Numbers(hi=w2477, lo=w2478) -> ((hi.lo)=w2475:u16)
                          n1102 = Join Numbers(hi=w2479, lo=w2480) -> ((hi.lo)=w2476:u16)
                          n1103 = Join Numbers(hi=w2475, lo=w2476) -> ((hi.lo)=w2473:u32)
                          n1104 = Multiply(x=0.0008056640625, y=w2473) -> (x*y=w2472:dbl)
                          n1105 = case shown="0, Default" w2469 {
                            tunnel: w2472 -> [w2485 w2487]
                            tunnel: [w2484 w2486] -> w2471
                            tunnel: w2470 -> [w2483 w2488]
                            frame 0, Default {
                              n1106 = Less Or Equal?(x=w2485, y=w2483) -> (x <= y?=w2484:bool)
                            }
                            frame 1 {
                              n1107 = Greater Or Equal?(x=w2487, y=w2488) -> (x >= y?=w2486:bool)
                            }
                          }
                        }
                      }
                    }
                  }
                }
              }
              n1108 = property class="DigNum (strict)"(reference=w2320, error in=w2286) -> (error out=w2288:errorcluster, "Value"=w2278:dbl)  [unwired: 1 out]
              n1109 = Number To Fractional String(number=w2278, precision (6)=i16 2) -> (F-format string=w2299:string)  [unwired: 2 in]
              n1110 = Concatenate Strings(w2305, "\nTimeout [sec]: " ("string"), w2302, "\nTemperature [Deg.]: " ("string"), w2299) -> (w2307:string)
              n1111 = call "Write panel message (SubVI).vi"(4:"rpm"=w2291, 5:"rpm"=FALSE ("rpm"), "PrintTime"=FALSE, "Stop"=w2308, "Time to wait"=0.2, "Strin"=w2307, "String in"=w2309) -> ()  [unwired: 4 in, 1 out]
              n1112 = case shown="0, Default" w2318 {
                tunnel: [w2401 w2426] -> w2317
                tunnel: w2278 -> [w2408 w2428]
                tunnel: w2297 -> [w2412 w2425]
                tunnel: [w2398 w2424] -> w2296
                tunnel: [w2408 0.0 ("Value")] -> w2295
                tunnel: w2294 -> [w2409 _]
                tunnel: w2293 -> [w2405 _]
                tunnel: [w2403 FALSE] -> w2292
                tunnel: w2288 -> [w2402 w2421]
                tunnel: [w2402 w2421] -> w2287
                tunnel: w2285 -> [w2400 w2420]
                tunnel: [w2399 w2420] -> w2284
                frame 0, Default {
                  n1113 = In Range and Coerce(upper limit=63.0, x=w2408, lower limit=58.0 ("y")) -> (In Range?=w2401:bool)  [unwired: 1 out]
                  n1114 = Less Or Equal?(x=w2408, y=w2409) -> (x <= y?=w2407:bool)
                  n1115 = Greater?(x=w2405, y=200.0) -> (0:w2406:bool)
                  n1116 = And(x=w2407, y=w2406) -> (x .and. y?=w2403:bool)
                  n1117 = Compound Arithmetic op=AND(w2401, w2412) -> (w2411:bool)
                  n1118 = case shown="True" w2401 {
                    tunnel: w2400 -> [_ w2419]
                    tunnel: [0.0 ("Value") w2418] -> w2399
                    tunnel: [FALSE w2416] -> w2397
                    frame False {
                    }
                    frame True {
                      n1119 = Increment(x=w2419) -> (x+1=w2418:dbl)
                      n1120 = Greater?(x=w2418, y=15.0) -> (0:w2416:bool)
                    }
                  }
                  n1121 = Or(x=w2397, y=w2411) -> (x .or. y?=w2398:bool)
                }
                frame 1 {
                  n1122 = In Range and Coerce(upper limit=57.0, x=w2428, lower limit=53.0 ("y")) -> (In Range?=w2426:bool)  [unwired: 1 out]
                  n1123 = Compound Arithmetic op=AND(w2426, w2425) -> (w2424:bool)
                }
              }
              n1124 = case shown="0, Default" w2276 {
                tunnel: [w2339 FALSE] -> w2283
                tunnel: [w2338 w2394] -> w2282
                tunnel: w2281 -> [w2337 w2394]
                tunnel: w2280 -> [w2336 _]
                tunnel: w2279 -> [w2335 w2396]
                tunnel: w2278 -> [w2334 _]
                tunnel: [w2333 w2396] -> w2277
                frame 0, Default {
                  n1125 = disable-structure shown="Enabled" {
                    disable-tunnel: w2335 -> [w2344 w2373]
                    disable-tunnel: w2334 -> [w2343 w2381]
                    disable-tunnel: [w2342 w2380] -> w2339
                    disable-tunnel: [w2341 w2379] -> w2338
                    disable-tunnel: w2337 -> [w2340 w2377]
                    disable-tunnel: w2336 -> [_ _]
                    disable-tunnel: w2334 -> [_ w2375]
                    disable-tunnel: [_ w2374] -> w2333
                    frame Disabled {
                      n1126 = case shown="0, Default" {
                        selector: _ -> [_ _]
                        tunnel: w2344 -> [w2349 w2363]
                        tunnel: w2343 -> [w2348 w2362]
                        tunnel: w2340 -> [w2352 w2364]
                        tunnel: [w2351 w2365] -> w2342
                        tunnel: [w2350 w2366] -> w2341
                        frame 0, Default {
                          n1127 = Subtract(x=w2348, y=w2349) -> (x-y=w2345:dbl)
                          n1128 = Greater?(x=w2345, y=1.0) -> (0:w2346:bool)
                          n1129 = case shown="False" w2346 {
                            tunnel: w2352 -> [w2356 _]
                            tunnel: [w2355 0.0 ("upper limit")] -> w2350
                            tunnel: [w2353 FALSE] -> w2351
                            frame False {
                              n1130 = Increment(x=w2356) -> (x+1=w2355:dbl)
                              n1131 = Greater Or Equal?(x=w2355, y=60.0) -> (x >= y?=w2353:bool)
                            }
                            frame True {
                            }
                          }
                        }
                        frame 1 {
                          n1132 = Subtract(x=w2363, y=w2362) -> (x-y=w2361:dbl)
                          n1133 = Greater?(x=w2361, y=1.0) -> (0:w2359:bool)
                          n1134 = case shown="False" w2359 {
                            tunnel: w2364 -> [w2370 _]
                            tunnel: [w2369 0.0 ("upper limit")] -> w2366
                            tunnel: [w2367 FALSE] -> w2365
                            frame False {
                              n1135 = Increment(x=w2370) -> (x+1=w2369:dbl)
                              n1136 = Greater Or Equal?(x=w2369, y=60.0) -> (x >= y?=w2367:bool)
                            }
                            frame True {
                            }
                          }
                        }
                      }
                    }
                    frame Enabled {
                      n1137 = Greater Or Equal?(x=w2377, y=200.0) -> (x >= y?=w2376:bool)
                      n1138 = case shown="False" w2376 {
                        tunnel: w2381 -> [_ w2393]
                        tunnel: w2373 -> [_ w2392]
                        tunnel: [FALSE w2388] -> w2380
                        frame False {
                        }
                        frame True {
                          n1139 = Subtract(x=w2393, y=w2392) -> (x-y=w2391:dbl)
                          n1140 = Greater Or Equal?(x=w2391, y=1.0) -> (x >= y?=w2389:bool)
                          n1141 = Not(x=w2389) -> (.not. x?=w2388:bool)
                        }
                      }
                      n1142 = case shown="False" w2376 {
                        tunnel: [w2384 0.0] -> w2379
                        tunnel: w2377 -> [w2383 _]
                        tunnel: w2375 -> [_ w2385]
                        tunnel: [w2382 w2385] -> w2374
                        tunnel: w2373 -> [w2382 _]
                        frame False {
                          n1143 = Increment(x=w2383) -> (x+1=w2384:dbl)
                        }
                        frame True {
                        }
                      }
                    }
                  }
                }
                frame 1 {
                }
              }
              n1144 = Compound Arithmetic op=OR(w2292, w2296, w2312, w2311, w2283) -> (w2313:bool)
            }
            n1145 = Number To Fractional String(number=w2244, precision (6)=i16 2) -> (F-format string=w2253:string)  [unwired: 2 in]
            n1146 = flat-sequence {
              tunnel: w2222 -> [w2490]
              tunnel: [w2490] -> w2255
              tunnel: [w2489] -> w2206
              frame #0 {
                n1147 = call <vilib>:"High Resolution Relative Seconds.vi"() -> ("relative seconds"=w2489:dbl)
              }
            }
            n1148 = call "Write panel message (SubVI).vi"("rpm"=w2216, "PrintTime"=FALSE, "Stop"=w2220, "error in (no error)"=w2259, "Time to wait"=10.0 ("Delay Time (sec)"), "Strin"=w2219, "String in"=w2221) -> ("error out"=w2222:errorcluster)  [unwired: 4 in]
            n1149 = Multiply(x=w2226, y=2) -> (x*y=w2238:i32)
            n1150 = Increment(x=w2238) -> (x+1=w2239:i32)
            n1151 = Add(x=w2245, y=w2239) -> (x+y=w2240:i32)
            n1152 = call "PassOrFail (SubVI).vi"("disabled index (col)"=w2249, "index (row)"=w2240, "error in (no error)"=w2241, "Boolean"=w2211, "Table in"=w2242) -> ("error out"=w2252:errorcluster)  [unwired: 6 in]
            n1153 = property class="Tbl (strict)"(reference=w2242, error in=w2252) -> (reference out=w2233:refnum<vi>, error out=w2231:errorcluster, "Value"=w2254:string[][])
            n1154 = Replace Array Subset(array=w2254, new element=w2253, index (row)=w2240, index (col)=5 ("disabled index (col)")) -> (w2236:string[][])
            n1155 = property class="Tbl (strict)"(reference=w2233, error in=w2231, "Value"=w2236) -> (reference out=w2234:refnum<vi>, error out=w2230:errorcluster)
            n1156 = Increment(x=w2240) -> (x+1=w2250:i32)
            n1157 = call "PassOrFail (SubVI).vi"("disabled index (col)"=w2249, "index (row)"=w2250, "error in (no error)"=w2230, "Boolean"=w2210, "Table in"=w2242) -> ("error out"=w2229:errorcluster)  [unwired: 6 in]
            n1158 = property class="Tbl (strict)"(reference=w2234, error in=w2229) -> (error out=w2232:errorcluster, "Value"=w2235:string[][])  [unwired: 1 out]
            n1159 = case shown="0, Default" w2226 {
              tunnel: w2210 -> [w2268 w2273]
              tunnel: [w2267 w2272] -> w2227
              tunnel: [w2266 FALSE] -> w2212
              tunnel: w2211 -> [w2265 _]
              tunnel: w2210 -> [w2264 _]
              frame 0, Default {
                n1160 = Not(x=w2264) -> (.not. x?=w2263:bool)
                n1161 = And(x=w2265, y=w2263) -> (x .and. y?=w2266:bool)
                n1162 = Select(t="ON", s=w2268, f="OFF") -> (s? t:f=w2267:string)
              }
              frame 1 {
                n1163 = Select(t="OFF", s=w2273, f="ON") -> (s? t:f=w2272:string)
              }
            }
            n1164 = Compound Arithmetic op=OR(w2208, w2212, w2214) -> (w2213:bool)
            n1165 = Replace Array Subset(array=w2235, new element=w2227, index (row)=w2250, index (col)=5 ("disabled index (col)")) -> (w2251:string[][])
            n1166 = property class="Tbl (strict)"(reference=w2233, error in=w2232, "Value"=w2251) -> (error out=w2243:errorcluster)  [unwired: 1 out]
          }
          n1167 = property class="VISAName"(reference=w2194, error in=w2184) -> (error out=w2171:errorcluster, "Value"=w2197:refnum<visa-resource-name>)  [unwired: 1 out]
          n1168 = property on="Start" class="Bool (strict)"(error in=w2171, "DisabledEnum"=w2172) -> (error out=w2173:errorcluster)  [unwired: 1 in, 1 out]
          n1169 = property on="Report" class="Bool (strict)"(error in=w2173, "DisabledEnum"=w2172) -> ()  [unwired: 1 in, 2 out]
          n1170 = VISA Write(VISA resource name=w2197, write buffer=w2196, error in (no error)=w2171) -> ()  [unwired: 3 out]
          n1171 = Build Array (concatenate)(w2181, w2180) -> (w2179:bool[])
          n1172 = And Array Elements(Boolean array=w2179) -> (logical AND=→"Auxiind":bool)
        }
      }
      n1173 = property on="Stop Button" class="Bool (strict)"() -> ("Value"=w259:bool)  [unwired: 2 in, 2 out]
      n1174 = Or(x=FALSE, y=w259) -> (x .or. y?=w260:bool)
      "f" <- w263
    }
    n1175 = property on="Pannel User Message" class="Str"(error in=w251, "Value"="You can press \"Start\" button to perform test(s).") -> ()  [unwired: 1 in, 2 out]
  }
  n1176 = while {
    shift-right: [w2511] -> _
    shift-left: T12."Initialize" -> [w2510]
    shift-right: [w2495] -> _
    shift-left: "" -> [w2498]
    shift-right: [w2506] -> _
    shift-left: _ -> [w2505]
    shift-right: [w2504] -> _
    shift-left: w23 -> [w2502]
    shift-right: [w2503] -> _
    shift-left: refnum<vi> refnum ("Config_CANAT") -> [w2501]
    shift-right: [w2499] -> _
    shift-left: w19 -> [w2500]
    tunnel: w12 -> [_]
    tunnel: w11 -> [w2497]
    tunnel: w10 -> [w2496]
    tunnel: w13 -> [w2508]
    tunnel: [w2507] -> _
    tunnel: w9 -> [_]
    tunnel: w8 -> [w2494]
    tunnel: w4 -> [w2493]
    shift-right: [w2491] -> _
    shift-left: 1 -> [w2492]
    tunnel: w2 -> [_]
    tunnel: w1 -> [_]
    stop <- w2509 stop-if-true
    n1177 = case shown="\"MainProgram\"" w2510 {
      tunnel: [T12."MainProgram" w2698 w2831 T12."Erase ATR Table"] -> w2511
      tunnel: [FALSE w2699 FALSE FALSE] -> w2509
      tunnel: [w2518 w2688 w2825 w3829] -> w2507
      tunnel: w2508 -> [_ w2685 w2829 _]
      tunnel: ["Initialization State..." w2696 w2813 "Initialization State..."] -> w2495
      tunnel: [w2564 w2693 w2826 w3840] -> w2506
      tunnel: w2505 -> [w2564 w2695 w2827 _]
      tunnel: [w2553 w2694 w2821 w3834] -> w2504
      tunnel: [w2552 w2692 w2822 w3836] -> w2503
      tunnel: w2502 -> [w2553 w2697 w2824 w3834]
      tunnel: w2501 -> [w2552 w2689 w2823 _]
      tunnel: w2500 -> [w2551 w2691 w2820 w3833]
      tunnel: [w2551 w2690 w2819 w3833] -> w2499
      tunnel: w2498 -> [_ w2686 w2815 _]
      tunnel: w2497 -> [_ _ w2818 _]
      tunnel: w2496 -> [w2525 _ w2812 _]
      tunnel: w2494 -> [_ _ w2811 _]
      tunnel: w2493 -> [_ _ w2810 _]
      tunnel: w2492 -> [w2517 w2682 w2809 w3828]
      tunnel: [w2517 w2682 w2808 w3828] -> w2491
      frame "Erase ATR Table", Default {
        w2522 = T13."Enabled" ("Disabled")
        w2533 = "Marvin" ("section")
        w2547 = refnum<visa-resource-name> "COM1" ("VISA resource name")
        w2559 = FALSE ("Visible")
        # "2"
        # "Venbale"
        # "Power ON"
        n1178 = call <vilib>:"Open Config Data.vi"("create file if necessary (T)"=FALSE, "configuration file path"=w2525) -> ("refnum"=w2523:T15)  [unwired: 7 in, 2 out]
        n1179 = property on="Serial Com" class="Bool"(error in=errorcluster {"status"=FALSE, "code"=0, "source"=""} ("error out"), "Visible"=TRUE) -> (error out=w2548:errorcluster)  [unwired: 1 in, 1 out]
        n1180 = case shown="False" w2535 {
          tunnel: ["AHU Software Version" ("key") "EBAY Software Version" ("key")] -> w2532
          tunnel: ["AHU Serial Number" ("key") "EBAY Serial Number" ("key")] -> w2531
          frame False {
          }
          frame True {
          }
        }
        n1181 = property on="VISA resource name" class="VISAName"(error in=w2548, "Visible"=w2559, "Value"=w2547) -> (error out=w2561:errorcluster)  [unwired: 1 in, 1 out]
        n1182 = property on="VISA resource name" class="VISAName"(error in=w2548, "Value"=w2547) -> ()  [unwired: 1 in, 2 out]
        n1183 = property on="Serial" class="Bool (strict)"(error in=w2561, "Value"=w2559) -> (error out=w2555:errorcluster)  [unwired: 1 in, 1 out]
        n1184 = flat-sequence {
          tunnel: [w2658] -> w2535
          tunnel: w2555 -> [w2657]
          tunnel: [w2656] -> w2529
          frame #0 {
            n1185 = disable-structure shown="Disabled" {
              frame Disabled {
                n1186 = Two Button Dialog(message="Please select the Unit Under Test.", 1:"AHU" ("F button name (\"Cancel\")"), 2:"EBAY" ("T button name (\"OK\")")) -> ()  [unwired: 1 out]
              }
              frame Enabled {
              }
            }
            n1187 = call "Select UUT"("error in (no error)"=w2657) -> ("EBAY"=w2658:bool, "error out"=w2656:errorcluster)  [unwired: 17 in]
          }
        }
        n1188 = call-poly <vilib>:"Read Key.vi"("section"=w2533, "error in (no error)"=w2529, "key"=w2532, "refnum"=w2523) -> ("error out"=w2530:errorcluster, "value"=→"SoftwareVer":string, "refnum out"=w2534:T15)  [unwired: 2 in, 3 out]
        n1189 = call-poly <vilib>:"Read Key.vi"("section"=w2533, "error in (no error)"=w2530, "key"=w2531, "refnum"=w2534) -> ("value"=w2528:string)  [unwired: 2 in, 5 out]
        n1190 = Decimal String To Number(string=w2528) -> (number=w2527:i32)  [unwired: 2 in, 1 out]
        n1191 = Increment(x=w2527) -> (x+1=w2516:i32)
        n1192 = Number To Decimal String(number=w2516) -> (decimal integer string=→"Next SN":string)  [unwired: 1 in]
        n1193 = case shown="False" w2535 {
          tunnel: [string[][] [["6.1", "Visual Inspection", "", "", "", "", ""], ["6.1.1", "Verification of Components Not Installed", "N/A", "-", "", "", ""], ["", "", "", "", "", "", ""], ["6.1.2", "Manufacturing Defects", "N/A", "-", "", "", ""], ["", "", "", "", "", "", ""], ["6.2", "Power Supply Testing", "", "", "", "", ""], ["6.2.1", "Input Current Drawn", "", "", "", "", ""], ["6.2.1.1", "DC Input Current", "< 150", "-", "mA", "", ""], ["", "", "", "", "", "", ""], ["6.2.2", "Power Supply Voltages", "", "", "", "", ""], ["6.2.2.1", "12V", "12.0", "+/-0.500", "V", "", ""], ["6.2.2.2", "5V", "5.0", "+/-0.200", "V", "", ""], ["6.2.2.3", "3.3V", "3.3", "+/-0.100", "V", "", ""], ["6.2.2.4", "1.8V", "1.8", "+/-0.100", "V", "", ""], ["", "", "", "", "", "", ""], ["7", "Functional Test Procedure", "", "", "", "", ""], ["7.1", "Weight Check", "3800", "+/-100.0", "gr", "", ""], ["", "", "", "", "", "", ""], ["7.2", "Insulation Resistance Test", "", "", "", "", ""], ["7.2.1", "J3.B to Chassis", "> 1M", "-", "W", "", ""], ["7.2.2", "J1.16 to Chassis", "> 100K", "-", "W", "", ""], ["", "", "", "", "", "", ""], ["7.2", "Bonding Resistance", "", "", "", "", ""], ["7.2.3", "J1 Body to Chassis", "< 2m", "-", "W", "", ""], ["7.2.4", "J2  Body to Chassis", "< 2m", "-", "W", "", ""], ["7.2.5", "J3  Body to Chassis", "< 2m", "-", "W", "", ""], ["", "", "", "", "", "", ""], ["7.2.1", "CANbus Resistance Test", "", "", "", "", ""], ["7.2.1.1", "J1.17 to J1.18", "> 10K", "-", "W", "", ""], ["", "", "", "", "", "", ""], ["7.3", "Sealing Test", "N/A", "-", "", "", ""], ["", "", "", "", "", "", ""], ["7.4", "Communication Test", "", "", "", "", ""], ["7.4.1", "Serial RS-232", "N/A", "-", "", "gf", "hfg"], ["7.4.2", "CAN Bus", "N/A", "-", "", "hfg", "hfg"], ["", "", "", "", "", "", ""], ["7.5", "Performances Tests", "", "", "", "", ""], ["7.5.1", "Reverse Polarity Test", "", "", "", "", ""], ["7.5.1.1", "DC Input Current", "< 1", "-", "mA", "", ""], ["", "", "", "", "", "", ""], ["7.5.2", "Enable Test", "", "", "", "", ""], ["7.5.2.1", "Fan Speed at Opened Enable ", "5000", "+/-200.0", "rpm", "", ""], ["7.5.2.2", "Fan Speed at Opened Enable ", "0", "+/-200.0", "rpm", "", ""], ["7.5.2.3", "Fan Speed at Closed Enable ", "5000", "+/-200.0", "rpm", "", ""], ["7.5.2.4", "Motor Rotation Direction", "Counter-clockwise (Inlet)", "-", "", "", ""], ["", "", "", "", "", "", ""], ["7.5.3", "Stop Time Test ", "", "", "", "", ""], ["7.5.3.1", "Motor Stop time", "< 50", "-", "sec", "", ""], ["", "", "", "", "", "", ""], ["7.5.4", "Speed Command Test", "", "", "", "", ""], ["7.5.4.1", "Fan Speed", "6000", "+/-200.0", "rpm", "", ""], ["7.5.4.2", "Fan Speed", "9000", "+/-200.0", "rpm", "", ""], ["7.5.4.3", "Fan Speed", "12100", "+/-200.0", "rpm", "", ""], ["", "", "", "", "", "", ""], ["7.5.5", "Temperature Sensor Calibration Test", "", "", "", "", ""], ["7.5.5.1", "Sensor Reading Analog Offset", "0", "+/-0.100", ".", "", ""], ["", "", "", "", "", "", ""], ["7.5.6", "Burn-in Test", "", "", "", "", ""], ["7.5.6.1", "DC Input Current", "28", "+/-5.000", "A", "", ""], ["7.5.6.2", "Ambient Temperature", "25", "+/-13.00", "ºC", "", ""], ["7.5.6.3", "After 10 min of operation", "", "", "ºC", "", ""], ["7.5.6.4", "After 20 min of operation", "", "", "ºC", "", ""], ["7.5.6.5", "After 30 min of operation", "", "", "ºC", "", ""], ["", "", "", "", "", "", ""], ["9", "Motor Temp. Test", "", "", "", "", ""], ["9.1", "60 Degree", "60", "+/-3.00", "ºC", "", ""], ["9.2", "90 Degree", "90", "+/-3.00", "ºC", "", ""], ["9.3", "110 Degree", "110", "+/-3.00", "ºC", "", ""]] ("data") string[][] [["6.1", "Visual Inspection", "", "", "", "", ""], ["6.1.1", "Verification of Components Not Installed", "N/A", "-", "", "", ""], ["", "", "", "", "", "", ""], ["6.1.2", "Manufacturing Defects", "N/A", "-", "", "", ""], ["", "", "", "", "", "", ""], ["6.2", "Power Supply Testing", "", "", "", "", ""], ["6.2.1", "Input Current Drawn", "", "", "", "", ""], ["6.2.1.1", "DC Input Current", "< 150", "-", "mA", "", ""], ["", "", "", "", "", "", ""], ["6.2.2", "Power Supply Voltages", "", "", "", "", ""], ["6.2.2.1", "12V", "12.0", "+/-0.500", "V", "", ""], ["6.2.2.2", "5V", "5.0", "+/-0.200", "V", "", ""], ["6.2.2.3", "3.3V", "3.3", "+/-0.100", "V", "", ""], ["6.2.2.4", "1.8V", "1.8", "+/-0.100", "V", "", ""], ["", "", "", "", "", "", ""], ["7", "Functional Test Procedure", "", "", "", "", ""], ["7.1", "Weight Check", "4180", "+/-10.00", "gr", "", ""], ["", "", "", "", "", "", ""], ["7.2", "Insulation Resistance Test", "", "", "", "", ""], ["7.2.1", "J3.B to Chassis", "> 1M", "-", "W", "", ""], ["7.2.2", "J1.16 to Chassis", "> 100K", "-", "W", "", ""], ["", "", "", "", "", "", ""], ["7.2", "Bonding Resistance", "", "", "", "", ""], ["7.2.3", "J1 Body to Chassis", "< 2m", "-", "W", "", ""], ["7.2.4", "J2  Body to Chassis", "< 2m", "-", "W", "", ""], ["7.2.5", "J3  Body to Chassis", "< 2m", "-", "W", "", ""], ["", "", "", "", "", "", ""], ["7.2.1", "CANbus Resistance Test", "", "", "", "", ""], ["7.2.1.1", "J1.17 to J1.18", "> 10K", "-", "W", "", ""], ["", "", "", "", "", "", ""], ["7.3", "Sealing Test", "N/A", "-", "", "", ""], ["", "", "", "", "", "", ""], ["7.4", "Communication Test", "", "", "", "", ""], ["7.4.1", "Serial RS-232", "N/A", "-", "", "", ""], ["7.4.2", "CAN Bus", "N/A", "-", "", "", ""], ["", "", "", "", "", "", ""], ["7.5", "Performances Tests", "", "", "", "", ""], ["7.5.1", "Reverse Polarity Test", "", "", "", "", ""], ["7.5.1.1", "DC Input Current", "< 1", "-", "mA", "", ""], ["", "", "", "", "", "", ""], ["7.5.2", "Enable Test", "", "", "", "", ""], ["7.5.2.1", "Fan Speed before Opened Enable ", "5000", "+/-200.0", "rpm", "", ""], ["7.5.2.2", "Fan Speed at Opened Enable ", "0", "+/-200.0", "rpm", "", ""], ["7.5.2.3", "Fan Speed at Closed Enable ", "5000", "+/-200.0", "rpm", "", ""], ["7.5.2.4", "Motor Rotation Direction", "Counter-clockwise (Inlet)", "-", "", "", ""], ["", "", "", "", "", "", ""], ["7.5.3", "Stop Time Test ", "", "", "", "", ""], ["7.5.3.1", "Motor Stop time", "< 50", "-", "sec", "", ""], ["", "", "", "", "", "", ""], ["7.5.4", "Speed Command Test", "", "", "", "", ""], ["7.5.4.1", "Fan Speed", "6000", "+/-200.0", "rpm", "", ""], ["7.5.4.2", "Fan Speed", "11500", "+/-200.0", "rpm", "", ""], ["7.5.4.3", "Fan Speed", "15100", "+/-200.0", "rpm", "", ""], ["", "", "", "", "", "", ""], ["7.5.5", "Temperature Sensor Calibration Test", "", "", "", "", ""], ["7.5.5.1", "Sensor Reading Analog Offset", "0", "+/-0.100", ".", "", ""], ["", "", "", "", "", "", ""], ["7.5.6", "Temperature Control Algorithm Test", "", "", "", "", ""], ["7.5.6.1", "Tair <   68 ± 2 oC", "6000", "+/-200.0", "rpm", "", ""], ["7.5.6.2", "Measured Temp.", "", "", "ºC", "", ""], ["7.5.6.3", "Tair >= 68 ± 2 oC", "11500", "+/-200.0", "rpm", "", ""], ["7.5.6.4", "Transition Temp.", "", "", "ºC.", "", ""], ["7.5.6.5", "Tair >= 88 ± 2 oC", "15100", "+/-400.0", "rpm", "", ""], ["7.5.6.6", "Transition Temp.", "", "", "ºC", "", ""], ["7.5.6.7", "Tair <= 80 ± 2 oC", "11500", "+/-200.0", "rpm", "", ""], ["7.5.6.8", "Transition Temp.", "", "", "ºC", "", ""], ["7.5.6.9", "Tair <= 60 ± 2 oC", "6000", "+/-200.0", "rpm", "", ""], ["7.5.6.10", "Transition Temp.", "", "", "ºC", "", ""], ["", "", "", "", "", "", ""], ["7.5.7", "Burn-in Test", "", "", "", "", ""], ["7.5.7.1", "DC Input Current", "50", "+/-7.000", "A", "", ""], ["7.5.7.2", "Fan Speed", "15100", "+/-400.0", "rpm", "", ""], ["7.5.7.3", "Ambient Temperature", "25", "+/-13.00", "ºC", "", ""], ["7.5.7.4", "After 10 min of operation", "", "-", "ºC", "", ""], ["7.5.7.5", "After 20 min of operation", "", "-", "ºC", "", ""], ["7.5.7.6", "After 30 min of operation", "", "-", "ºC", "", ""], ["", "", "", "", "", "", ""], ["8", "Auxiliary Fan Test", "", "", "", "", ""], ["8.1", "Auxiliary Cooling Fan ON", "60", "+/-2.00", "ºC", "", ""], ["8.2", "Fan status", "ON", "-", "-", "", ""], ["8.3", "Auxiliary Cooling Fan OFF", "55", "+/-2.00", "ºC", "", ""], ["8.4", "Fan status", "OFF", "-", "-", "", ""], ["", "", "", "", "", "", ""], ["9", "Motor Temp. Test", "", "", "", "", ""], ["9.1", "60 Degree", "60", "+/-3.00", "ºC", "", ""], ["9.2", "90 Degree", "90", "+/-3.00", "ºC", "", ""], ["9.3", "110 Degree", "110", "+/-3.00", "ºC", "", ""]] ("data")] -> w2557
          tunnel: ["AHU" "EBAY"] -> w2556
          tunnel: [w2662 w2665] -> w2554
          tunnel: w2529 -> [w2662 w2665]
          frame False {
          }
          frame True {
          }
        }
        "UUT" <- w2556
        n1194 = for {
          tunnel: w2557 -> [w2672] mode=indexing
          tunnel: w2554 -> [w2670]
          tunnel: [w2669] -> w2550
          tunnel: w2557 -> [w2668]
          i -> [w2671]
          n1195 = for {
            tunnel: w2672 -> [_] mode=indexing
            tunnel: w2671 -> [w2678]
            tunnel: w2670 -> [w2675]
            tunnel: [w2674] -> w2669
            tunnel: w2668 -> [w2673]
            i -> [w2679]
            n1196 = Bundle By Name(cluster=T17 {"Row"=0, "Column"=0} ("Active Cell:Active Cell"), "Row"=w2678, "Column"=w2679) -> (w2677:T17)
            n1197 = control-ref of="ATR"() -> (w2676:refnum<vi>)
            n1198 = property class="Tbl (strict)"(reference=w2676, error in=w2675, "Active Cell"=w2677, "Cell BG Color"=u32 16777226, "Value"=w2673) -> (error out=w2674:errorcluster)  [unwired: 1 out]
          }
        }
        n1199 = property on="Automation" class="Bool (strict)"("Value"=FALSE ("Automation")) -> ()  [unwired: 2 in, 2 out]
        n1200 = call "COM EvolutionBoard.vi"("error in (no error)"=w2550, "VISA resource name 2"=refnum<visa-resource-name> "COM1" ("VISA resource name")) -> ("error out"=w2539:errorcluster, ".not. x?"=w2540:bool, "VISA resource name out"=w2537:refnum<visa-resource-name>)  [unwired: 7 in]
        "VISA resource name out" <- w2537
        n1201 = Byte Array To String(unsigned byte array=u8[] [75, 0, 4, 2, 0, 0, 0, 0] ("appended array")) -> (string=w2542:string)
        n1202 = Byte Array To String(unsigned byte array=u8[] [75, 0, 4, 2, 0, 0, 0, 0] ("appended array")) -> (string=w2546:string)
        n1203 = case shown="True" w2540 {
          tunnel: w2539 -> [w2571 w2577]
          tunnel: [w2570 w2574] -> w2538
          tunnel: w2537 -> [w2569 w2578]
          tunnel: [w2569 w2573] -> w2536
          frame False {
            n1204 = call "Display Message to User4"("error in (no error)"=w2571) -> ("error out"=w2570:errorcluster)  [unwired: 9 in, 1 out]
          }
          frame True {
            n1205 = Byte Array To String(unsigned byte array=u8[] [75, 0, 4, 17, 0, 0, 0, 0] ("appended array")) -> (string=w2581:string)
            n1206 = VISA Write(VISA resource name=w2578, write buffer=w2581, error in (no error)=w2577) -> (VISA resource name out=w2576:refnum<visa-resource-name>, error out=w2582:errorcluster)  [unwired: 1 out]
            n1207 = while {
              tunnel: w2576 -> [w2596]
              tunnel: w2580 -> [w2595]
              tunnel: [w2594] -> w2573
              tunnel: [w2593] -> w2574
              tunnel: w2575 -> [w2591]
              tunnel: [w2585] -> w2572
              stop <- w2587 stop-if-true
              n1208 = VISA Read(VISA resource name=w2596, byte count=u32 1, error in (no error)=w2595) -> (VISA resource name out=w2598:refnum<visa-resource-name>, read buffer=w2599:string, error out=w2597:errorcluster)  [unwired: 1 out]
              n1209 = String To Byte Array(string=w2599) -> (unsigned byte array=w2602:u8[])
              n1210 = Index Array(array=w2602, index=0) -> (element=w2600:u8)
              n1211 = case shown="75" w2600 {
                tunnel: [w2607 w2611] -> w2593
                tunnel: w2598 -> [w2606 w2620]
                tunnel: w2597 -> [w2607 w2619]
                tunnel: [w2606 w2612] -> w2594
                tunnel: [u32 9999 w2609] -> w2585
                tunnel: [FALSE w2608] -> w2586
                frame 0, Default {
                }
                frame 75 {
                  n1212 = VISA Read(VISA resource name=w2620, byte count=u32 3, error in (no error)=w2619) -> (VISA resource name out=w2615:refnum<visa-resource-name>, read buffer=w2623:string, error out=w2614:errorcluster)  [unwired: 1 out]
                  n1213 = String To Byte Array(string=w2623) -> (unsigned byte array=w2613:u8[])
                  n1214 = Index Array(array=w2613, index #1=0 ("index")) -> (element #1=w2618:u8, element #2=w2616:u8)  [unwired: 2 in, 1 out]
                  n1215 = Equal?(x=u8 0, y=w2618) -> (x = y?=w2617:bool)
                  n1216 = case shown="True" w2617 {
                    tunnel: [w2626 w2633] -> w2611
                    tunnel: w2616 -> [_ w2640]
                    tunnel: w2615 -> [w2627 w2639]
                    tunnel: w2614 -> [w2626 w2638]
                    tunnel: w2613 -> [_ w2637]
                    tunnel: [w2627 w2635] -> w2612
                    tunnel: [u32 9999 w2629] -> w2609
                    tunnel: [FALSE w2628] -> w2608
                    frame False {
                    }
                    frame True {
                      n1217 = VISA Read(VISA resource name=w2639, byte count=w2640, error in (no error)=w2638) -> (VISA resource name out=w2635:refnum<visa-resource-name>, read buffer=w2634:string, error out=w2633:errorcluster)  [unwired: 1 out]
                      n1218 = String To Byte Array(string=w2634) -> (unsigned byte array=w2636:u8[])
                      n1219 = Insert Into Array(array=w2637, new element=w2636) -> (w2630:u8[])  [unwired: 1 in]
                      n1220 = Index Array(array=w2630, index #1=0 ("index")) -> (element #3=w2631:u8)  [unwired: 2 in, 2 out]
                      n1221 = case shown="15..19" w2631 {
                        tunnel: w2630 -> [_ w2654]
                        tunnel: [u32 9999 w2643] -> w2629
                        tunnel: [FALSE w2644] -> w2628
                        frame 0, Default {
                        }
                        frame 15..19 {
                          n1222 = Index Array(array=w2654, index #1=3 ("index")) -> (element #1=w2653:u8, element #2=w2652:u8, element #3=w2651:u8, element #4=w2650:u8)  [unwired: 3 in]
                          n1223 = Join Numbers(hi=w2652, lo=w2653) -> ((hi.lo)=w2649:u16)
                          n1224 = Join Numbers(hi=w2650, lo=w2651) -> ((hi.lo)=w2648:u16)
                          n1225 = Join Numbers(hi=w2648, lo=w2649) -> ((hi.lo)=w2646:u32)
                          n1226 = Multiply(x=0.02003173828125, y=w2646) -> (x*y=w2643:dbl)
                          n1227 = Greater Or Equal?(x=w2643, y=0.0) -> (x >= y?=w2644:bool)
                        }
                      }
                    }
                  }
                }
              }
              n1228 = call <vilib>:"High Resolution Relative Seconds.vi"() -> ("relative seconds"=w2592:dbl)
              n1229 = Subtract(x=w2592, y=w2591) -> (x-y=w2590:dbl)
              n1230 = Greater Or Equal?(x=w2590, y=10.0) -> (x >= y?=w2588:bool)
              n1231 = Compound Arithmetic op=OR(w2588, w2586) -> (w2587:bool)
            }
            "CurrentOffset" <- w2572
            n1232 = flat-sequence {
              tunnel: w2582 -> [w2584]
              tunnel: [w2584] -> w2580
              tunnel: [w2583] -> w2575
              frame #0 {
                n1233 = call <vilib>:"High Resolution Relative Seconds.vi"() -> ("relative seconds"=w2583:dbl)
              }
            }
          }
        }
        n1234 = VISA Write(VISA resource name=w2536, write buffer=w2546, error in (no error)=w2538) -> (error out=w2544:errorcluster)  [unwired: 2 out]
        n1235 = call "Time Delay5"("error in (no error)"=w2544) -> ("error out"=w2543:errorcluster)  [unwired: 10 in]
        n1236 = VISA Write(VISA resource name=w2536, write buffer=w2542, error in (no error)=w2543) -> (error out=w2519:errorcluster)  [unwired: 2 out]
        n1237 = call <vilib>:"Clear Errors.vi"("error in (no error)"=w2519) -> ("error out"=w2518:errorcluster)  [unwired: 5 in, 1 out]
        n1238 = property on="Start" class="Bool (strict)"(error in=w2518, "DisabledEnum"=w2522) -> (error out=w2521:errorcluster)  [unwired: 1 in, 1 out]
        n1239 = property on="Report" class="Bool (strict)"(error in=w2521, "DisabledEnum"=w2522) -> (error out=w2514:errorcluster)  [unwired: 1 in, 1 out]
        n1240 = property on="ClosePanel" class="Bool (strict)"(error in=w2514, "Value"=FALSE ("ClosePanel")) -> ()  [unwired: 1 in, 2 out]
      }
      frame "Stop" {
        n1241 = disable-structure shown="Disabled" {
          disable-tunnel: w2691 -> [w2703 w2704]
          disable-tunnel: [w2702 w2704] -> w2683
          frame Disabled {
            n1242 = Preview Queue Element(queue=w2703) -> (queue out=w2702:refnum<queue>, element=w2701:T10)  [unwired: 2 in, 2 out]
            n1243 = Unbundle By Name(w2701) -> ("Array Test"=→"Array Test":T1)
          }
          frame Enabled {
          }
        }
        n1244 = property on="Stop Button" class="Bool (strict)"(error in=w2685) -> (error out=w2684:errorcluster, "Value"=w2687:bool)  [unwired: 1 in, 1 out]
        n1245 = case shown="True" w2687 {
          tunnel: [FALSE w2745] -> w2699
          tunnel: [T12."Initialize" w2744] -> w2698
          tunnel: w2697 -> [w2717 w2743]
          tunnel: ["Restarting program..." w2742] -> w2696
          tunnel: w2695 -> [w2726 w2741]
          tunnel: [w2716 w2740] -> w2694
          tunnel: [refnum<visa-resource-name> refnum ("VISA resource name") w2739] -> w2693
          tunnel: [w2706 w2738] -> w2692
          tunnel: w2683 -> [w2715 w2737]
          tunnel: [w2714 w2736] -> w2690
          tunnel: w2684 -> [w2705 w2733]
          tunnel: w2689 -> [w2706 w2735]
          tunnel: [w2718 w2734] -> w2688
          tunnel: w2686 -> [_ _]
          frame False {
            # "K15 OFF + Venable"
            n1246 = Flush Queue(queue=w2717) -> (queue out=w2716:refnum<queue>)  [unwired: 1 in, 2 out]
            n1247 = Flush Queue(queue=w2715) -> (queue out=w2714:refnum<queue>)  [unwired: 1 in, 2 out]
            n1248 = control-ref of="VISA resource name out"() -> (w2724:refnum<vi>)
            n1249 = call "Reset CAN Device.vi"("error in (no error)"=w2705, "Cluster in"=w2706) -> ()  [unwired: 9 in, 1 out]
            n1250 = Merge Errors(w2705) -> (w2718:errorcluster)
            n1251 = VISA Flush I/O Buffer(VISA resource name=w2726, error in (no error)=w2705) -> (VISA resource name out=w2713:refnum<visa-resource-name>, error out=w2707:errorcluster)  [unwired: 1 in]
            n1252 = VISA Close(VISA resource name=w2713, error in (no error)=w2705) -> (error out=w2708:errorcluster)
            n1253 = call <vilib>:"Clear Errors.vi"("error in (no error)"=w2708) -> ()  [unwired: 5 in, 2 out]
            n1254 = call <vilib>:"Clear Errors.vi"("error in (no error)"=w2707) -> ()  [unwired: 5 in, 2 out]
            n1255 = property class="VISAName"(reference=w2724, error in=w2705) -> (error out=w2721:errorcluster, "Value"=w2720:refnum<visa-resource-name>)  [unwired: 1 out]
            n1256 = Byte Array To String(unsigned byte array=u8[] [75, 0, 4, 2, 0, 0, 16, 0] ("appended array")) -> (string=w2723:string)
            n1257 = VISA Write(VISA resource name=w2720, write buffer=w2723, error in (no error)=w2721) -> (VISA resource name out=w2719:refnum<visa-resource-name>, error out=w2711:errorcluster)  [unwired: 1 out]
            n1258 = VISA Flush I/O Buffer(VISA resource name=w2719, error in (no error)=w2711) -> (VISA resource name out=w2712:refnum<visa-resource-name>, error out=w2710:errorcluster)  [unwired: 1 in]
            n1259 = VISA Close(VISA resource name=w2712, error in (no error)=w2710) -> (error out=w2709:errorcluster)
            n1260 = call <vilib>:"Clear Errors.vi"("error in (no error)"=w2709) -> ()  [unwired: 5 in, 2 out]
          }
          frame True {
            n1261 = property on="ClosePanel" class="Bool (strict)"() -> ("Value"=w2730:bool)  [unwired: 2 in, 2 out]
            n1262 = case shown="False" w2730 {
              tunnel: w2733 -> [w2748 w2750]
              tunnel: [w2747 w2750] -> w2732
              tunnel: [w2746 TRUE ("Yes")] -> w2731
              frame False {
                n1263 = call "Display Message to User7"("error in (no error)"=w2748) -> ("error out"=w2747:errorcluster, "Yes"=w2746:bool)  [unwired: 9 in]
              }
              frame True {
              }
            }
            n1264 = case shown="True" w2731 {
              tunnel: [FALSE TRUE] -> w2745
              tunnel: [T12."MainProgram" T12."Stop"] -> w2744
              tunnel: w2743 -> [w2754 w2799]
              tunnel: [w2753 w2775] -> w2734
              tunnel: ["Press \"Start\" to perform test(s)." "Program Stopped...\r\nPlease turn OFF All Power sinks"] -> w2742
              tunnel: w2741 -> [w2764 w2797]
              tunnel: [w2762 refnum<queue> refnum ("queue out")] -> w2740
              tunnel: [w2764 refnum<visa-resource-name> refnum ("VISA resource name")] -> w2739
              tunnel: [w2752 refnum<vi> refnum ("Config_CANAT")] -> w2738
              tunnel: w2737 -> [w2760 w2792]
              tunnel: [w2761 refnum<queue> refnum ("queue out")] -> w2736
              tunnel: w2732 -> [w2753 w2777]
              tunnel: w2735 -> [w2752 w2778]
              tunnel: w2730 -> [_ w2774]
              frame False {
                n1265 = call "Clear CAN Buffer.vi"("error in (no error)"=w2753, "Cluster in"=w2752) -> ()  [unwired: 8 in, 2 out]
                n1266 = Flush Queue(queue=w2754) -> (queue out=w2762:refnum<queue>)  [unwired: 1 in, 2 out]
                n1267 = property on="f" class="Enum (strict)"(error in=w2753) -> (error out=w2756:errorcluster, "Value"=w2759:T2)  [unwired: 1 in, 1 out]
                n1268 = Equal?(x=w2759, y=T2."Empty") -> (x = y?=w2757:bool)
                n1269 = case shown="False" w2757 {
                  tunnel: [w2767 w2768] -> w2751
                  tunnel: w2756 -> [w2767 w2768]
                  frame False {
                  }
                  frame True {
                  }
                }
                n1270 = property on="Stop Button" class="Bool (strict)"(error in=w2751, "Value"=FALSE ("Stop Button")) -> ()  [unwired: 1 in, 2 out]
                n1271 = Flush Queue(queue=w2760, error in (no error)=w2751) -> (queue out=w2761:refnum<queue>)  [unwired: 2 out]
              }
              frame True {
                # "K15 OFF + Venable"
                n1272 = call "Close CAN Device.vi"("error in (no error)"=w2777, "Cluster in"=w2778) -> ()  [unwired: 8 in, 2 out]
                n1273 = control-ref of="VISA resource name out"() -> (w2791:refnum<vi>)
                n1274 = Flush Queue(queue=w2799, error in (no error)=w2777) -> (queue out=w2770:refnum<queue>, error out=w2800:errorcluster)  [unwired: 1 out]
                n1275 = Release Queue(queue=w2770, force destroy? (F)=TRUE, error in (no error)=w2800) -> (error out=w2771:errorcluster)  [unwired: 2 out]
                n1276 = VISA Close(VISA resource name=w2797, error in (no error)=w2777) -> (error out=w2781:errorcluster)
                n1277 = Flush Queue(queue=w2792, error in (no error)=w2777) -> (queue out=w2769:refnum<queue>, error out=w2793:errorcluster)  [unwired: 1 out]
                n1278 = call <vilib>:"Clear Errors.vi"("error in (no error)"=w2793) -> ("error out"=w2783:errorcluster)  [unwired: 5 in, 1 out]
                n1279 = Release Queue(queue=w2769, force destroy? (F)=TRUE, error in (no error)=w2783) -> (error out=w2780:errorcluster)  [unwired: 2 out]
                n1280 = property class="VISAName"(reference=w2791, error in=w2777) -> (error out=w2787:errorcluster, "Value"=w2786:refnum<visa-resource-name>)  [unwired: 1 out]
                n1281 = Byte Array To String(unsigned byte array=u8[] [75, 0, 4, 2, 0, 0, 16, 0] ("appended array")) -> (string=w2789:string)
                n1282 = VISA Write(VISA resource name=w2786, write buffer=w2789, error in (no error)=w2787) -> (VISA resource name out=w2785:refnum<visa-resource-name>, error out=w2784:errorcluster)  [unwired: 1 out]
                n1283 = VISA Close(VISA resource name=w2785, error in (no error)=w2784) -> (error out=w2782:errorcluster)
                n1284 = Merge Errors(w2771, w2782, w2781, w2780) -> (w2779:errorcluster)
                n1285 = call <vilib>:"Clear Errors.vi"("error in (no error)"=w2779) -> ("error out"=w2776:errorcluster)  [unwired: 5 in, 1 out]
                n1286 = case shown="True" w2774 {
                  tunnel: w2776 -> [w2803 w2806]
                  tunnel: [w2803 w2804] -> w2775
                  frame False {
                  }
                  frame True {
                    n1287 = control-ref of="This VI"() -> (w2807:refnum<vi>)
                    n1288 = property class="VI"(reference=w2807, error in=w2806, "FP.State"=T18."Closed" ("Front Panel Window:State")) -> (error out=w2804:errorcluster)  [unwired: 1 out]
                  }
                }
              }
            }
          }
        }
      }
      frame "MainProgram" {
        n1289 = event shown="[10] \"Refresh Button\": Value Change" {
          selector: w2810 -> [_ _ _ _ _ _ _ _ _ _ _ _ _]
          dyn-events: _ -> [_ _ _ _ _ _ _ _ _ _ _ _ _]
          timeout: 50 -> [_ _ _ _ _ _ _ _ _ _ _ _ _]
          tunnel: [T12."MainProgram" T12."MainProgram" T12."MainProgram" T12."MainProgram" T12."MainProgram" T12."MainProgram" w3436 T12."MainProgram" T12."MainProgram" T12."MainProgram" T12."Stop" T12."MainProgram" T12."MainProgram"] -> w2831
          tunnel: [w2836 w2910 w3001 w3008 w3017 w3029 w3470 w3564 w3583 w3588 w3712 w3715 w3727] -> w2825
          tunnel: w2829 -> [w2841 w2935 w3000 w3010 w3017 w3047 w3472 w3571 w3582 w3592 w3712 w3715 w3730]
          tunnel: [w2850 w2914 w3002 w3009 w3018 w3041 w3468 w3569 w3580 w3596 w3709 w3721 w3729] -> w2826
          tunnel: w2827 -> [w2850 w2914 w3002 w3009 w3018 w3041 w3468 w3569 w3580 _ w3709 w3721 w3729]
          tunnel: w2824 -> [w2843 w2939 w2996 w3005 w3014 w3044 w3475 w3568 w3579 w3599 w3708 w3720 w3734]
          tunnel: w2823 -> [w2837 w2940 w2997 w3006 w3015 w3045 w3474 w3567 w3578 w3598 w3707 w3719 w3733]
          tunnel: [w2839 w2940 w2997 w3006 w3015 w3045 w3474 w3567 w3578 w3598 w3707 w3719 w3733] -> w2822
          tunnel: [w2842 w2939 w2996 w3005 w3014 w3044 w3475 w3568 w3579 w3599 w3708 w3720 w3734] -> w2821
          tunnel: w2820 -> [w2840 w2941 w2995 w3004 w3013 w3043 w3473 w3566 w3577 w3597 w3706 w3718 w3732]
          tunnel: [w2840 w2941 w2995 w3004 w3013 w3039 w3473 w3566 w3577 w3597 w3706 w3718 w3732] -> w2819
          tunnel: w2818 -> [_ _ _ _ _ _ _ _ _ _ _ _ _]
          tunnel: [w2834 _ _ _ _ w3038 _ _ _ _ _ _ _] -> w2814
          tunnel: w2815 -> [_ _ _ _ _ w3038 _ _ _ _ _ _ _]
          tunnel: w2812 -> [_ _ _ _ _ _ w3455 _ _ _ _ _ _]
          tunnel: w2812 -> [_ w2909 _ _ _ _ _ _ _ _ _ _ _]
          tunnel: w2811 -> [_ _ _ _ _ _ w3466 _ _ _ _ _ _]
          tunnel: w2809 -> [w2833 w2906 w2994 w3003 w3012 w3031 w3429 w3563 w3576 w3590 w3705 w3713 w3723]
          tunnel: [w2833 w2906 w2994 w3003 w3012 w3031 w3428 w3563 w3576 w3590 w3705 w3713 w3723] -> w2808
          event Timeout {
            n1290 = event-data() -> ()  [unwired: 1 in, 3 out]
            n1291 = property class="Clust (strict)"(reference=w2837, error in=w2841) -> (reference out=w2839:refnum<vi>, error out=w2838:errorcluster, "Value"=w2847:T9)
            n1292 = Unbundle By Name(w2847) -> ("DevType"=w2848:T4, "CanIndex"=w2845:T3)
            n1293 = call "VCI_Receive.vi"("CANIndex"=w2845, "DevIndex"=u32 0, "DevType"=w2848) -> ("Recieve"=w2844:T21[])  [unwired: 3 in, 5 out]
            n1294 = Empty Array?(array=w2844) -> (empty?=w2846:bool)
            n1295 = case shown="False" w2846 {
              tunnel: w2845 -> [w2870 _]
              tunnel: w2839 -> [w2868 _]
              tunnel: w2843 -> [w2867 w2903]
              tunnel: w2838 -> [w2866 w2902]
              tunnel: w2844 -> [w2871 _]
              tunnel: [w2861 w2902] -> w2836
              tunnel: [w2860 w2903] -> w2842
              tunnel: [w2859 0] -> _
              frame False {
                n1296 = call "Demo_MakeDispBuff.vi"("Channel"=w2870, "Type"=enum16{"接收", "发送"}."接收", "OBJs"=w2871) -> ("Buffer"=w2869:T22)
                n1297 = for {
                  N: 3 -> [_]
                  tunnel: w2869 -> [w2885]
                  tunnel: w2868 -> [w2884]
                  tunnel: w2867 -> [w2875]
                  tunnel: w2866 -> [w2874]
                  tunnel: [w2877] -> w2864 mode=indexing
                  tunnel: [w2875] -> w2863
                  tunnel: [w2874] -> w2862
                  tunnel: [w2873] -> w2859
                  i -> [w2873]
                  n1298 = property class="Clust (strict)"(reference=w2884) -> ("Value"=w2882:T9)  [unwired: 1 in, 2 out]
                  n1299 = Index Array(array=w2885, index=w2873) -> (element=w2878:T23)
                  n1300 = Unbundle By Name(w2878) -> ("Channel"=w2880:T3, "VCI_CAN_OBJ"=w2883:T21)  [unwired: 2 out]
                  n1301 = Unbundle By Name(w2882) -> ("CanIndex"=w2881:T3)
                  n1302 = Equal?(x=w2881, y=w2880) -> (x = y?=w2879:bool)
                  n1303 = case shown="True" w2879 {
                    tunnel: w2883 -> [_ w2896]
                    tunnel: [w2886 w2892] -> w2877
                    tunnel: T14 {"ID"=0, "MSGTYPE"=0, "LEN"=0, "aDATA"=[]} ("Msg") -> [w2886 w2891]
                    frame False {
                    }
                    frame True {
                      n1304 = Unbundle By Name(w2896) -> ("ID"=w2890:u32, "DataLen"=w2895:u8, "Data"=w2893:u8[])
                      n1305 = Bundle By Name(cluster=w2891, "ID"=w2890, "MSGTYPE"=u8 0, "LEN"=w2895, "aDATA"=w2893) -> (w2892:T14)
                      n1306 = Unbundle By Name(w2892) -> ("ID"=w2888:u32)
                      n1307 = Split Number(x=w2888) -> (lo(x)=w2889:u16)  [unwired: 1 out]
                      n1308 = Split Number(x=w2889) -> (lo(x)=w2887:u8)  [unwired: 1 out]
                      "UUT" <- w2887
                      n1309 = case shown="63" w2887 {
                        tunnel: ["EBAY 5F" "" "AHU 3F" "AHU 2F"] -> _
                        frame 95 {
                        }
                        frame Default {
                        }
                        frame 63 {
                        }
                        frame 47 {
                        }
                      }
                    }
                  }
                }
                n1310 = Enqueue Element(queue=w2863, element=w2864, error in (no error)=w2862) -> (queue out=w2860:refnum<queue>, error out=w2861:errorcluster)  [unwired: 2 out]
              }
              frame True {
              }
            }
            n1311 = property on="ClosePanel" class="Bool (strict)"() -> ("Value"=→"ClosePanel 2":bool)  [unwired: 2 in, 2 out]
            n1312 = First Call?() -> (First Call?: T/F=w2835:bool)
            n1313 = case shown="False" w2835 {
              tunnel: [w2855 "Main Program..."] -> w2834
              frame False {
                n1314 = property on="f" class="Enum (strict)"() -> ("Value"=w2854:T2)  [unwired: 2 in, 2 out]
                n1315 = Equal?(x=w2854, y=T2."Empty") -> (x = y?=w2852:bool)
                n1316 = property on="Pannel User Message" class="Str"() -> ("Value"=w2856:string)  [unwired: 2 in, 2 out]
                n1317 = Select(t="You can press \"Start\" button to perform test(s).", s=w2852, f=w2856) -> (s? t:f=w2855:string)
              }
              frame True {
              }
            }
          }
          event "SetSN": Value Change {
            w2904 = TRUE ("Report")
            n1318 = event-data() -> ()  [unwired: 1 in, 6 out]
            n1319 = property on="UUT" class="DigNum (strict)"() -> ("Value"=w2944:u8)  [unwired: 2 in, 2 out]
            n1320 = Equal?(x=w2944, y=u8 95) -> (x = y?=w2942:bool)
            n1321 = property on="ComTestind" class="Bool (strict)"() -> ("Value"=w2921:bool)  [unwired: 2 in, 2 out]
            n1322 = property on="VisualInspectionResult" class="Bool (strict)"() -> ("Value"=w2924:bool)  [unwired: 2 in, 2 out]
            n1323 = property on="Auxiind" class="Bool (strict)"() -> ("Value"=w2923:bool)  [unwired: 2 in, 2 out]
            n1324 = property on="TempSensCalind" class="Bool (strict)"() -> ("Value"=w2926:bool)  [unwired: 2 in, 2 out]
            n1325 = call <vilib>:"Clear Errors.vi"("error in (no error)"=w2935) -> ("error out"=w2933:errorcluster)  [unwired: 5 in, 1 out]
            n1326 = case shown="True" w2942 {
              tunnel: ["AHU Software Version" ("key") "EBAY Software Version" ("key")] -> _
              tunnel: ["AHU Serial Number" ("key") "EBAY Serial Number" ("key")] -> w2915
              tunnel: [TRUE ("Value") w2991] -> w2918
              frame False {
              }
              frame True {
                n1327 = property on="TempControlind" class="Bool (strict)"() -> ("Value"=w2991:bool)  [unwired: 2 in, 2 out]
              }
            }
            n1328 = VISA Flush I/O Buffer(VISA resource name=w2914, error in (no error)=w2933) -> (VISA resource name out=w2937:refnum<visa-resource-name>, error out=w2934:errorcluster)  [unwired: 1 in]
            n1329 = property on="MotorTempind" class="Bool (strict)"() -> ("Value"=w2919:bool)  [unwired: 2 in, 2 out]
            n1330 = property on="SpeedStopind" class="Bool (strict)"() -> ("Value"=w2920:bool)  [unwired: 2 in, 2 out]
            n1331 = property on="Burninind" class="Bool (strict)"() -> ("Value"=w2925:bool)  [unwired: 2 in, 2 out]
            n1332 = property on="EnableTestind" class="Bool (strict)"() -> ("Value"=w2922:bool)  [unwired: 2 in, 2 out]
            n1333 = call "SerialMarvinMod.vi"("error in (no error)"=w2934, "write buffer"="SN\r\n", "VISA resource name"=w2937) -> ("error out"=w2913:errorcluster, "read buffer"=w2932:string)  [unwired: 7 in]
            n1334 = Decimal String To Number(string=w2932) -> (number=w2931:i32)  [unwired: 2 in, 1 out]
            n1335 = Equal?(x=w2931, y=0) -> (x = y?=w2928:bool)
            n1336 = Equal?(x=w2931, y=-1) -> (x = y?=w2927:bool)
            n1337 = Build Array(w2926, w2925, w2924, w2923, w2922, w2921, w2920, w2919, w2918) -> (w2917:bool[])
            n1338 = Compound Arithmetic op=OR(w2928, w2927) -> (w2907:bool)
            n1339 = And Array Elements(Boolean array=w2917) -> (logical AND=w2916:bool)
            n1340 = And(x=w2907, y=w2916) -> (x .and. y?=w2908:bool)
            n1341 = case shown="True" w2908 {
              tunnel: w2915 -> [_ w2972]
              tunnel: w2914 -> [_ w2970]
              tunnel: w2913 -> [w2946 w2969]
              tunnel: [w2947 w2956] -> w2912
              tunnel: w2909 -> [_ w2953]
              tunnel: w2907 -> [w2945 _]
              frame False {
                n1342 = case shown="True" w2945 {
                  tunnel: [w2948 w2950] -> w2947
                  tunnel: w2946 -> [w2948 w2949]
                  frame False {
                  }
                  frame True {
                    n1343 = call "Display Message to User5"("error in (no error)"=w2949) -> ("error out"=w2950:errorcluster)  [unwired: 9 in, 1 out]
                  }
                }
              }
              frame True {
                n1344 = VISA Flush I/O Buffer(VISA resource name=w2970, error in (no error)=w2969) -> (VISA resource name out=w2964:refnum<visa-resource-name>, error out=w2971:errorcluster)  [unwired: 1 in]
                n1345 = property on="Next SN" class="Str"() -> ("Value"=w2952:string)  [unwired: 2 in, 2 out]
                n1346 = Decimal String To Number(string=w2952) -> (number=w2951:i32)  [unwired: 2 in, 1 out]
                n1347 = Number To Decimal String(number=w2951) -> (decimal integer string=w2959:string)  [unwired: 1 in]
                n1348 = Concatenate Strings("EP=1\r\nSN=" ("write buffer"), w2959, "\r\n" ("string")) -> (w2966:string)
                n1349 = call "SerialMarvinMod.vi"("error in (no error)"=w2971, "Clear Log"=FALSE, "write buffer"=w2966, "VISA resource name"=w2964) -> ("error out"=w2963:errorcluster)  [unwired: 6 in, 1 out]
                n1350 = VISA Flush I/O Buffer(VISA resource name=w2964, error in (no error)=w2963) -> (VISA resource name out=w2962:refnum<visa-resource-name>, error out=w2965:errorcluster)  [unwired: 1 in]
                n1351 = call "SerialMarvinMod.vi"("error in (no error)"=w2965, "Clear Log"=FALSE, "write buffer"="SN\r\n", "VISA resource name"=w2962) -> ("error out"=w2957:errorcluster, "read buffer"=w2960:string)  [unwired: 6 in]
                n1352 = Equal?(x=w2960, y=w2959) -> (x = y?=w2958:bool)
                n1353 = case shown="True" w2958 {
                  tunnel: w2972 -> [_ w2986]
                  tunnel: w2959 -> [_ w2985]
                  tunnel: w2957 -> [w2973 w2976]
                  tunnel: [w2973 w2983] -> w2956
                  tunnel: w2951 -> [_ w2981]
                  tunnel: w2953 -> [_ w2979]
                  frame False {
                  }
                  frame True {
                    n1354 = call <vilib>:"Open Config Data.vi"("error in (no error)"=w2976, "create file if necessary (T)"=FALSE, "configuration file path"=w2979) -> ("error out"=w2977:errorcluster, "refnum"=w2978:T15)  [unwired: 7 out]
                    n1355 = Increment(x=w2981) -> (x+1=w2975:i32)
                    n1356 = Number To Decimal String(number=w2975) -> (decimal integer string=w2974:string)  [unwired: 1 in]
                    n1357 = property on="Next SN" class="Str"("Value"=w2974) -> ()  [unwired: 2 in, 2 out]
                    n1358 = call-poly <vilib>:"Write Key.vi"("section"="Marvin", "error in (no error)"=w2977, "value"=w2985, "key"=w2986, "refnum"=w2978) -> ("error out"=w2984:errorcluster, "refnum out"=w2982:T15)  [unwired: 4 in, 1 out]
                    n1359 = call <vilib>:"Close Config Data.vi"("error in (no error)"=w2984, "refnum"=w2982) -> ("error out"=w2983:errorcluster)  [unwired: 8 in, 1 out]
                  }
                }
              }
            }
            n1360 = call <vilib>:"Clear Errors.vi"("error in (no error)"=w2912) -> ("error out"=w2910:errorcluster)  [unwired: 5 in, 1 out]
            n1361 = property on="SetSN" class="Bool (strict)"(error in=w2910, "Value"=FALSE ("SetSN")) -> (error out=w2905:errorcluster)  [unwired: 1 in, 1 out]
            n1362 = property on="Report" class="Bool (strict)"(error in=w2905, "Value"=w2904, "Val(Sgnl)"=w2904) -> ()  [unwired: 1 in, 2 out]
          }
          event "ATR", "Pannel User Message": Mouse Enter {
            n1363 = event-data() -> ()  [unwired: 1 in, 4 out]
            n1364 = call-poly <vilib>:"Set Cursor.vi"("error in (no error)"=w3000, "icon"=u16 1) -> ("error out"=w3001:errorcluster)  [unwired: 8 in, 1 out]
          }
          event "ATR", "Pannel User Message": Mouse Leave {
            n1365 = event-data() -> ()  [unwired: 1 in, 4 out]
            n1366 = call-poly <vilib>:"Set Cursor.vi"("error in (no error)"=w3010, "icon"=u16 0) -> ("error out"=w3008:errorcluster)  [unwired: 8 in, 1 out]
          }
          event "ATR": Mouse Down? {
            n1367 = event-data() -> ("Coords"=w3025:T24)  [unwired: 1 in, 4 out]
            n1368 = invoke on="ATR" class="Tbl (strict)" method="Point To Row Column"("Point"=w3025) -> ("InBounds"=w3021:bool, "CellPosition"=w3020:T17)  [unwired: 5 in, 4 out]
            n1369 = Greater Than 0?(x=w3020) -> (x > 0?=w3024:cluster{"Row":bool, "Column":bool})
            n1370 = Cluster To Array(cluster=w3024) -> (array=w3023:bool[])
            n1371 = Or Array Elements(Boolean array=w3023) -> (logical OR=w3022:bool)
            n1372 = Compound Arithmetic op=OR(w3021, w3022) -> (w3019:bool)
            n1373 = event-data("Discard?"=w3019) -> ()  [unwired: 1 in, 1 out]
          }
          event "Start": Value Change {
            w3027 = FALSE ("Stop Button")
            (unwired) T19."Start"
            n1374 = event-data() -> ()  [unwired: 1 in, 2 out]
            n1375 = call <vilib>:"Clear Errors.vi"("error in (no error)"=w3047) -> ("error out"=w3033:errorcluster)  [unwired: 5 in, 1 out]
            n1376 = property on="UUT" class="Str"(error in=w3033) -> (error out=w3032:errorcluster, "Value"=w3046:string)  [unwired: 1 in, 1 out]
            n1377 = property on="ClosePanel" class="Bool (strict)"("Value"=w3027) -> ()  [unwired: 2 in, 2 out]
            n1378 = property on="Stop Button" class="Bool (strict)"("Value"=w3027) -> ()  [unwired: 2 in, 2 out]
            n1379 = while {
              tunnel: w3046 -> [w3055]
              tunnel: [w3054] -> w3040
              tunnel: [w3053] -> w3034
              tunnel: w3032 -> [w3051]
              shift-right: [w3050] -> _
              shift-left: T19."Verify VR" -> [w3052]
              stop <- w3049 stop-if-true
              n1380 = case shown="\"Verify UUT\"" w3052 {
                tunnel: w3055 -> [_ w3071 w3190 w3216]
                tunnel: [w3060 w3070 w3184 w3235] -> w3054
                tunnel: [w3062 w3069 w3191 w3257] -> w3053
                tunnel: w3051 -> [w3059 _ w3188 w3252]
                tunnel: [T19."End" T19."Start" w3192 w3229] -> w3050
                tunnel: [w3061 TRUE w3185 w3223] -> w3049
                frame "End", Default {
                  w3062 = T1 [] items=["Auxiliary", "Temp Sens Cal", "Com Test", "Enable Test", "Speed Command", "Stop Time", "Temp Control", "Burn in", "Visual Inspec", "Empty"]
                  n1381 = call "Display Message to User10"("error in (no error)"=w3059) -> ("error out"=w3056:errorcluster)  [unwired: 9 in, 1 out]
                  n1382 = property on="Refresh Button" class="Bool (strict)"(error in=w3056, "Val(Sgnl)"=TRUE ("Value (Signaling)")) -> (error out=w3057:errorcluster)  [unwired: 1 in, 1 out]
                  n1383 = flat-sequence {
                    tunnel: w3057 -> [w3064]
                    tunnel: [TRUE] -> w3061
                    tunnel: [w3064] -> w3060
                    frame #0 {
                    }
                  }
                }
                frame "Start" {
                  n1384 = case shown="\"EBAY\"" w3071 {
                    tunnel: [w3084 w3135] -> w3069
                    tunnel: [w3083 w3134] -> w3070
                    tunnel: [w3072 w3122] -> w3066
                    frame "AHU", Default {
                      n1385 = call "Load Program Process AHU.vi"() -> ("Speed Command Test"=w3077:bool, "Enable Test"=w3078:bool, "Burn-in Test"=w3075:bool, "Auxiliary"=w3073:bool, "Temperature Sensor Calibration Test"=w3080:bool, "Communication Test"=w3079:bool, "Motor Temperature Test"=w3076:bool, "Visual Inspection"=w3074:bool, "OK"=w3081:bool, "Automation"=w3072:bool, "error out"=w3083:errorcluster)  [unwired: 8 in, 9 out]
                      n1386 = Compound Arithmetic op=OR(w3081, w3072) -> (w3082:bool)
                      n1387 = case shown="True" w3082 {
                        tunnel: [w3085 w3095] -> w3084
                        tunnel: w3072 -> [_ w3094]
                        tunnel: w3080 -> [_ w3093]
                        tunnel: w3079 -> [_ w3092]
                        tunnel: w3078 -> [_ w3091]
                        tunnel: w3077 -> [_ w3090]
                        tunnel: w3076 -> [_ w3089]
                        tunnel: w3075 -> [_ w3088]
                        tunnel: w3074 -> [_ w3087]
                        tunnel: w3073 -> [_ w3086]
                        frame False {
                          w3085 = T1 [] items=["Auxiliary", "Temp Sens Cal", "Com Test", "Enable Test", "Speed Command", "Stop Time", "Temp Control", "Burn in", "Visual Inspec", "Empty"]
                        }
                        frame True {
                          n1388 = case shown="False" w3094 {
                            tunnel: [w3120 w3121] -> w3095
                            tunnel: w3093 -> [w3112 _]
                            tunnel: w3092 -> [w3111 _]
                            tunnel: w3091 -> [w3110 _]
                            tunnel: w3090 -> [w3109 _]
                            tunnel: w3089 -> [w3108 _]
                            tunnel: w3088 -> [w3107 _]
                            tunnel: w3087 -> [w3106 _]
                            tunnel: w3086 -> [w3105 _]
                            frame False {
                              w3103 = T2."Empty" ("f")
                              n1389 = Select(t=T2."Temp Sens Cal" ("f"), s=w3112, f=w3103) -> (s? t:f=w3097:T2)
                              n1390 = Select(t=T2."Com Test" ("f"), s=w3111, f=w3103) -> (s? t:f=w3096:T2)
                              n1391 = Select(t=T2."Enable Test" ("f"), s=w3110, f=w3103) -> (s? t:f=w3099:T2)
                              n1392 = Select(t=T2."Speed Command" ("f"), s=w3109, f=w3103) -> (s? t:f=w3100:T2)
                              n1393 = Select(t=T2."Stop Time" ("f"), s=w3108, f=w3103) -> (s? t:f=w3098:T2)
                              n1394 = Select(t=T2."Burn in" ("f"), s=w3107, f=w3103) -> (s? t:f=w3101:T2)
                              n1395 = Select(t=T2."Auxiliary" ("f"), s=w3105, f=w3103) -> ()  [unwired: 1 out]
                              n1396 = Select(t=T2."Visual Inspec" ("f"), s=w3106, f=w3103) -> (s? t:f=w3102:T2)
                              n1397 = Build Array(w3096, w3097, w3098, w3099, w3100, w3101, w3102) -> (w3120:T1)
                            }
                            frame True {
                              w3121 = T1 [enum."Com Test", enum."Temp Sens Cal", enum."Stop Time", enum."Enable Test", enum."Speed Command", enum."Burn in", enum."Visual Inspec"] items=["Auxiliary", "Temp Sens Cal", "Com Test", "Enable Test", "Speed Command", "Stop Time", "Temp Control", "Burn in", "Visual Inspec", "Empty"]
                            }
                          }
                        }
                      }
                    }
                    frame "EBAY" {
                      n1398 = call "Load Program Process EBAY.vi"() -> ("Speed Command Test"=w3128:bool, "Enable Test"=w3129:bool, "Burn-in Test"=w3126:bool, "Temperature Control Algorithm Test"=w3125:bool, "Auxiliary"=w3123:bool, "Temperature Sensor Calibration Test"=w3131:bool, "Communication Test"=w3130:bool, "Motor Temperature Test"=w3127:bool, "Visual Inspection"=w3124:bool, "OK"=w3132:bool, "Automation"=w3122:bool, "error out"=w3134:errorcluster)  [unwired: 8 in, 8 out]
                      n1399 = Compound Arithmetic op=OR(w3132, w3122) -> (w3133:bool)
                      n1400 = case shown="True" w3133 {
                        tunnel: [w3136 w3147] -> w3135
                        tunnel: w3122 -> [_ w3146]
                        tunnel: w3131 -> [_ w3145]
                        tunnel: w3130 -> [_ w3144]
                        tunnel: w3129 -> [_ w3143]
                        tunnel: w3128 -> [_ w3142]
                        tunnel: w3127 -> [_ w3141]
                        tunnel: w3126 -> [_ w3140]
                        tunnel: w3125 -> [_ w3139]
                        tunnel: w3124 -> [_ w3138]
                        tunnel: w3123 -> [_ w3137]
                        frame False {
                          w3136 = T1 [] items=["Auxiliary", "Temp Sens Cal", "Com Test", "Enable Test", "Speed Command", "Stop Time", "Temp Control", "Burn in", "Visual Inspec", "Empty"]
                        }
                        frame True {
                          n1401 = case shown="False" w3146 {
                            tunnel: [w3176 w3177] -> w3147
                            tunnel: w3145 -> [w3167 _]
                            tunnel: w3144 -> [w3166 _]
                            tunnel: w3143 -> [w3165 _]
                            tunnel: w3142 -> [w3164 _]
                            tunnel: w3141 -> [w3154 _]
                            tunnel: w3140 -> [w3159 _]
                            tunnel: w3139 -> [w3158 _]
                            tunnel: w3138 -> [w3163 _]
                            tunnel: w3137 -> [w3162 _]
                            frame False {
                              w3160 = T2."Empty" ("f")
                              n1402 = Select(t=T2."Temp Sens Cal" ("f"), s=w3167, f=w3160) -> (s? t:f=w3149:T2)
                              n1403 = Select(t=T2."Com Test" ("f"), s=w3166, f=w3160) -> (s? t:f=w3148:T2)
                              n1404 = Select(t=T2."Enable Test" ("f"), s=w3165, f=w3160) -> (s? t:f=w3151:T2)
                              n1405 = Select(t=T2."Speed Command" ("f"), s=w3164, f=w3160) -> (s? t:f=w3152:T2)
                              n1406 = Select(t=T2."Stop Time" ("f"), s=w3154, f=w3160) -> (s? t:f=w3150:T2)
                              n1407 = Select(t=T2."Temp Control" ("f"), s=w3158, f=w3160) -> (s? t:f=w3153:T2)
                              n1408 = Select(t=T2."Burn in" ("f"), s=w3159, f=w3160) -> (s? t:f=w3155:T2)
                              n1409 = Select(t=T2."Visual Inspec" ("f"), s=w3163, f=w3160) -> (s? t:f=w3157:T2)
                              n1410 = Select(t=T2."Auxiliary" ("f"), s=w3162, f=w3160) -> (s? t:f=w3156:T2)
                              n1411 = Build Array(w3148, w3149, w3150, w3151, w3152, w3153, w3155, w3156, w3157) -> (w3176:T1)
                            }
                            frame True {
                              w3177 = T1 [enum."Com Test", enum."Temp Sens Cal", enum."Stop Time", enum."Enable Test", enum."Speed Command", enum."Temp Control", enum."Burn in", enum."Auxiliary", enum."Visual Inspec"] items=["Auxiliary", "Temp Sens Cal", "Com Test", "Enable Test", "Speed Command", "Stop Time", "Temp Control", "Burn in", "Visual Inspec", "Empty"]
                              # "Temp control - empty"
                            }
                          }
                        }
                      }
                    }
                  }
                  "Automation" <- w3066
                }
                frame "Verify VR" {
                  w3191 = T1 [] items=["Auxiliary", "Temp Sens Cal", "Com Test", "Enable Test", "Speed Command", "Stop Time", "Temp Control", "Burn in", "Visual Inspec", "Empty"]
                  n1412 = control-ref of="Stop Button"() -> (w3180:refnum<vi>)
                  n1413 = property on="Serial" class="Bool (strict)"(error in=w3188) -> (error out=w3187:errorcluster, "Value"=w3186:bool)  [unwired: 1 in, 1 out]
                  n1414 = control-ref of="Pannel User Message"() -> (w3181:refnum<vi>)
                  n1415 = case shown="True" w3186 {
                    tunnel: w3187 -> [w3196 w3206]
                    tunnel: [T19."Verify VR" w3200] -> w3192
                    tunnel: w3190 -> [_ w3205]
                    tunnel: [w3194 w3199] -> w3189
                    tunnel: [TRUE FALSE] -> w3185
                    frame False {
                      n1416 = call "Display Message to User9"("error in (no error)"=w3196) -> ("error out"=w3194:errorcluster)  [unwired: 9 in, 1 out]
                    }
                    frame True {
                      n1417 = property on="VISA resource name" class="VISAName"() -> ("Value"=w3208:refnum<visa-resource-name>)  [unwired: 2 in, 2 out]
                      n1418 = case shown="\"EBAY\"" w3205 {
                        tunnel: ["5.3.8d" ("write buffer") "5.3.9" ("write buffer")] -> w3203
                        frame "AHU", Default {
                        }
                        frame "EBAY" {
                        }
                      }
                      n1419 = VISA Flush I/O Buffer(VISA resource name=w3208, error in (no error)=w3206) -> (VISA resource name out=w3210:refnum<visa-resource-name>, error out=w3209:errorcluster)  [unwired: 1 in]
                      n1420 = call "SerialMarvinMod.vi"("error in (no error)"=w3209, "write buffer"="VR\r\n", "VISA resource name"=w3210) -> ("error out"=w3199:errorcluster, "read buffer"=w3204:string)  [unwired: 7 in]
                      n1421 = Equal?(x=w3204, y=w3203) -> (x = y?=w3198:bool)
                      n1422 = Select(t=T19."Verify UUT", s=w3198, f=T19."End") -> (s? t:f=w3200:T19)
                    }
                  }
                  n1423 = control-ref of="Motor Speed RPM"() -> (w3178:refnum<vi>)
                  n1424 = call "Write panel message (SubVI).vi"("rpm"=w3178, "PrintTime"=FALSE, "Stop"=w3180, "error in (no error)"=w3189, "Time to wait"=0.1, "Strin"="TESTER BIT TEST OPERATION IN PROCESS", "String in"=w3181) -> ("error out"=w3184:errorcluster)  [unwired: 4 in]
                }
                frame "Verify UUT" {
                  w3238 = FALSE ("Clear Log")
                  w3257 = T1 [] items=["Auxiliary", "Temp Sens Cal", "Com Test", "Enable Test", "Speed Command", "Stop Time", "Temp Control", "Burn in", "Visual Inspec", "Empty"]
                  # "25 C"
                  n1425 = property on="VISA resource name" class="VISAName"() -> ("Value"=w3254:refnum<visa-resource-name>)  [unwired: 2 in, 2 out]
                  n1426 = Equal?(x=w3216, y="EBAY") -> (x = y?=w3214:bool)
                  n1427 = VISA Flush I/O Buffer(VISA resource name=w3254, error in (no error)=w3252) -> (VISA resource name out=w3256:refnum<visa-resource-name>, error out=w3255:errorcluster)  [unwired: 1 in]
                  n1428 = control-ref of="VISA resource name out"() -> (w3249:refnum<vi>)
                  n1429 = call "SerialMarvinMod.vi"("error in (no error)"=w3255, "Clear Log"=w3238, "write buffer"="TA[1]\r\n", "VISA resource name"=w3256) -> ("error out"=w3240:errorcluster, "read buffer"=w3234:string)  [unwired: 6 in]
                  n1430 = case shown="True" w3214 {
                    tunnel: [w3300 w3304] -> w3217
                    tunnel: [i32[] [2] i32[] [1, 2]] -> w3213
                    frame False {
                      # "Cur"
                      n1431 = Byte Array To String(unsigned byte array=u8[] [75, 0, 4, 17, 0, 0, 0, 0] ("appended array")) -> (string=w3301:string)
                      n1432 = Build Array(w3301) -> (w3300:string[])
                    }
                    frame True {
                      # "Cur"
                      # "EBAYFAN"
                      n1433 = Byte Array To String(unsigned byte array=u8[] [75, 0, 4, 18, 0, 0, 0, 0] ("appended array")) -> (string=w3305:string)
                      n1434 = Byte Array To String(unsigned byte array=u8[] [75, 0, 4, 17, 0, 0, 0, 0] ("appended array")) -> (string=w3306:string)
                      n1435 = Build Array(w3305, w3306) -> (w3304:string[])
                    }
                  }
                  n1436 = property class="VISAName"(reference=w3249, error in=w3240) -> (error out=w3250:errorcluster, "Value"=w3251:refnum<visa-resource-name>)  [unwired: 1 out]
                  n1437 = Byte Array To String(unsigned byte array=u8[] [75, 0, 4, 2, 8, 0, 0, 0] ("appended array")) -> (string=w3247:string)
                  n1438 = property on="VISA resource name" class="VISAName"() -> ("Value"=w3245:refnum<visa-resource-name>)  [unwired: 2 in, 2 out]
                  n1439 = VISA Write(VISA resource name=w3251, write buffer=w3247, error in (no error)=w3250) -> (error out=w3242:errorcluster)  [unwired: 2 out]
                  n1440 = call <vilib>:"Clear Errors.vi"("error in (no error)"=w3242) -> ("error out"=w3241:errorcluster)  [unwired: 5 in, 1 out]
                  n1441 = call "Time Delay10"("error in (no error)"=w3241) -> ("error out"=w3219:errorcluster)  [unwired: 10 in]
                  n1442 = VISA Flush I/O Buffer(VISA resource name=w3245, error in (no error)=w3219) -> (VISA resource name out=w3243:refnum<visa-resource-name>, error out=w3244:errorcluster)  [unwired: 1 in]
                  n1443 = call "SerialMarvinMod.vi"("error in (no error)"=w3244, "Clear Log"=w3238, "write buffer"="TA[2]\r\n", "VISA resource name"=w3243) -> ("error out"=w3239:errorcluster, "read buffer"=w3233:string)  [unwired: 6 in]
                  n1444 = call "Time Delay9"("error in (no error)"=w3239) -> ("error out"=w3220:errorcluster)  [unwired: 10 in]
                  n1445 = case shown="True" w3214 {
                    tunnel: w3238 -> [_ w3287]
                    tunnel: [w3281 w3286] -> w3237
                    tunnel: ["" ("read buffer") w3285] -> w3232
                    tunnel: w3220 -> [w3281 w3284]
                    frame False {
                    }
                    frame True {
                      # "K17"
                      n1446 = control-ref of="VISA resource name out"() -> (w3296:refnum<vi>)
                      n1447 = property class="VISAName"(reference=w3296, error in=w3284) -> (error out=w3295:errorcluster, "Value"=w3294:refnum<visa-resource-name>)  [unwired: 1 out]
                      n1448 = Byte Array To String(unsigned byte array=u8[] [75, 0, 4, 2, 0, 0, 1, 0] ("appended array")) -> (string=w3298:string)
                      n1449 = VISA Write(VISA resource name=w3294, write buffer=w3298, error in (no error)=w3295) -> (error out=w3289:errorcluster)  [unwired: 2 out]
                      n1450 = property on="VISA resource name" class="VISAName"() -> ("Value"=w3291:refnum<visa-resource-name>)  [unwired: 2 in, 2 out]
                      n1451 = call <vilib>:"Clear Errors.vi"("error in (no error)"=w3289) -> ("error out"=w3288:errorcluster)  [unwired: 5 in, 1 out]
                      n1452 = call "Time Delay11"("error in (no error)"=w3288) -> ("error out"=w3283:errorcluster)  [unwired: 10 in]
                      n1453 = VISA Flush I/O Buffer(VISA resource name=w3291, error in (no error)=w3283) -> (VISA resource name out=w3293:refnum<visa-resource-name>, error out=w3292:errorcluster)  [unwired: 1 in]
                      n1454 = call "SerialMarvinMod.vi"("error in (no error)"=w3292, "Clear Log"=w3287, "write buffer"="TA[3]\r\n", "VISA resource name"=w3293) -> ("error out"=w3286:errorcluster, "read buffer"=w3285:string)  [unwired: 6 in]
                    }
                  }
                  n1455 = for {
                    tunnel: [w3312] -> w3231 mode=indexing
                    tunnel: w3217 -> [w3310] mode=indexing
                    tunnel: w3237 -> [w3319]
                    tunnel: [w3313] -> w3236
                    tunnel: w3213 -> [w3309] mode=indexing
                    n1456 = call <vilib>:"Clear Errors.vi"("error in (no error)"=w3315) -> ("error out"=w3317:errorcluster)  [unwired: 5 in, 1 out]
                    n1457 = control-ref of="VISA resource name out"() -> (w3320:refnum<vi>)
                    n1458 = property class="VISAName"(reference=w3320, error in=w3319) -> (error out=w3321:errorcluster, "Value"=w3322:refnum<visa-resource-name>)  [unwired: 1 out]
                    n1459 = VISA Write(VISA resource name=w3322, write buffer=w3310, error in (no error)=w3321) -> (VISA resource name out=w3318:refnum<visa-resource-name>, error out=w3316:errorcluster)  [unwired: 1 out]
                    n1460 = while {
                      tunnel: w3317 -> [w3337]
                      tunnel: [w3336] -> _
                      tunnel: w3314 -> [w3334]
                      tunnel: [w3329] -> _
                      tunnel: w3318 -> [w3328]
                      tunnel: [w3327] -> w3313
                      tunnel: [w3326] -> w3312
                      tunnel: w3309 -> [w3325]
                      stop <- w3330 stop-if-true
                      n1461 = VISA Read(VISA resource name=w3328, byte count=u32 1, error in (no error)=w3337) -> (VISA resource name out=w3339:refnum<visa-resource-name>, read buffer=w3340:string, error out=w3338:errorcluster)  [unwired: 1 out]
                      n1462 = String To Byte Array(string=w3340) -> (unsigned byte array=w3343:u8[])
                      n1463 = call <vilib>:"High Resolution Relative Seconds.vi"() -> ("relative seconds"=w3335:dbl)
                      n1464 = Index Array(array=w3343, index=0) -> (element=w3341:u8)
                      n1465 = Subtract(x=w3335, y=w3334) -> (x-y=w3333:dbl)
                      n1466 = case shown="75" w3341 {
                        tunnel: [w3348 w3353] -> w3327
                        tunnel: w3339 -> [w3347 w3362]
                        tunnel: w3338 -> [w3348 w3361]
                        tunnel: [w3347 w3354] -> w3336
                        tunnel: [u32 9999 w3351] -> w3329
                        tunnel: [FALSE w3350] -> w3326
                        tunnel: w3325 -> [_ w3349]
                        frame 0, Default {
                        }
                        frame 75 {
                          n1467 = VISA Read(VISA resource name=w3362, byte count=u32 3, error in (no error)=w3361) -> (VISA resource name out=w3357:refnum<visa-resource-name>, read buffer=w3365:string, error out=w3356:errorcluster)  [unwired: 1 out]
                          n1468 = String To Byte Array(string=w3365) -> (unsigned byte array=w3355:u8[])
                          n1469 = Index Array(array=w3355, index #1=0 ("index")) -> (element #1=w3360:u8, element #2=w3358:u8)  [unwired: 2 in, 1 out]
                          n1470 = Equal?(x=u8 0, y=w3360) -> (x = y?=w3359:bool)
                          n1471 = case shown="True" w3359 {
                            tunnel: [w3368 w3376] -> w3353
                            tunnel: w3358 -> [_ w3383]
                            tunnel: w3357 -> [w3369 w3382]
                            tunnel: w3356 -> [w3368 w3381]
                            tunnel: w3355 -> [_ w3380]
                            tunnel: [w3369 w3378] -> w3354
                            tunnel: [u32 9999 w3372] -> w3351
                            tunnel: [FALSE w3371] -> w3350
                            tunnel: w3349 -> [_ w3370]
                            frame False {
                            }
                            frame True {
                              n1472 = VISA Read(VISA resource name=w3382, byte count=w3383, error in (no error)=w3381) -> (VISA resource name out=w3378:refnum<visa-resource-name>, read buffer=w3377:string, error out=w3376:errorcluster)  [unwired: 1 out]
                              n1473 = String To Byte Array(string=w3377) -> (unsigned byte array=w3379:u8[])
                              n1474 = Insert Into Array(array=w3380, new element=w3379) -> (w3373:u8[])  [unwired: 1 in]
                              n1475 = Index Array(array=w3373, index #1=0 ("index")) -> (element #3=w3374:u8)  [unwired: 2 in, 2 out]
                              n1476 = case shown="15..19" w3374 {
                                tunnel: w3373 -> [_ w3395]
                                tunnel: [u32 9999 w3387] -> w3372
                                tunnel: [FALSE w3388] -> w3371
                                tunnel: w3370 -> [_ w3386]
                                frame 0, Default {
                                }
                                frame 15..19 {
                                n1477 = Index Array(array=w3395, index #1=3 ("index")) -> (element #1=w3394:u8, element #2=w3393:u8, element #3=w3392:u8, element #4=w3391:u8)  [unwired: 3 in]
                                n1478 = Join Numbers(hi=w3393, lo=w3394) -> ((hi.lo)=w3390:u16)
                                n1479 = Join Numbers(hi=w3391, lo=w3392) -> ((hi.lo)=w3389:u16)
                                n1480 = Join Numbers(hi=w3389, lo=w3390) -> ((hi.lo)=w3387:u32)
                                n1481 = case shown="1" w3386 {
                                tunnel: [w3397 w3401] -> w3388
                                tunnel: w3387 -> [w3399 w3400]
                                frame 2, Default {
                                n1482 = Less Or Equal?(x=w3399, y=u32 50) -> (x <= y?=w3397:bool)
                                }
                                frame 1 {
                                n1483 = Greater Or Equal?(x=w3400, y=2200.0) -> (x >= y?=w3401:bool)
                                }
                                }
                                }
                              }
                            }
                          }
                        }
                      }
                      n1484 = Greater Or Equal?(x=w3333, y=5.0) -> (x >= y?=w3331:bool)
                      n1485 = Compound Arithmetic op=OR(w3331, w3326) -> (w3330:bool)
                    }
                    n1486 = call "Time Delay12"("error in (no error)"=w3316) -> ("error out"=w3311:errorcluster)  [unwired: 10 in]
                    n1487 = flat-sequence {
                      tunnel: w3311 -> [w3324]
                      tunnel: [w3324] -> w3315
                      tunnel: [w3323] -> w3314
                      frame #0 {
                        n1488 = call <vilib>:"High Resolution Relative Seconds.vi"() -> ("relative seconds"=w3323:dbl)
                      }
                    }
                  }
                  n1489 = call <vilib>:"Clear Errors.vi"("error in (no error)"=w3236) -> ("error out"=w3235:errorcluster)  [unwired: 5 in, 1 out]
                  n1490 = case shown="False" w3214 {
                    tunnel: w3234 -> [w3267 w3280]
                    tunnel: w3233 -> [w3266 w3279]
                    tunnel: w3232 -> [_ w3278]
                    tunnel: w3231 -> [w3260 w3270]
                    tunnel: [w3259 w3269] -> w3227
                    tunnel: [string[] ["TA[1] OPERATION FAILED!", "TA[2] OPERATION FAILED!", "CURRENT OPERATION FAILED!"] string[] ["TA[1] OPERATION FAILED!", "TA[2] OPERATION FAILED!", "TA[3] OPERATION FAILED!", "EBAY FAN OPERATION FAILED!", "CURRENT OPERATION FAILED!"]] -> w3226
                    frame False {
                      w3263 = 100.0 ("y")
                      n1491 = Fract/Exp String To Number(string=w3267) -> (number=w3265:dbl)  [unwired: 3 in, 1 out]
                      n1492 = Fract/Exp String To Number(string=w3266) -> (number=w3264:dbl)  [unwired: 3 in, 1 out]
                      n1493 = Less Or Equal?(x=w3265, y=w3263) -> (x <= y?=w3262:bool)
                      n1494 = Less Or Equal?(x=w3264, y=w3263) -> (x <= y?=w3261:bool)
                      n1495 = Build Array (concatenate)(w3262, w3261, w3260) -> (w3259:bool[])
                    }
                    frame True {
                      w3274 = 100.0 ("y")
                      n1496 = Fract/Exp String To Number(string=w3280) -> (number=w3277:dbl)  [unwired: 3 in, 1 out]
                      n1497 = Fract/Exp String To Number(string=w3279) -> (number=w3276:dbl)  [unwired: 3 in, 1 out]
                      n1498 = Fract/Exp String To Number(string=w3278) -> (number=w3275:dbl)  [unwired: 3 in, 1 out]
                      n1499 = Less Or Equal?(x=w3277, y=w3274) -> (x <= y?=w3273:bool)
                      n1500 = Less Or Equal?(x=w3276, y=w3274) -> (x <= y?=w3272:bool)
                      n1501 = Less Or Equal?(x=w3275, y=w3274) -> (x <= y?=w3271:bool)
                      n1502 = Build Array (concatenate)(w3273, w3272, w3271, w3270) -> (w3269:bool[])
                    }
                  }
                  n1503 = for {
                    tunnel: w3227 -> [w3409] mode=indexing
                    tunnel: w3226 -> [w3408] mode=indexing
                    shift-right: [w3406] -> w3224
                    shift-left: "" -> [w3407]
                    n1504 = case shown="False" w3409 {
                      tunnel: w3408 -> [w3412 _]
                      tunnel: w3407 -> [w3413 w3414]
                      tunnel: [w3410 w3414] -> w3406
                      frame False {
                        n1505 = Concatenate Strings(w3413, w3412, "\r\n") -> (w3410:string)
                      }
                      frame True {
                      }
                    }
                  }
                  n1506 = And Array Elements(Boolean array=w3227) -> (logical AND=w3218:bool)
                  n1507 = Not(x=w3218) -> (.not. x?=w3221:bool)
                  n1508 = Select(t=T19."Start", s=w3218, f=T19."End") -> (s? t:f=w3229:T19)
                  n1509 = case shown="True" w3218 {
                    tunnel: w3224 -> [w3404 _]
                    tunnel: [w3403 FALSE ("true")] -> w3222
                    frame False {
                      n1510 = One Button Dialog(message=w3404) -> (true=w3403:bool)  [unwired: 1 in]
                    }
                    frame True {
                    }
                  }
                  n1511 = And(x=w3222, y=w3221) -> (x .and. y?=w3223:bool)
                }
              }
            }
            n1512 = Bundle By Name(cluster=T10 {"VISA"="COM1", "Array Test"=[]}, "VISA"=w3041, "Array Test"=w3034) -> (w3036:T10)
            n1513 = property on="Serial" class="Bool (strict)"() -> ("Value"=w3037:bool)  [unwired: 2 in, 2 out]
            n1514 = case shown="False" w3037 {
              tunnel: w3034 -> [w3415 _]
              tunnel: w3036 -> [w3417 w3427]
              tunnel: [w3416 w3427] -> w3035
              frame False {
                n1515 = for {
                  tunnel: w3415 -> [w3426] mode=indexing
                  tunnel: [w3421] -> w3418
                  stop <- w3421 stop-if-true
                  n1516 = Equal?(x=w3426, y=T2."Temp Sens Cal") -> (x = y?=w3423:bool)
                  n1517 = Equal?(x=w3426, y=T2."Enable Test") -> (x = y?=w3422:bool)
                  n1518 = Or(x=w3423, y=w3422) -> (x .or. y?=w3421:bool)
                }
                n1519 = case shown="True" w3418 {
                  tunnel: w3417 -> [w3419 _]
                  tunnel: [w3419 T10 {"VISA"="COM1", "Array Test"=[]}] -> w3416
                  frame False {
                  }
                  frame True {
                    n1520 = call "Display Message to User8"() -> ()  [unwired: 10 in, 2 out]
                  }
                }
              }
              frame True {
              }
            }
            n1521 = Enqueue Element(queue=w3043, element=w3035, error in (no error)=w3040) -> (queue out=w3039:refnum<queue>, error out=w3030:errorcluster)  [unwired: 2 out]
            n1522 = property on="Start" class="Bool (strict)"(error in=w3030, "Value"=FALSE ("Start")) -> (error out=w3029:errorcluster)  [unwired: 1 in, 1 out]
          }
          event "Report", "Stop Button": Value Change {
            w3449 = "Marvin" ("section")
            w3461 = "_"
            # "EBAY 414-8005\nAHU-L (47) P/N 413-8005-1\nAHU-R (63) P/N 413-8005-2"
            n1523 = event-data() -> ("CtlRef"=w3441:refnum<vi>)  [unwired: 1 in, 5 out]
            n1524 = call <vilib>:"Application Directory.vi"() -> ("Application Directory"=w3483:path)
            n1525 = Build Path(base path=w3483, name or relative path="Reports") -> (appended path=w3486:path)
            n1526 = property on="Serial" class="Bool (strict)"() -> ("Value"=w3446:bool)  [unwired: 2 in, 2 out]
            n1527 = call <vilib>:"Open Config Data.vi"("create file if necessary (T)"=FALSE, "configuration file path"=w3455) -> ("refnum"=w3457:T15)  [unwired: 1 in, 8 out]
            n1528 = Get Date/Time String(want seconds? (F)=TRUE) -> (date string=w3488:string)  [unwired: 2 in, 1 out]
            n1529 = Search and Replace String(replace all?=TRUE ("replace all? (F)"), input string=w3488, search string="/") -> (result string=w3460:string)  [unwired: 5 in, 3 out]
            n1530 = property on="Report" class="Bool (strict)"("Value"=FALSE ("Report")) -> ()  [unwired: 2 in, 2 out]
            n1531 = local read "UUT"() -> (w3445:string)
            n1532 = case shown="\"EBAY\", Default" w3445 {
              tunnel: ["REV EBAY" ("key") "REV AHU" ("key")] -> w3444
              frame "EBAY", Default {
              }
              frame "AHU" {
              }
            }
            n1533 = call-poly <vilib>:"Read Key.vi"("section"=w3449, "key"=w3444, "refnum"=w3457) -> ("error out"=w3451:errorcluster, "value"=w3454:string, "refnum out"=w3453:T15)  [unwired: 5 in, 1 out]
            n1534 = call-poly <vilib>:"Read Key.vi"("section"=w3449, "error in (no error)"=w3451, "key"="Tester Software Ver", "refnum"=w3453) -> ("error out"=w3448:errorcluster, "value"=w3447:string, "refnum out"=w3452:T15)  [unwired: 4 in, 1 out]
            n1535 = call <vilib>:"Close Config Data.vi"("error in (no error)"=w3448, "refnum"=w3452) -> ()  [unwired: 8 in, 2 out]
            n1536 = control-ref of="ATR"() -> (w3495:refnum<vi>)
            n1537 = Concatenate Strings("  Rev-" ("string"), w3454) -> (w3459:string)
            n1538 = property class="Bool (strict)"(reference=w3441) -> ("BoolText.Text"=w3440:string)  [unwired: 1 in, 2 out]
            n1539 = Equal?(x=w3440, y="Report") -> (x = y?=w3435:bool)
            n1540 = case shown="False" w3446 {
              tunnel: w3472 -> [w3521 w3544]
              tunnel: ["N_A" ("read buffer") w3528] -> w3462
              tunnel: [w3525 w3532] -> w3471
              tunnel: w3468 -> [_ w3542]
              tunnel: [w3524 w3535] -> w3467
              tunnel: [w3524 w3533] -> w3465
              tunnel: [w3524 w3531] -> w3464
              tunnel: ["N_A" w3530] -> w3443
              tunnel: w3435 -> [w3520 _]
              frame False {
                w3524 = "N/A" ("read buffer")
                n1541 = case shown="True" w3520 {
                  tunnel: [w3526 w3527] -> w3525
                  tunnel: w3521 -> [w3526 _]
                  frame False {
                  }
                  frame True {
                    n1542 = call "Display Message to User12"() -> ("error out"=w3527:errorcluster)  [unwired: 10 in, 1 out]
                  }
                }
              }
              frame True {
                n1543 = call <vilib>:"Clear Errors.vi"("error in (no error)"=w3544) -> ("error out"=w3546:errorcluster)  [unwired: 5 in, 1 out]
                n1544 = VISA Flush I/O Buffer(VISA resource name=w3542, error in (no error)=w3546) -> (VISA resource name out=w3536:refnum<visa-resource-name>, error out=w3547:errorcluster)  [unwired: 1 in]
                n1545 = call "SerialMarvinMod.vi"("error in (no error)"=w3547, "write buffer"="SN\r\n", "VISA resource name"=w3536) -> ("error out"=w3543:errorcluster, "read buffer"=w3528:string)  [unwired: 7 in]
                n1546 = call <vilib>:"Clear Errors.vi"("error in (no error)"=w3543) -> ("error out"=w3537:errorcluster)  [unwired: 5 in, 1 out]
                n1547 = VISA Flush I/O Buffer(VISA resource name=w3536, error in (no error)=w3537) -> (VISA resource name out=w3538:refnum<visa-resource-name>, error out=w3539:errorcluster)  [unwired: 1 in]
                n1548 = call "SerialMarvinMod.vi"("error in (no error)"=w3539, "write buffer"="VR\r\n", "VISA resource name"=w3538) -> ("error out"=w3541:errorcluster, "read buffer"=w3535:string)  [unwired: 7 in]
                n1549 = call <vilib>:"Clear Errors.vi"("error in (no error)"=w3541) -> ("error out"=w3534:errorcluster)  [unwired: 5 in, 1 out]
                n1550 = property on="UUT" class="DigNum (strict)"(error in=w3534) -> (error out=w3532:errorcluster, "Value"=w3529:u8)  [unwired: 1 in, 1 out]
                n1551 = case shown="63" w3529 {
                  tunnel: ["EBAY 414-8005            " "AHU-L (47) 413-8005-1" "AHU-R (63) 413-8005-2"] -> w3533
                  tunnel: ["414-8005-95" " 413-8005-1-47" " 413-8005-2-63"] -> w3531
                  tunnel: ["414-8005_95_EBAY" " 413-8005_47_AHU" " 413-8005_63_AHU"] -> w3530
                  frame 95, Default {
                    (unwired) "AHU-R (63) 413-8005-2"
                  }
                  frame 47 {
                  }
                  frame 63 {
                  }
                }
              }
            }
            n1552 = call <vilib>:"Check if File or Folder Exists.vi"("error in (no error)"=w3471, "path"=w3486) -> ("error out"=w3484:errorcluster, "file or folder exists?"=w3487:bool, "dup path"=w3485:path)  [unwired: 7 in]
            n1553 = case shown="False" w3487 {
              tunnel: w3484 -> [w3560 w3561]
              tunnel: w3485 -> [w3559 w3562]
              tunnel: [w3558 w3562] -> w3493
              tunnel: [w3557 w3561] -> w3489
              frame False {
                n1554 = Create Folder(path (use dialog)=w3559, error in=w3560) -> (created path=w3558:path, error out=w3557:errorcluster)  [unwired: 1 in, 1 out]
              }
              frame True {
              }
            }
            n1555 = property on="Logger Path" class="Path"(error in=w3489, "Value"=w3493, "StartPath"=w3493) -> (error out=w3490:errorcluster)  [unwired: 1 in, 1 out]
            n1556 = Concatenate Strings("ATR" ("string"), w3443, w3461, w3462, w3461, w3460, ".docx" ("string")) -> (w3434:string)
            n1557 = property on="Logger Path" class="Path"(error in=w3490) -> (error out=w3491:errorcluster, "StartPath"=w3430:path)  [unwired: 1 in, 1 out]
            n1558 = Build Path(base path=w3430, name or relative path=w3434) -> (appended path=w3432:path)
            n1559 = while {
              tunnel: w3434 -> [w3503]
              tunnel: w3430 -> [w3500]
              shift-right: [w3502] -> w3433
              shift-left: w3432 -> [w3501]
              shift-right: [w3498] -> w3428
              shift-left: w3429 -> [w3499]
              tunnel: w3491 -> [w3504]
              tunnel: [w3505] -> w3492
              stop <- w3497 continue-if-true
              n1560 = call <vilib>:"Check if File or Folder Exists.vi"("error in (no error)"=w3504, "path"=w3501) -> ("error out"=w3505:errorcluster, "file or folder exists?"=w3497:bool)  [unwired: 7 in, 1 out]
              n1561 = case shown="True" w3497 {
                tunnel: w3503 -> [_ w3517]
                tunnel: w3499 -> [_ w3509]
                tunnel: [w3507 w3514] -> w3502
                tunnel: w3501 -> [w3507 _]
                tunnel: w3500 -> [_ w3515]
                tunnel: [1 w3508] -> w3498
                frame False {
                }
                frame True {
                  w3510 = ".docx" ("search string")
                  n1562 = Search and Replace String(input string=w3517, search string=w3510) -> (result string=w3516:string)  [unwired: 6 in, 3 out]
                  n1563 = Number To Decimal String(number=w3509) -> (decimal integer string=w3512:string)  [unwired: 1 in]
                  n1564 = call <vilib>:"Space Constant.vi"() -> ("String"=w3511:string)
                  n1565 = Concatenate Strings(w3516, w3511, w3512, w3510) -> (w3513:string)
                  n1566 = Build Path(base path=w3515, name or relative path=w3513) -> (appended path=w3514:path)
                  n1567 = Increment(x=w3509) -> (x+1=w3508:i32)
                }
              }
            }
            n1568 = call "HeaderuRayon.vi"("Tester Software Ver"=w3447, "UUTHeader"=w3445, "UUT"=w3465, "S/N"=w3462, "VR"=w3467, "Oper."=w3466) -> ("HEADER1"=w3494:string)
            n1569 = Open/Create/Replace File(file path (use dialog)=w3433, error in=w3492, operation (0:open)=T20."create") -> (error out=w3477:errorcluster)  [unwired: 3 in, 2 out]
            n1570 = property class="Tbl (strict)"(reference=w3495, error in=w3477) -> (error out=w3469:errorcluster, "Value"=w3496:string[][])  [unwired: 1 out]
            n1571 = call "MarvinReport.vi"("HEADER1"=w3494, "ATR Or"=w3495, "Steps   pfull"=w3496, "Footer UUT"=w3464, "pageNum"=3, "FILE NAME"=w3434, "Report Folder"=w3433, "error in (no error)"=w3469, "REV"=w3459, "Test-Conductor"=w3466) -> ("error out"=w3470:errorcluster)  [unwired: 4 in, 1 out]
            n1572 = Select(t=T12."MainProgram", s=w3435, f=T12."Stop") -> (s? t:f=w3436:T12)
          }
          event "Help Button": Value Change {
            n1573 = event-data() -> ()  [unwired: 1 in, 6 out]
            n1574 = vi-ref "Help.vi"() -> (w3573:refnum<vi>)
            n1575 = invoke class="VI" method="FP.Open"(reference=w3573, error in=w3571, "Activate"=TRUE ("Activate?"), "State"=T18."Standard") -> (error out=w3572:errorcluster)  [unwired: 1 in, 4 out]
            n1576 = call "Help.vi"("error in"=w3572) -> ("error out"=w3564:errorcluster)  [unwired: 7 in]
            n1577 = property on="Help Button" class="Bool (strict)"(error in=w3564, "Value"=FALSE ("Help Button")) -> ()  [unwired: 1 in, 2 out]
          }
          event "Serial Com": Value Change {
            n1578 = event-data() -> ()  [unwired: 1 in, 6 out]
            n1579 = property on="Serial Com" class="Bool"(error in=w3582, "Visible"=FALSE) -> (error out=w3586:errorcluster)  [unwired: 1 in, 1 out]
            n1580 = property on="VISA resource name" class="VISAName"(error in=w3586, "Visible"=TRUE) -> (error out=w3583:errorcluster)  [unwired: 1 in, 1 out]
          }
          event "VISA resource name": Value Change {
            w3589 = T13."Enabled" ("Disabled")
            n1581 = event-data() -> ()  [unwired: 1 in, 6 out]
            n1582 = control-ref of="This VI"() -> (w3603:refnum<vi>)
            n1583 = property on="Pannel User Message" class="Str"(error in=w3592, "Value"="Serial conection in process" ("Pannel User Message")) -> ()  [unwired: 1 in, 2 out]
            n1584 = call "Serial InitMarvin.vi"("error in (no error)"=w3592, "VI reference (current VI)"=w3603, "VISA Refnum in"="VISA resource name") -> ("error out"=w3610:errorcluster, "Boolean"=w3591:bool)  [unwired: 7 in]
            n1585 = property on="Serial" class="Bool (strict)"(error in=w3610, "Value"=w3591) -> (error out=w3607:errorcluster)  [unwired: 1 in, 1 out]
            n1586 = property on="VISA resource name" class="VISAName"(error in=w3607, "Visible"=FALSE) -> (error out=w3606:errorcluster)  [unwired: 1 in, 1 out]
            n1587 = property on="Serial Com" class="Bool"(error in=w3606, "Visible"=TRUE) -> (error out=w3602:errorcluster)  [unwired: 1 in, 1 out]
            n1588 = case shown="True" w3591 {
              tunnel: w3602 -> [w3612 w3628]
              tunnel: [w3612 w3622] -> w3601
              tunnel: "VISA resource name" -> [_ w3624]
              frame False {
              }
              frame True {
                n1589 = call "SerialMarvinMod.vi"("error in (no error)"=w3628, "Clear Log"=FALSE, "write buffer"="SN\r\n", "VISA resource name"=w3624) -> ("error out"=w3623:errorcluster, "read buffer"=→"Curret SN":string)  [unwired: 6 in]
                n1590 = call "SerialMarvinMod.vi"("error in (no error)"=w3623, "Clear Log"=FALSE, "write buffer"="AO[1]\r\n", "VISA resource name"=w3624) -> ("error out"=w3622:errorcluster, "read buffer"=w3615:string)  [unwired: 6 in]
                n1591 = control-ref of="ATR"() -> (w3613:refnum<vi>)
                n1592 = property class="Tbl (strict)"(reference=w3613) -> ("Value"=w3618:string[][])  [unwired: 1 in, 2 out]
                n1593 = Index Array(array=w3618, index (col)=0 ("disabled index (col)")) -> (element=w3620:string[])  [unwired: 1 in]
                n1594 = call "Find_Number_LineMARVIN.vi"("Test Paragraph"="7.5.5.1", "Row Headers[]"=w3620) -> ("Line number"=w3617:i32)  [unwired: 3 in, 3 out]
                n1595 = Replace Array Subset(array=w3618, new element=w3615, index (row)=w3617, index (col)=5 ("disabled index (col)")) -> (w3614:string[][])
                n1596 = property class="Tbl (strict)"(reference=w3613, "Value"=w3614) -> ()  [unwired: 1 in, 2 out]
              }
            }
            n1597 = call <vilib>:"Clear Errors.vi"("error in (no error)"=w3601) -> ("error out"=w3611:errorcluster)  [unwired: 5 in, 1 out]
            n1598 = case shown="True" w3591 {
              tunnel: w3611 -> [w3700 w3704]
              tunnel: [w3700 w3703] -> w3595
              tunnel: "VISA resource name" -> [w3699 w3702]
              tunnel: [w3699 w3701] -> w3596
              frame False {
              }
              frame True {
                n1599 = VISA Flush I/O Buffer(VISA resource name=w3702, error in (no error)=w3704) -> (VISA resource name out=w3701:refnum<visa-resource-name>, error out=w3703:errorcluster)  [unwired: 1 in]
              }
            }
            n1600 = case shown="True" w3591 {
              tunnel: w3595 -> [w3632 w3635]
              tunnel: [w3632 w3634] -> w3594
              tunnel: [FALSE ("Yes") w3633] -> w3593
              frame False {
              }
              frame True {
                n1601 = call "Display Message to User2"("error in (no error)"=w3635) -> ("error out"=w3634:errorcluster, "Yes"=w3633:bool)  [unwired: 9 in]
              }
            }
            n1602 = case shown="True" w3593 {
              tunnel: w3594 -> [w3636 w3638]
              tunnel: [w3636 w3642] -> w3588
              frame False {
              }
              frame True {
                w3639 = T13."Disabled and Grayed Out" ("Disabled")
                n1603 = property on="Serial" class="Bool (strict)"() -> ("Value"=w3640:bool)  [unwired: 2 in, 2 out]
                n1604 = property on="VISA resource name" class="VISAName"() -> ("Value"=w3641:refnum<visa-resource-name>)  [unwired: 2 in, 2 out]
                n1605 = case shown="True" w3640 {
                  selector: w3640 -> [_ w3683]
                  tunnel: w3638 -> [w3644 w3673]
                  tunnel: w3641 -> [_ w3653]
                  tunnel: [w3643 w3652] -> w3642
                  frame False {
                    n1606 = call "Display Message to User3"("error in (no error)"=w3644) -> ("error out"=w3643:errorcluster)  [unwired: 9 in, 1 out]
                  }
                  frame True {
                    w3660 = "Set parameters in process..." ("Strin")
                    n1607 = control-ref of="VISA resource name out"() -> (w3682:refnum<vi>)
                    n1608 = control-ref of="Stop Button"() -> (w3658:refnum<vi>)
                    n1609 = control-ref of="Motor Speed RPM"() -> (w3647:refnum<vi>)
                    n1610 = control-ref of="Pannel User Message"() -> (w3659:refnum<vi>)
                    n1611 = property on="UUT" class="Str"(error in=w3673) -> (error out=w3668:errorcluster, "Value"=w3672:string)  [unwired: 1 in, 1 out]
                    n1612 = Equal?(x=w3672, y="EBAY") -> (x = y?=w3670:bool)
                    n1613 = case shown="False" w3670 {
                      tunnel: [w3688 u16 95 ("Param to Set in")] -> w3669
                      tunnel: w3668 -> [w3685 w3697]
                      tunnel: [w3684 w3697] -> w3667
                      frame False {
                        n1614 = while {
                          tunnel: [w3692] -> w3686
                          tunnel: w3685 -> [w3691]
                          tunnel: [w3690] -> w3684
                          stop <- w3696 stop-if-true
                          n1615 = call "AHU #"("error in (no error)"=w3691) -> ("47"=w3692:bool, "63"=w3695:bool, "OK"=w3693:bool, "error out"=w3690:errorcluster)  [unwired: 15 in]
                          n1616 = Exclusive Or(1:w3695, 2:w3692) -> (0:w3694:bool)
                          n1617 = And(x=w3694, y=w3693) -> (x .and. y?=w3696:bool)
                        }
                        n1618 = Select(t=u16 47 ("Param to Set in"), s=w3686, f=u16 63 ("Param to Set in")) -> (s? t:f=w3688:u16)
                      }
                      frame True {
                      }
                    }
                    n1619 = property class="VISAName"(reference=w3682, error in=w3667) -> (error out=w3679:errorcluster, "Value"=w3657:refnum<visa-resource-name>)  [unwired: 1 out]
                    n1620 = Byte Array To String(unsigned byte array=u8[] [75, 0, 4, 2, 0, 0, 0, 0] ("appended array")) -> (string=w3681:string)
                    n1621 = VISA Write(VISA resource name=w3657, write buffer=w3681, error in (no error)=w3679) -> (VISA resource name out=w3675:refnum<visa-resource-name>, error out=w3666:errorcluster)  [unwired: 1 out]
                    n1622 = call "Write panel message (SubVI).vi"(4:"rpm"=w3647, 5:"rpm"=FALSE ("rpm"), "PrintTime"=FALSE, "Stop"=w3658, "error in (no error)"=w3666, "Time to wait"=0.2, "Strin"=w3660, "String in"=w3659) -> ("error out"=w3665:errorcluster)  [unwired: 3 in]
                    n1623 = call "SetParam.vi"("RS"=w3683, "error in (no error)"=w3665, "Param to Set in"=w3669, "Visa"=w3653) -> ("error out"=w3664:errorcluster)  [unwired: 7 in]
                    n1624 = Byte Array To String(unsigned byte array=u8[] [75, 0, 4, 2, 0, 0, 0, 0] ("appended array")) -> (string=w3677:string)
                    n1625 = Byte Array To String(unsigned byte array=u8[] [75, 0, 4, 2, 0, 0, 16, 0] ("appended array")) -> (string=w3655:string)
                    n1626 = VISA Write(VISA resource name=w3657, write buffer=w3655, error in (no error)=w3664) -> (error out=w3663:errorcluster)  [unwired: 2 out]
                    n1627 = call "Write panel message (SubVI).vi"("rpm"=w3647, "Stop"=w3658, "error in (no error)"=w3663, "Time to wait"=15.0, "Strin"=w3660, "String in"=w3659) -> ("error out"=w3662:errorcluster)  [unwired: 5 in]
                    n1628 = call <vilib>:"Clear Errors.vi"("error in (no error)"=w3662) -> ("error out"=w3676:errorcluster)  [unwired: 5 in, 1 out]
                    n1629 = VISA Write(VISA resource name=w3675, write buffer=w3677, error in (no error)=w3676) -> (error out=w3654:errorcluster)  [unwired: 2 out]
                    n1630 = call "Serial.vi"("error in (no error)"=w3654, "Clear Log"=FALSE, "write buffer"="AO[1]\r\n", "VISA resource name"=w3653) -> ("error out"=w3652:errorcluster, "read buffer"=w3649:string)  [unwired: 5 in, 1 out]
                    n1631 = Equal?(x=w3649, y="") -> ()  [unwired: 1 out]
                  }
                }
                n1632 = property on="Start" class="Bool (strict)"(error in=w3638, "DisabledEnum"=w3639) -> (error out=w3637:errorcluster)  [unwired: 1 in, 1 out]
                n1633 = property on="Report" class="Bool (strict)"(error in=w3637, "DisabledEnum"=w3639) -> ()  [unwired: 1 in, 2 out]
              }
            }
            n1634 = property on="Start" class="Bool (strict)"(error in=w3588, "DisabledEnum"=w3589) -> (error out=w3587:errorcluster)  [unwired: 1 in, 1 out]
            n1635 = property on="Report" class="Bool (strict)"(error in=w3587, "DisabledEnum"=w3589) -> ()  [unwired: 1 in, 2 out]
          }
          event "Refresh Button": Value Change {
            n1636 = event-data() -> ()  [unwired: 1 in, 6 out]
            n1637 = property on="Refresh Button" class="Bool (strict)"("Value"=FALSE ("Refresh Button")) -> ()  [unwired: 2 in, 2 out]
          }
          event Panel Close? {
            w3714 = TRUE ("Stop Button")
            n1638 = event-data() -> ("VIRef"=w3716:refnum<vi>)  [unwired: 1 in, 3 out]
            n1639 = Close Reference(reference=w3716) -> ()  [unwired: 1 in, 1 out]
            n1640 = property on="Stop Button" class="Bool (strict)"(error in=w3715, "Val(Sgnl)"=w3714, "Value"=w3714) -> ()  [unwired: 1 in, 2 out]
            n1641 = event-data("Discard?"=TRUE) -> ()  [unwired: 1 in, 1 out]
            "ClosePanel" <- w3714
          }
          event "Settings": Value Change {
            n1642 = event-data() -> ()  [unwired: 1 in, 6 out]
            n1643 = disable-structure shown="Enabled" {
              disable-tunnel: [w3737 w3740] -> w3725
              disable-tunnel: [w3736 w3740] -> w3724
              frame Disabled {
                n1644 = call "Temperature calibration settings"() -> ("Password"=w3739:dbl, "OK"=w3737:bool)  [unwired: 17 in, 1 out]
                n1645 = Equal?(x=w3739, y=1234.0) -> (x = y?=w3736:bool)
              }
              frame Enabled {
                w3740 = TRUE ("OK")
              }
            }
            n1646 = property on="Serial" class="Bool (strict)"(error in=w3730) -> (error out=w3728:errorcluster, "Value"=w3731:bool)  [unwired: 1 in, 1 out]
            n1647 = Compound Arithmetic op=AND(w3731, w3725, w3724) -> (w3726:bool)
            n1648 = case shown="True" w3726 {
              tunnel: w3728 -> [w3742 w3747]
              tunnel: w3729 -> [_ w3746]
              tunnel: [w3741 w3745] -> w3727
              frame False {
                n1649 = flat-sequence {
                  tunnel: w3742 -> [w3743]
                  tunnel: [w3743] -> w3741
                  frame #0 {
                    n1650 = One Button Dialog(message="Please establish RS connection.") -> ()  [unwired: 1 in, 1 out]
                  }
                }
              }
              frame True {
                n1651 = call "Calibration (SubVI).vi"("error constant"=w3747) -> ("error constant 2"=w3749:errorcluster, "Val"=w3757:dbl[], "K"=w3758:u32[])  [unwired: 8 in]
                n1652 = Concatenate Strings("EP=1\r\nAO" ("string"), "[", "1" ("string"), "]=0", "\r\n" ("write buffer")) -> (w3756:string)
                n1653 = call "SerialMarvinMod.vi"("error in (no error)"=w3749, "Clear Log"=FALSE, "write buffer"=w3756, "VISA resource name"=w3746) -> ("error out"=w3748:errorcluster)  [unwired: 6 in, 1 out]
                n1654 = for {
                  tunnel: w3758 -> [w3808] mode=indexing
                  tunnel: w3746 -> [w3803]
                  tunnel: w3757 -> [w3801] mode=indexing
                  tunnel: [w3792] -> w3791 mode=indexing
                  tunnel: [w3800] -> w3759
                  tunnel: w3748 -> [w3798]
                  tunnel: [w3796] -> w3765
                  n1655 = control-ref of="VISA resource name out"() -> (w3805:refnum<vi>)
                  n1656 = To Unsigned Long Integer(number=w3808) -> (unsigned 32bit integer=w3810:u32)
                  n1657 = Split Number(x=w3810) -> (hi(x)=w3815:u16, lo(x)=w3816:u16)
                  n1658 = Split Number(x=w3816) -> (hi(x)=w3814:u8, lo(x)=w3813:u8)
                  n1659 = Split Number(x=w3815) -> (hi(x)=w3812:u8, lo(x)=w3811:u8)
                  n1660 = property class="VISAName"(reference=w3805, error in=w3798) -> (error out=w3799:errorcluster, "Value"=w3796:refnum<visa-resource-name>)  [unwired: 1 out]
                  n1661 = Build Array(u8 75, u8 0 ("element"), u8 4 ("Length"), u8 2, w3813, w3814, w3811, w3812) -> (w3807:u8[])
                  n1662 = Byte Array To String(unsigned byte array=w3807) -> (string=w3806:string)
                  n1663 = Concatenate Strings("TA" ("string"), "[", "5" ("string"), "]", "\r\n" ("write buffer")) -> (w3820:string)
                  n1664 = VISA Write(VISA resource name=w3796, write buffer=w3806, error in (no error)=w3799) -> (error out=w3802:errorcluster)  [unwired: 2 out]
                  n1665 = call "Wait_Sec.vi"("Delay Time (sec)"=2.0, "error out"=w3802) -> ("error in"=w3794:errorcluster)  [unwired: 2 in]
                  n1666 = call "SerialMarvinMod.vi"("error in (no error)"=w3794, "Clear Log"=FALSE, "write buffer"=w3820, "VISA resource name"=w3803) -> ("error out"=w3800:errorcluster, "read buffer"=w3797:string)  [unwired: 6 in]
                  n1667 = Fract/Exp String To Number(string=w3797) -> (number=w3795:dbl)  [unwired: 3 in, 1 out]
                  n1668 = Subtract(x=w3795, y=w3801) -> (x-y=w3792:dbl)
                }
                n1669 = To Unsigned Long Integer(number=u32 0) -> (unsigned 32bit integer=w3777:u32)
                n1670 = Split Number(x=w3777) -> (hi(x)=w3783:u16, lo(x)=w3784:u16)
                n1671 = Split Number(x=w3784) -> (hi(x)=w3782:u8, lo(x)=w3781:u8)
                n1672 = Split Number(x=w3783) -> (hi(x)=w3780:u8, lo(x)=w3779:u8)
                n1673 = Build Array(u8 75, u8 0 ("element"), u8 4 ("Length"), u8 2, w3781, w3782, w3779, w3780) -> (w3775:u8[])
                n1674 = Byte Array To String(unsigned byte array=w3775) -> (string=w3788:string)
                n1675 = Add Array Elements(numeric array=w3791) -> (sum=w3790:dbl)
                n1676 = Divide(x=w3790, y=4.0) -> (x/y=w3760:dbl)
                n1677 = Number To Fractional String(number=w3760, precision (6)=i16 4) -> (F-format string=w3761:string)  [unwired: 2 in]
                "Cal Value" <- w3761
                n1678 = Concatenate Strings("EP=1\r\nAO" ("string"), "[", "1" ("string"), "]=", w3761, "\r\n" ("write buffer")) -> (w3769:string)
                n1679 = VISA Write(VISA resource name=w3765, write buffer=w3788, error in (no error)=w3759) -> (error out=w3766:errorcluster)  [unwired: 2 out]
                n1680 = call "SerialMarvinMod.vi"("error in (no error)"=w3766, "Clear Log"=FALSE, "write buffer"=w3769, "VISA resource name"=w3746) -> ("error out"=w3764:errorcluster)  [unwired: 6 in, 1 out]
                n1681 = call "SerialMarvinMod.vi"("error in (no error)"=w3764, "write buffer"="AO[1]\r\n", "VISA resource name"=w3746) -> ("error out"=w3745:errorcluster, "read buffer"=w3762:string)  [unwired: 7 in]
                n1682 = Equal?(x=w3761, y=w3762) -> ()  [unwired: 1 out]
              }
            }
          }
        }
        n1683 = Equal?(x="", y=w2814) -> (x = y?=w2816:bool)
        n1684 = Select(t=w2815, s=w2816, f=w2814) -> (s? t:f=w2813:string)
      }
      frame "Initialize" {
        w3831 = T13."Enabled" ("Disabled")
        w3840 = refnum<visa-resource-name> "COM1" ("VISA resource name")
        w3826 = FALSE ("Visible")
        n1685 = disable-structure shown="Disabled" {
          frame Disabled {
            n1686 = local write "UUT"("" ("UUT")) -> ()
          }
          frame Enabled {
          }
        }
        n1687 = property on="Serial Com" class="Bool"(error in=errorcluster {"status"=FALSE, "code"=0, "source"=""} ("error out"), "Visible"=TRUE) -> (error out=w3844:errorcluster)  [unwired: 1 in, 1 out]
        n1688 = property on="VISA resource name" class="VISAName"(error in=w3844, "Visible"=w3826, "Value"=w3840) -> (error out=w3832:errorcluster)  [unwired: 1 in, 1 out]
        n1689 = property on="Stop Burn-in" class="Bool"(error in=w3832, "Visible"=w3826) -> (error out=w3827:errorcluster)  [unwired: 1 in, 1 out]
        n1690 = flat-sequence {
          tunnel: w3827 -> [w3848]
          tunnel: [w3847] -> w3838
          tunnel: [w3850] -> w3837
          tunnel: w3838 -> [w3850]
          tunnel: [w3863] -> w3836
          tunnel: w3837 -> [w3864]
          tunnel: [w3864] -> w3829
          frame #0 {
            n1691 = control-ref of="This VI"() -> (w3849:refnum<vi>)
            n1692 = invoke class="VI" method="Default Vals.Reinit All"(reference=w3849, error in=w3848) -> (error out=w3847:errorcluster)  [unwired: 1 in, 2 out]
          }
          frame #1 {
            w3854 = u32 4294967295  # AccMask
            w3853 = T6 0 items=["使用Flash参数", "使用界面设置参数"] ("InitFlag")
            w3851 = T8 0 items=["normal operation", "Listen-only mode", "test mode"]  # Mode
            w3852 = T7 3 items=["接收所有类型"=1, "只接收标准帧"=2, "只接收扩展帧"=3] ("Fliter")
            w3858 = u8 10 items=["5k bps"=1, "10k bps"=2, "20k bps"=3, "40k bps"=4, "50k bps"=5, "80k bps"=6, "100k bps"=7, "125k bps"=8, "200k bps"=9, "250k bps"=10, "400k bps"=11, "500k bps"=12, "666k bps"=13, "800k bps"=14, "1000k bps"=15, "33.33k bps"=16, "66.66k bps"=17, "83.33k bps"=18]  # kBaudRate
            w3855 = u32 0  # AccCode
            w3856 = T4 4 items=["USB-CAN"=3, "USB-CAN2"=4] ("DevType")
            w3857 = T9 {"DevType"=3, "DevIndex"=0, "CanIndex"=0, "VCI_INIT_CONFIG"={"AccCode"=0, "AccMask"=0, "InitFlag"=1, "Fliter"=7, "Timing0"=0, "Timing1"=0, "Mode"=0}}  # Config
            # "CANalystII"
            n1693 = call "Demo_GetT0T1.vi"("kBaudRate"=w3858) -> ("Timing0"=w3860:u8, "Timing1"=w3861:u8)
            n1694 = Bundle By Name(cluster=w3857, "DevType"=w3856, "CanIndex"="Channel 2", "VCI_INIT_CONFIG.AccCode"=w3855, "VCI_INIT_CONFIG.AccMask"=w3854, "VCI_INIT_CONFIG.InitFlag"=w3853, "VCI_INIT_CONFIG.Fliter"=w3852, "VCI_INIT_CONFIG.Timing0"=w3860, "VCI_INIT_CONFIG.Timing1"=w3861, "VCI_INIT_CONFIG.Mode"=w3851) -> (→"Config_CANAT":T9)
          }
          frame #2 {
            w3865 = u16 284 items=["1M"=20, "500K"=28, "250K"=284, "125K"=796, "100K"=17199, "50K"=18223, "20K"=21295, "10K"=26415, "5K"=32639] ("baud in")
            n1695 = control-ref of="Config_CANAT"() -> (w3863:refnum<vi>)
            n1696 = call "ChangeCANBaud.vi"("baud in"=w3865, "reference"=w3863) -> ()
            n1697 = call "InitCAN_ATII.vi"("Config"=w3863) -> ("Sts"=→"CAN Status":bool)
          }
        }
        n1698 = Wait (ms)(milliseconds to wait=u32 150) -> ()  [unwired: 1 out]
        n1699 = property on="Start" class="Bool (strict)"(error in=w3829, "DisabledEnum"=w3831) -> (error out=w3830:errorcluster)  [unwired: 1 in, 1 out]
        n1700 = property on="Report" class="Bool (strict)"(error in=w3830, "DisabledEnum"=w3831) -> ()  [unwired: 1 in, 2 out]
        "Serial" <- FALSE ("Serial Status")
      }
    }
    "Pannel User Message" <- w2495
  }
